vi "Drift Verification Konfig.vi"() -> ()   [LabVIEW 2020, in "EPA 1065.lvlib" / "Gas Analyzer Drift 1065-550.lvlib"]
uses:
  Gas Analyzer Drift 1065-550.lvlib
  Spaninlet Cluster.ctl
  Seiten/System Einstellungen V2/Konfig Gasflasche.ctl
  Seiten/System Einstellungen V2/Analysatoren.ctl
  Seiten/System Einstellungen V2/Gasflasche Auswahl.ctl
  T90 1065-308/Modus.ctl
  Komponentencluster.ctl
  Komponentenauswahl.ctl
  Drifttabelle.ctl
  Konfig Daten Drift Verification.ctl
  Anzeigecluster.ctl
  Chiller NO2 1065-376/Aktion FGV Drift Daten.ctl
  Aktion FGV Komponentenreferenz verwalten.ctl
  Sprachverwaltung/FGV Aktion Tabelle zerlegen.ctl
  Aktion Automatischer Ablauf Zustandsautomat.ctl
  Seiten/System Einstellungen V2/Aktion FGV Gasbottledefinition.ctl
  Seiten/FT-IR/FGV FT-IR Gasliste Aktionen.ctl
  Allgemeine VIs/Aktion Wertaenderung Gasliste.ctl
  Allgemeine VIs/Aktion Test Status.ctl
  Funktionstasten/Funktionstasten-Aktion.ctl
  Funktionstasten/Zustaende.ctl
  Allgemein/allgemeine Sub-VIs.lvlib
  Seiten/FT-IR/FT-IR.lvlib
  Funktionstasten/Funktionstasten.lvlib
  EPA 1065.lvlib
  Sprachverwaltung/Sprachverwaltung.lvlib
  Seiten/System Einstellungen V2/System Einstellungen V2.lvlib
  T90 1065-308/T90 Test 1065-308.lvlib
panel:
  in  "Systemeinstellung":bool
  in  "Gasliste geändert":bool
  in  "Registerkarte":T1(tab)
  in  "Pre Drift entsperren":bool caption="Test Start"
  in  "Pre Drift sperren":bool caption="Test Start"
  in  "Drift Konfig Daten":T2={"Bearbeiter:"="", "Pfad:"=path "D:/IAG_Data/Log", "Textname:"="", "CG Aufschaltzeit:"=120.0, "N2 Aufschaltzeit:"=120.0} caption="T90 Konfig Daten" {"N2 Aufschaltzeit:" min=10.0; "CG Aufschaltzeit:" min=10.0}
  in  "Speichern":bool
  in  "SpanRegister":T3(tab)
  in  "Span 1":T4={"Span Inlet Active"=FALSE, "Analysator"="FT-IR", "Konfig Gasflasche"=FALSE, "Gasflasche"=0, "Gasflaschen Nr.:"="", "Ablaufdatum"=timestamp(0 s since 1904-01-01), "Modus"=0, "Komponenten"={"Komponente 1"={"Komponente:"=0, "Konzentration IST"=0.0, "Einheit"=enum."ppm", "Genauigkeit"=0.0}, "Komponente 2"={"Komponente:"=0, "Konzentration IST"=0.0, "Einheit"=enum."ppm", "Genauigkeit"=0.0}, "Komponente 3"={"Komponente:"=0, "Konzentration IST"=0.0, "Einheit"=enum."ppm", "Genauigkeit"=0.0}, "Komponente 4"={"Komponente:"=0, "Konzentration IST"=0.0, "Einheit"=enum."ppm", "Genauigkeit"=0.0}, "Komponente 5"={"Komponente:"=0, "Konzentration IST"=0.0, "Einheit"=enum."ppm", "Genauigkeit"=0.0}}} {"Komponenten"."Komponente 5"."Komponente:" items=["---", "NO (3000) LP 191C", "NO2 (150) LP 191C (1of2)", "NO2 (2000) LP 191C (2of2)", "N2O (300) LP 191C (1of2)", "NH3 (300) LP 191C (1of2)", "NH3 (900,3000) LP 191C (2of2)", "HNCO (400) 191C", "H2O% (30) LP 191C", "Formaldehyde (70,500) LP 191C", "CO2 low% (4) LP 191C (2of2)", "CO2% (20) LP 191C (1of2)", "CO (700) LP 191C (1of3)", "CO% (1) LP 191C (2of3)", "Propylene (1000) LP 191C", "Aromatic HC C7 (500) LP 191C", "Ethylene (1000) LP 191C", "CH4 (250) LP 191C (1of2)", "CH4 (5000) LP 191C (2of2)", "Ethane (1000) LP 191C", "Acetylene (1000) LP 191C", "HNO2 (20) 191C", "MeOH (1000) 191C", "CO% (10) LP 191C (3of3)", "Formic Acid (100) 191C", "SO2 (500) LP 191C", "Acetaldehyde (1000) LP 191C", "COS (100) LP 191C", "1,3 butadiene (100) LP 191C", "Oil as Octane (200) LP 191C", "N2O (1000) LP 191C (2of2)", "Propane (200) LP 191C", "NO2 autorange (2000)", "CO autorange (100000)", "CH4 autorange (5000)", "NH3 autorange (3000)", "NOx autorange (3000)", "HCD (10000)", "NMHCD (10000)", "CO2% autorange (20)", "H2Oppm (300000)", "N2O autorange (1000)", "NMNEHCD (3000)", "Temp. Gascell", "Pressure Gascell", "sBeam@2500", "Temp. HL to FT-IR", "Temp. HL Extern SP1", "Outlet Temp FT-IR", "Temp. Cabinet", "Constant 0", "Constant 50", "Constant 100", "AK DUMMY"]; "Komponenten"."Komponente 5"."Konzentration IST" format="%#.4f"; "Komponenten"."Komponente 5"."Genauigkeit" format="%#.1f"; "Komponenten"."Komponente 4"."Komponente:" items=["---", "NO (3000) LP 191C", "NO2 (150) LP 191C (1of2)", "NO2 (2000) LP 191C (2of2)", "N2O (300) LP 191C (1of2)", "NH3 (300) LP 191C (1of2)", "NH3 (900,3000) LP 191C (2of2)", "HNCO (400) 191C", "H2O% (30) LP 191C", "Formaldehyde (70,500) LP 191C", "CO2 low% (4) LP 191C (2of2)", "CO2% (20) LP 191C (1of2)", "CO (700) LP 191C (1of3)", "CO% (1) LP 191C (2of3)", "Propylene (1000) LP 191C", "Aromatic HC C7 (500) LP 191C", "Ethylene (1000) LP 191C", "CH4 (250) LP 191C (1of2)", "CH4 (5000) LP 191C (2of2)", "Ethane (1000) LP 191C", "Acetylene (1000) LP 191C", "HNO2 (20) 191C", "MeOH (1000) 191C", "CO% (10) LP 191C (3of3)", "Formic Acid (100) 191C", "SO2 (500) LP 191C", "Acetaldehyde (1000) LP 191C", "COS (100) LP 191C", "1,3 butadiene (100) LP 191C", "Oil as Octane (200) LP 191C", "N2O (1000) LP 191C (2of2)", "Propane (200) LP 191C", "NO2 autorange (2000)", "CO autorange (100000)", "CH4 autorange (5000)", "NH3 autorange (3000)", "NOx autorange (3000)", "HCD (10000)", "NMHCD (10000)", "CO2% autorange (20)", "H2Oppm (300000)", "N2O autorange (1000)", "NMNEHCD (3000)", "Temp. Gascell", "Pressure Gascell", "sBeam@2500", "Temp. HL to FT-IR", "Temp. HL Extern SP1", "Outlet Temp FT-IR", "Temp. Cabinet", "Constant 0", "Constant 50", "Constant 100", "AK DUMMY"]; "Komponenten"."Komponente 4"."Konzentration IST" format="%#.4f"; "Komponenten"."Komponente 4"."Genauigkeit" format="%#.1f"; "Komponenten"."Komponente 3"."Komponente:" items=["---", "NO (3000) LP 191C", "NO2 (150) LP 191C (1of2)", "NO2 (2000) LP 191C (2of2)", "N2O (300) LP 191C (1of2)", "NH3 (300) LP 191C (1of2)", "NH3 (900,3000) LP 191C (2of2)", "HNCO (400) 191C", "H2O% (30) LP 191C", "Formaldehyde (70,500) LP 191C", "CO2 low% (4) LP 191C (2of2)", "CO2% (20) LP 191C (1of2)", "CO (700) LP 191C (1of3)", "CO% (1) LP 191C (2of3)", "Propylene (1000) LP 191C", "Aromatic HC C7 (500) LP 191C", "Ethylene (1000) LP 191C", "CH4 (250) LP 191C (1of2)", "CH4 (5000) LP 191C (2of2)", "Ethane (1000) LP 191C", "Acetylene (1000) LP 191C", "HNO2 (20) 191C", "MeOH (1000) 191C", "CO% (10) LP 191C (3of3)", "Formic Acid (100) 191C", "SO2 (500) LP 191C", "Acetaldehyde (1000) LP 191C", "COS (100) LP 191C", "1,3 butadiene (100) LP 191C", "Oil as Octane (200) LP 191C", "N2O (1000) LP 191C (2of2)", "Propane (200) LP 191C", "NO2 autorange (2000)", "CO autorange (100000)", "CH4 autorange (5000)", "NH3 autorange (3000)", "NOx autorange (3000)", "HCD (10000)", "NMHCD (10000)", "CO2% autorange (20)", "H2Oppm (300000)", "N2O autorange (1000)", "NMNEHCD (3000)", "Temp. Gascell", "Pressure Gascell", "sBeam@2500", "Temp. HL to FT-IR", "Temp. HL Extern SP1", "Outlet Temp FT-IR", "Temp. Cabinet", "Constant 0", "Constant 50", "Constant 100", "AK DUMMY"]; "Komponenten"."Komponente 3"."Konzentration IST" format="%#.4f"; "Komponenten"."Komponente 3"."Genauigkeit" format="%#.1f"; "Komponenten"."Komponente 2"."Komponente:" items=["---", "NO (3000) LP 191C", "NO2 (150) LP 191C (1of2)", "NO2 (2000) LP 191C (2of2)", "N2O (300) LP 191C (1of2)", "NH3 (300) LP 191C (1of2)", "NH3 (900,3000) LP 191C (2of2)", "HNCO (400) 191C", "H2O% (30) LP 191C", "Formaldehyde (70,500) LP 191C", "CO2 low% (4) LP 191C (2of2)", "CO2% (20) LP 191C (1of2)", "CO (700) LP 191C (1of3)", "CO% (1) LP 191C (2of3)", "Propylene (1000) LP 191C", "Aromatic HC C7 (500) LP 191C", "Ethylene (1000) LP 191C", "CH4 (250) LP 191C (1of2)", "CH4 (5000) LP 191C (2of2)", "Ethane (1000) LP 191C", "Acetylene (1000) LP 191C", "HNO2 (20) 191C", "MeOH (1000) 191C", "CO% (10) LP 191C (3of3)", "Formic Acid (100) 191C", "SO2 (500) LP 191C", "Acetaldehyde (1000) LP 191C", "COS (100) LP 191C", "1,3 butadiene (100) LP 191C", "Oil as Octane (200) LP 191C", "N2O (1000) LP 191C (2of2)", "Propane (200) LP 191C", "NO2 autorange (2000)", "CO autorange (100000)", "CH4 autorange (5000)", "NH3 autorange (3000)", "NOx autorange (3000)", "HCD (10000)", "NMHCD (10000)", "CO2% autorange (20)", "H2Oppm (300000)", "N2O autorange (1000)", "NMNEHCD (3000)", "Temp. Gascell", "Pressure Gascell", "sBeam@2500", "Temp. HL to FT-IR", "Temp. HL Extern SP1", "Outlet Temp FT-IR", "Temp. Cabinet", "Constant 0", "Constant 50", "Constant 100", "AK DUMMY"]; "Komponenten"."Komponente 2"."Konzentration IST" format="%#.4f"; "Komponenten"."Komponente 2"."Genauigkeit" format="%#.1f"; "Komponenten"."Komponente 1"."Komponente:" items=["---", "NO (3000) LP 191C", "NO2 (150) LP 191C (1of2)", "NO2 (2000) LP 191C (2of2)", "N2O (300) LP 191C (1of2)", "NH3 (300) LP 191C (1of2)", "NH3 (900,3000) LP 191C (2of2)", "HNCO (400) 191C", "H2O% (30) LP 191C", "Formaldehyde (70,500) LP 191C", "CO2 low% (4) LP 191C (2of2)", "CO2% (20) LP 191C (1of2)", "CO (700) LP 191C (1of3)", "CO% (1) LP 191C (2of3)", "Propylene (1000) LP 191C", "Aromatic HC C7 (500) LP 191C", "Ethylene (1000) LP 191C", "CH4 (250) LP 191C (1of2)", "CH4 (5000) LP 191C (2of2)", "Ethane (1000) LP 191C", "Acetylene (1000) LP 191C", "HNO2 (20) 191C", "MeOH (1000) 191C", "CO% (10) LP 191C (3of3)", "Formic Acid (100) 191C", "SO2 (500) LP 191C", "Acetaldehyde (1000) LP 191C", "COS (100) LP 191C", "1,3 butadiene (100) LP 191C", "Oil as Octane (200) LP 191C", "N2O (1000) LP 191C (2of2)", "Propane (200) LP 191C", "NO2 autorange (2000)", "CO autorange (100000)", "CH4 autorange (5000)", "NH3 autorange (3000)", "NOx autorange (3000)", "HCD (10000)", "NMHCD (10000)", "CO2% autorange (20)", "H2Oppm (300000)", "N2O autorange (1000)", "NMNEHCD (3000)", "Temp. Gascell", "Pressure Gascell", "sBeam@2500", "Temp. HL to FT-IR", "Temp. HL Extern SP1", "Outlet Temp FT-IR", "Temp. Cabinet", "Constant 0", "Constant 50", "Constant 100", "AK DUMMY"]; "Komponenten"."Komponente 1"."Konzentration IST" format="%#.4f"; "Komponenten"."Komponente 1"."Genauigkeit" format="%#.1f"; "Modus" items=["CG zu PNS", "CG zu Entnahmestelle"]; "Ablaufdatum" format="%<%d.%m.%Y>T"; "Gasflasche" items=["----"=10000, "IAG O2"=0, "IAG C2H2"=1, "IAG C2H4"=2, "IAG NH3 200"=3, "IAG NH3 2000"=4, "IAG NH3 3000"=5, "IAG CO 5%"=6, "IAG Propane 2%"=7, "IAG NO 1000"=8, "IAG SO2"=9, "IAG C3H6"=10, "IAG CO2"=11, "IAG CO"=12, "IAG N2O"=13, "IAG N2O 100"=14, "IAG NO2 1000"=15, "IAG NO2 100"=16, "IAG CH4"=17, "IAG Propane"=18, "IAG NO 5000"=19, "Hansi"=20, "IAG MG"=21]}
  in  "Span 2":T4={"Span Inlet Active"=FALSE, "Analysator"="FT-IR", "Konfig Gasflasche"=FALSE, "Gasflasche"=0, "Gasflaschen Nr.:"="", "Ablaufdatum"=timestamp(0 s since 1904-01-01), "Modus"=0, "Komponenten"={"Komponente 1"={"Komponente:"=0, "Konzentration IST"=0.0, "Einheit"=enum."ppm", "Genauigkeit"=0.0}, "Komponente 2"={"Komponente:"=0, "Konzentration IST"=0.0, "Einheit"=enum."ppm", "Genauigkeit"=0.0}, "Komponente 3"={"Komponente:"=0, "Konzentration IST"=0.0, "Einheit"=enum."ppm", "Genauigkeit"=0.0}, "Komponente 4"={"Komponente:"=0, "Konzentration IST"=0.0, "Einheit"=enum."ppm", "Genauigkeit"=0.0}, "Komponente 5"={"Komponente:"=0, "Konzentration IST"=0.0, "Einheit"=enum."ppm", "Genauigkeit"=0.0}}} {"Komponenten"."Komponente 5"."Komponente:" items=["---", "NO (3000) LP 191C", "NO2 (150) LP 191C (1of2)", "NO2 (2000) LP 191C (2of2)", "N2O (300) LP 191C (1of2)", "NH3 (300) LP 191C (1of2)", "NH3 (900,3000) LP 191C (2of2)", "HNCO (400) 191C", "H2O% (30) LP 191C", "Formaldehyde (70,500) LP 191C", "CO2 low% (4) LP 191C (2of2)", "CO2% (20) LP 191C (1of2)", "CO (700) LP 191C (1of3)", "CO% (1) LP 191C (2of3)", "Propylene (1000) LP 191C", "Aromatic HC C7 (500) LP 191C", "Ethylene (1000) LP 191C", "CH4 (250) LP 191C (1of2)", "CH4 (5000) LP 191C (2of2)", "Ethane (1000) LP 191C", "Acetylene (1000) LP 191C", "HNO2 (20) 191C", "MeOH (1000) 191C", "CO% (10) LP 191C (3of3)", "Formic Acid (100) 191C", "SO2 (500) LP 191C", "Acetaldehyde (1000) LP 191C", "COS (100) LP 191C", "1,3 butadiene (100) LP 191C", "Oil as Octane (200) LP 191C", "N2O (1000) LP 191C (2of2)", "Propane (200) LP 191C", "NO2 autorange (2000)", "CO autorange (100000)", "CH4 autorange (5000)", "NH3 autorange (3000)", "NOx autorange (3000)", "HCD (10000)", "NMHCD (10000)", "CO2% autorange (20)", "H2Oppm (300000)", "N2O autorange (1000)", "NMNEHCD (3000)", "Temp. Gascell", "Pressure Gascell", "sBeam@2500", "Temp. HL to FT-IR", "Temp. HL Extern SP1", "Outlet Temp FT-IR", "Temp. Cabinet", "Constant 0", "Constant 50", "Constant 100", "AK DUMMY"]; "Komponenten"."Komponente 5"."Konzentration IST" format="%#.4f"; "Komponenten"."Komponente 5"."Genauigkeit" format="%#.1f"; "Komponenten"."Komponente 4"."Komponente:" items=["---", "NO (3000) LP 191C", "NO2 (150) LP 191C (1of2)", "NO2 (2000) LP 191C (2of2)", "N2O (300) LP 191C (1of2)", "NH3 (300) LP 191C (1of2)", "NH3 (900,3000) LP 191C (2of2)", "HNCO (400) 191C", "H2O% (30) LP 191C", "Formaldehyde (70,500) LP 191C", "CO2 low% (4) LP 191C (2of2)", "CO2% (20) LP 191C (1of2)", "CO (700) LP 191C (1of3)", "CO% (1) LP 191C (2of3)", "Propylene (1000) LP 191C", "Aromatic HC C7 (500) LP 191C", "Ethylene (1000) LP 191C", "CH4 (250) LP 191C (1of2)", "CH4 (5000) LP 191C (2of2)", "Ethane (1000) LP 191C", "Acetylene (1000) LP 191C", "HNO2 (20) 191C", "MeOH (1000) 191C", "CO% (10) LP 191C (3of3)", "Formic Acid (100) 191C", "SO2 (500) LP 191C", "Acetaldehyde (1000) LP 191C", "COS (100) LP 191C", "1,3 butadiene (100) LP 191C", "Oil as Octane (200) LP 191C", "N2O (1000) LP 191C (2of2)", "Propane (200) LP 191C", "NO2 autorange (2000)", "CO autorange (100000)", "CH4 autorange (5000)", "NH3 autorange (3000)", "NOx autorange (3000)", "HCD (10000)", "NMHCD (10000)", "CO2% autorange (20)", "H2Oppm (300000)", "N2O autorange (1000)", "NMNEHCD (3000)", "Temp. Gascell", "Pressure Gascell", "sBeam@2500", "Temp. HL to FT-IR", "Temp. HL Extern SP1", "Outlet Temp FT-IR", "Temp. Cabinet", "Constant 0", "Constant 50", "Constant 100", "AK DUMMY"]; "Komponenten"."Komponente 4"."Konzentration IST" format="%#.4f"; "Komponenten"."Komponente 4"."Genauigkeit" format="%#.1f"; "Komponenten"."Komponente 3"."Komponente:" items=["---", "NO (3000) LP 191C", "NO2 (150) LP 191C (1of2)", "NO2 (2000) LP 191C (2of2)", "N2O (300) LP 191C (1of2)", "NH3 (300) LP 191C (1of2)", "NH3 (900,3000) LP 191C (2of2)", "HNCO (400) 191C", "H2O% (30) LP 191C", "Formaldehyde (70,500) LP 191C", "CO2 low% (4) LP 191C (2of2)", "CO2% (20) LP 191C (1of2)", "CO (700) LP 191C (1of3)", "CO% (1) LP 191C (2of3)", "Propylene (1000) LP 191C", "Aromatic HC C7 (500) LP 191C", "Ethylene (1000) LP 191C", "CH4 (250) LP 191C (1of2)", "CH4 (5000) LP 191C (2of2)", "Ethane (1000) LP 191C", "Acetylene (1000) LP 191C", "HNO2 (20) 191C", "MeOH (1000) 191C", "CO% (10) LP 191C (3of3)", "Formic Acid (100) 191C", "SO2 (500) LP 191C", "Acetaldehyde (1000) LP 191C", "COS (100) LP 191C", "1,3 butadiene (100) LP 191C", "Oil as Octane (200) LP 191C", "N2O (1000) LP 191C (2of2)", "Propane (200) LP 191C", "NO2 autorange (2000)", "CO autorange (100000)", "CH4 autorange (5000)", "NH3 autorange (3000)", "NOx autorange (3000)", "HCD (10000)", "NMHCD (10000)", "CO2% autorange (20)", "H2Oppm (300000)", "N2O autorange (1000)", "NMNEHCD (3000)", "Temp. Gascell", "Pressure Gascell", "sBeam@2500", "Temp. HL to FT-IR", "Temp. HL Extern SP1", "Outlet Temp FT-IR", "Temp. Cabinet", "Constant 0", "Constant 50", "Constant 100", "AK DUMMY"]; "Komponenten"."Komponente 3"."Konzentration IST" format="%#.4f"; "Komponenten"."Komponente 3"."Genauigkeit" format="%#.1f"; "Komponenten"."Komponente 2"."Komponente:" items=["---", "NO (3000) LP 191C", "NO2 (150) LP 191C (1of2)", "NO2 (2000) LP 191C (2of2)", "N2O (300) LP 191C (1of2)", "NH3 (300) LP 191C (1of2)", "NH3 (900,3000) LP 191C (2of2)", "HNCO (400) 191C", "H2O% (30) LP 191C", "Formaldehyde (70,500) LP 191C", "CO2 low% (4) LP 191C (2of2)", "CO2% (20) LP 191C (1of2)", "CO (700) LP 191C (1of3)", "CO% (1) LP 191C (2of3)", "Propylene (1000) LP 191C", "Aromatic HC C7 (500) LP 191C", "Ethylene (1000) LP 191C", "CH4 (250) LP 191C (1of2)", "CH4 (5000) LP 191C (2of2)", "Ethane (1000) LP 191C", "Acetylene (1000) LP 191C", "HNO2 (20) 191C", "MeOH (1000) 191C", "CO% (10) LP 191C (3of3)", "Formic Acid (100) 191C", "SO2 (500) LP 191C", "Acetaldehyde (1000) LP 191C", "COS (100) LP 191C", "1,3 butadiene (100) LP 191C", "Oil as Octane (200) LP 191C", "N2O (1000) LP 191C (2of2)", "Propane (200) LP 191C", "NO2 autorange (2000)", "CO autorange (100000)", "CH4 autorange (5000)", "NH3 autorange (3000)", "NOx autorange (3000)", "HCD (10000)", "NMHCD (10000)", "CO2% autorange (20)", "H2Oppm (300000)", "N2O autorange (1000)", "NMNEHCD (3000)", "Temp. Gascell", "Pressure Gascell", "sBeam@2500", "Temp. HL to FT-IR", "Temp. HL Extern SP1", "Outlet Temp FT-IR", "Temp. Cabinet", "Constant 0", "Constant 50", "Constant 100", "AK DUMMY"]; "Komponenten"."Komponente 2"."Konzentration IST" format="%#.4f"; "Komponenten"."Komponente 2"."Genauigkeit" format="%#.1f"; "Komponenten"."Komponente 1"."Komponente:" items=["---", "NO (3000) LP 191C", "NO2 (150) LP 191C (1of2)", "NO2 (2000) LP 191C (2of2)", "N2O (300) LP 191C (1of2)", "NH3 (300) LP 191C (1of2)", "NH3 (900,3000) LP 191C (2of2)", "HNCO (400) 191C", "H2O% (30) LP 191C", "Formaldehyde (70,500) LP 191C", "CO2 low% (4) LP 191C (2of2)", "CO2% (20) LP 191C (1of2)", "CO (700) LP 191C (1of3)", "CO% (1) LP 191C (2of3)", "Propylene (1000) LP 191C", "Aromatic HC C7 (500) LP 191C", "Ethylene (1000) LP 191C", "CH4 (250) LP 191C (1of2)", "CH4 (5000) LP 191C (2of2)", "Ethane (1000) LP 191C", "Acetylene (1000) LP 191C", "HNO2 (20) 191C", "MeOH (1000) 191C", "CO% (10) LP 191C (3of3)", "Formic Acid (100) 191C", "SO2 (500) LP 191C", "Acetaldehyde (1000) LP 191C", "COS (100) LP 191C", "1,3 butadiene (100) LP 191C", "Oil as Octane (200) LP 191C", "N2O (1000) LP 191C (2of2)", "Propane (200) LP 191C", "NO2 autorange (2000)", "CO autorange (100000)", "CH4 autorange (5000)", "NH3 autorange (3000)", "NOx autorange (3000)", "HCD (10000)", "NMHCD (10000)", "CO2% autorange (20)", "H2Oppm (300000)", "N2O autorange (1000)", "NMNEHCD (3000)", "Temp. Gascell", "Pressure Gascell", "sBeam@2500", "Temp. HL to FT-IR", "Temp. HL Extern SP1", "Outlet Temp FT-IR", "Temp. Cabinet", "Constant 0", "Constant 50", "Constant 100", "AK DUMMY"]; "Komponenten"."Komponente 1"."Konzentration IST" format="%#.4f"; "Komponenten"."Komponente 1"."Genauigkeit" format="%#.1f"; "Modus" items=["CG zu PNS", "CG zu Entnahmestelle"]; "Ablaufdatum" format="%<%d.%m.%Y>T"; "Gasflasche" items=["----"=10000, "IAG O2"=0, "IAG C2H2"=1, "IAG C2H4"=2, "IAG NH3 200"=3, "IAG NH3 2000"=4, "IAG NH3 3000"=5, "IAG CO 5%"=6, "IAG Propane 2%"=7, "IAG NO 1000"=8, "IAG SO2"=9, "IAG C3H6"=10, "IAG CO2"=11, "IAG CO"=12, "IAG N2O"=13, "IAG N2O 100"=14, "IAG NO2 1000"=15, "IAG NO2 100"=16, "IAG CH4"=17, "IAG Propane"=18, "IAG NO 5000"=19, "Hansi"=20, "IAG MG"=21]}
  in  "Span 3":T4={"Span Inlet Active"=FALSE, "Analysator"="FT-IR", "Konfig Gasflasche"=FALSE, "Gasflasche"=0, "Gasflaschen Nr.:"="", "Ablaufdatum"=timestamp(0 s since 1904-01-01), "Modus"=0, "Komponenten"={"Komponente 1"={"Komponente:"=0, "Konzentration IST"=0.0, "Einheit"=enum."ppm", "Genauigkeit"=0.0}, "Komponente 2"={"Komponente:"=0, "Konzentration IST"=0.0, "Einheit"=enum."ppm", "Genauigkeit"=0.0}, "Komponente 3"={"Komponente:"=0, "Konzentration IST"=0.0, "Einheit"=enum."ppm", "Genauigkeit"=0.0}, "Komponente 4"={"Komponente:"=0, "Konzentration IST"=0.0, "Einheit"=enum."ppm", "Genauigkeit"=0.0}, "Komponente 5"={"Komponente:"=0, "Konzentration IST"=0.0, "Einheit"=enum."ppm", "Genauigkeit"=0.0}}} {"Komponenten"."Komponente 5"."Komponente:" items=["---", "NO (3000) LP 191C", "NO2 (150) LP 191C (1of2)", "NO2 (2000) LP 191C (2of2)", "N2O (300) LP 191C (1of2)", "NH3 (300) LP 191C (1of2)", "NH3 (900,3000) LP 191C (2of2)", "HNCO (400) 191C", "H2O% (30) LP 191C", "Formaldehyde (70,500) LP 191C", "CO2 low% (4) LP 191C (2of2)", "CO2% (20) LP 191C (1of2)", "CO (700) LP 191C (1of3)", "CO% (1) LP 191C (2of3)", "Propylene (1000) LP 191C", "Aromatic HC C7 (500) LP 191C", "Ethylene (1000) LP 191C", "CH4 (250) LP 191C (1of2)", "CH4 (5000) LP 191C (2of2)", "Ethane (1000) LP 191C", "Acetylene (1000) LP 191C", "HNO2 (20) 191C", "MeOH (1000) 191C", "CO% (10) LP 191C (3of3)", "Formic Acid (100) 191C", "SO2 (500) LP 191C", "Acetaldehyde (1000) LP 191C", "COS (100) LP 191C", "1,3 butadiene (100) LP 191C", "Oil as Octane (200) LP 191C", "N2O (1000) LP 191C (2of2)", "Propane (200) LP 191C", "NO2 autorange (2000)", "CO autorange (100000)", "CH4 autorange (5000)", "NH3 autorange (3000)", "NOx autorange (3000)", "HCD (10000)", "NMHCD (10000)", "CO2% autorange (20)", "H2Oppm (300000)", "N2O autorange (1000)", "NMNEHCD (3000)", "Temp. Gascell", "Pressure Gascell", "sBeam@2500", "Temp. HL to FT-IR", "Temp. HL Extern SP1", "Outlet Temp FT-IR", "Temp. Cabinet", "Constant 0", "Constant 50", "Constant 100", "AK DUMMY"]; "Komponenten"."Komponente 5"."Konzentration IST" format="%#.4f"; "Komponenten"."Komponente 5"."Genauigkeit" format="%#.1f"; "Komponenten"."Komponente 4"."Komponente:" items=["---", "NO (3000) LP 191C", "NO2 (150) LP 191C (1of2)", "NO2 (2000) LP 191C (2of2)", "N2O (300) LP 191C (1of2)", "NH3 (300) LP 191C (1of2)", "NH3 (900,3000) LP 191C (2of2)", "HNCO (400) 191C", "H2O% (30) LP 191C", "Formaldehyde (70,500) LP 191C", "CO2 low% (4) LP 191C (2of2)", "CO2% (20) LP 191C (1of2)", "CO (700) LP 191C (1of3)", "CO% (1) LP 191C (2of3)", "Propylene (1000) LP 191C", "Aromatic HC C7 (500) LP 191C", "Ethylene (1000) LP 191C", "CH4 (250) LP 191C (1of2)", "CH4 (5000) LP 191C (2of2)", "Ethane (1000) LP 191C", "Acetylene (1000) LP 191C", "HNO2 (20) 191C", "MeOH (1000) 191C", "CO% (10) LP 191C (3of3)", "Formic Acid (100) 191C", "SO2 (500) LP 191C", "Acetaldehyde (1000) LP 191C", "COS (100) LP 191C", "1,3 butadiene (100) LP 191C", "Oil as Octane (200) LP 191C", "N2O (1000) LP 191C (2of2)", "Propane (200) LP 191C", "NO2 autorange (2000)", "CO autorange (100000)", "CH4 autorange (5000)", "NH3 autorange (3000)", "NOx autorange (3000)", "HCD (10000)", "NMHCD (10000)", "CO2% autorange (20)", "H2Oppm (300000)", "N2O autorange (1000)", "NMNEHCD (3000)", "Temp. Gascell", "Pressure Gascell", "sBeam@2500", "Temp. HL to FT-IR", "Temp. HL Extern SP1", "Outlet Temp FT-IR", "Temp. Cabinet", "Constant 0", "Constant 50", "Constant 100", "AK DUMMY"]; "Komponenten"."Komponente 4"."Konzentration IST" format="%#.4f"; "Komponenten"."Komponente 4"."Genauigkeit" format="%#.1f"; "Komponenten"."Komponente 3"."Komponente:" items=["---", "NO (3000) LP 191C", "NO2 (150) LP 191C (1of2)", "NO2 (2000) LP 191C (2of2)", "N2O (300) LP 191C (1of2)", "NH3 (300) LP 191C (1of2)", "NH3 (900,3000) LP 191C (2of2)", "HNCO (400) 191C", "H2O% (30) LP 191C", "Formaldehyde (70,500) LP 191C", "CO2 low% (4) LP 191C (2of2)", "CO2% (20) LP 191C (1of2)", "CO (700) LP 191C (1of3)", "CO% (1) LP 191C (2of3)", "Propylene (1000) LP 191C", "Aromatic HC C7 (500) LP 191C", "Ethylene (1000) LP 191C", "CH4 (250) LP 191C (1of2)", "CH4 (5000) LP 191C (2of2)", "Ethane (1000) LP 191C", "Acetylene (1000) LP 191C", "HNO2 (20) 191C", "MeOH (1000) 191C", "CO% (10) LP 191C (3of3)", "Formic Acid (100) 191C", "SO2 (500) LP 191C", "Acetaldehyde (1000) LP 191C", "COS (100) LP 191C", "1,3 butadiene (100) LP 191C", "Oil as Octane (200) LP 191C", "N2O (1000) LP 191C (2of2)", "Propane (200) LP 191C", "NO2 autorange (2000)", "CO autorange (100000)", "CH4 autorange (5000)", "NH3 autorange (3000)", "NOx autorange (3000)", "HCD (10000)", "NMHCD (10000)", "CO2% autorange (20)", "H2Oppm (300000)", "N2O autorange (1000)", "NMNEHCD (3000)", "Temp. Gascell", "Pressure Gascell", "sBeam@2500", "Temp. HL to FT-IR", "Temp. HL Extern SP1", "Outlet Temp FT-IR", "Temp. Cabinet", "Constant 0", "Constant 50", "Constant 100", "AK DUMMY"]; "Komponenten"."Komponente 3"."Konzentration IST" format="%#.4f"; "Komponenten"."Komponente 3"."Genauigkeit" format="%#.1f"; "Komponenten"."Komponente 2"."Komponente:" items=["---", "NO (3000) LP 191C", "NO2 (150) LP 191C (1of2)", "NO2 (2000) LP 191C (2of2)", "N2O (300) LP 191C (1of2)", "NH3 (300) LP 191C (1of2)", "NH3 (900,3000) LP 191C (2of2)", "HNCO (400) 191C", "H2O% (30) LP 191C", "Formaldehyde (70,500) LP 191C", "CO2 low% (4) LP 191C (2of2)", "CO2% (20) LP 191C (1of2)", "CO (700) LP 191C (1of3)", "CO% (1) LP 191C (2of3)", "Propylene (1000) LP 191C", "Aromatic HC C7 (500) LP 191C", "Ethylene (1000) LP 191C", "CH4 (250) LP 191C (1of2)", "CH4 (5000) LP 191C (2of2)", "Ethane (1000) LP 191C", "Acetylene (1000) LP 191C", "HNO2 (20) 191C", "MeOH (1000) 191C", "CO% (10) LP 191C (3of3)", "Formic Acid (100) 191C", "SO2 (500) LP 191C", "Acetaldehyde (1000) LP 191C", "COS (100) LP 191C", "1,3 butadiene (100) LP 191C", "Oil as Octane (200) LP 191C", "N2O (1000) LP 191C (2of2)", "Propane (200) LP 191C", "NO2 autorange (2000)", "CO autorange (100000)", "CH4 autorange (5000)", "NH3 autorange (3000)", "NOx autorange (3000)", "HCD (10000)", "NMHCD (10000)", "CO2% autorange (20)", "H2Oppm (300000)", "N2O autorange (1000)", "NMNEHCD (3000)", "Temp. Gascell", "Pressure Gascell", "sBeam@2500", "Temp. HL to FT-IR", "Temp. HL Extern SP1", "Outlet Temp FT-IR", "Temp. Cabinet", "Constant 0", "Constant 50", "Constant 100", "AK DUMMY"]; "Komponenten"."Komponente 2"."Konzentration IST" format="%#.4f"; "Komponenten"."Komponente 2"."Genauigkeit" format="%#.1f"; "Komponenten"."Komponente 1"."Komponente:" items=["---", "NO (3000) LP 191C", "NO2 (150) LP 191C (1of2)", "NO2 (2000) LP 191C (2of2)", "N2O (300) LP 191C (1of2)", "NH3 (300) LP 191C (1of2)", "NH3 (900,3000) LP 191C (2of2)", "HNCO (400) 191C", "H2O% (30) LP 191C", "Formaldehyde (70,500) LP 191C", "CO2 low% (4) LP 191C (2of2)", "CO2% (20) LP 191C (1of2)", "CO (700) LP 191C (1of3)", "CO% (1) LP 191C (2of3)", "Propylene (1000) LP 191C", "Aromatic HC C7 (500) LP 191C", "Ethylene (1000) LP 191C", "CH4 (250) LP 191C (1of2)", "CH4 (5000) LP 191C (2of2)", "Ethane (1000) LP 191C", "Acetylene (1000) LP 191C", "HNO2 (20) 191C", "MeOH (1000) 191C", "CO% (10) LP 191C (3of3)", "Formic Acid (100) 191C", "SO2 (500) LP 191C", "Acetaldehyde (1000) LP 191C", "COS (100) LP 191C", "1,3 butadiene (100) LP 191C", "Oil as Octane (200) LP 191C", "N2O (1000) LP 191C (2of2)", "Propane (200) LP 191C", "NO2 autorange (2000)", "CO autorange (100000)", "CH4 autorange (5000)", "NH3 autorange (3000)", "NOx autorange (3000)", "HCD (10000)", "NMHCD (10000)", "CO2% autorange (20)", "H2Oppm (300000)", "N2O autorange (1000)", "NMNEHCD (3000)", "Temp. Gascell", "Pressure Gascell", "sBeam@2500", "Temp. HL to FT-IR", "Temp. HL Extern SP1", "Outlet Temp FT-IR", "Temp. Cabinet", "Constant 0", "Constant 50", "Constant 100", "AK DUMMY"]; "Komponenten"."Komponente 1"."Konzentration IST" format="%#.4f"; "Komponenten"."Komponente 1"."Genauigkeit" format="%#.1f"; "Modus" items=["CG zu PNS", "CG zu Entnahmestelle"]; "Ablaufdatum" format="%<%d.%m.%Y>T"; "Gasflasche" items=["----"=10000, "IAG O2"=0, "IAG C2H2"=1, "IAG C2H4"=2, "IAG NH3 200"=3, "IAG NH3 2000"=4, "IAG NH3 3000"=5, "IAG CO 5%"=6, "IAG Propane 2%"=7, "IAG NO 1000"=8, "IAG SO2"=9, "IAG C3H6"=10, "IAG CO2"=11, "IAG CO"=12, "IAG N2O"=13, "IAG N2O 100"=14, "IAG NO2 1000"=15, "IAG NO2 100"=16, "IAG CH4"=17, "IAG Propane"=18, "IAG NO 5000"=19, "Hansi"=20, "IAG MG"=21]}
  in  "Span 4":T4={"Span Inlet Active"=FALSE, "Analysator"="FT-IR", "Konfig Gasflasche"=FALSE, "Gasflasche"=0, "Gasflaschen Nr.:"="", "Ablaufdatum"=timestamp(0 s since 1904-01-01), "Modus"=0, "Komponenten"={"Komponente 1"={"Komponente:"=0, "Konzentration IST"=0.0, "Einheit"=enum."ppm", "Genauigkeit"=0.0}, "Komponente 2"={"Komponente:"=0, "Konzentration IST"=0.0, "Einheit"=enum."ppm", "Genauigkeit"=0.0}, "Komponente 3"={"Komponente:"=0, "Konzentration IST"=0.0, "Einheit"=enum."ppm", "Genauigkeit"=0.0}, "Komponente 4"={"Komponente:"=0, "Konzentration IST"=0.0, "Einheit"=enum."ppm", "Genauigkeit"=0.0}, "Komponente 5"={"Komponente:"=0, "Konzentration IST"=0.0, "Einheit"=enum."ppm", "Genauigkeit"=0.0}}} {"Komponenten"."Komponente 5"."Komponente:" items=["---", "NO (3000) LP 191C", "NO2 (150) LP 191C (1of2)", "NO2 (2000) LP 191C (2of2)", "N2O (300) LP 191C (1of2)", "NH3 (300) LP 191C (1of2)", "NH3 (900,3000) LP 191C (2of2)", "HNCO (400) 191C", "H2O% (30) LP 191C", "Formaldehyde (70,500) LP 191C", "CO2 low% (4) LP 191C (2of2)", "CO2% (20) LP 191C (1of2)", "CO (700) LP 191C (1of3)", "CO% (1) LP 191C (2of3)", "Propylene (1000) LP 191C", "Aromatic HC C7 (500) LP 191C", "Ethylene (1000) LP 191C", "CH4 (250) LP 191C (1of2)", "CH4 (5000) LP 191C (2of2)", "Ethane (1000) LP 191C", "Acetylene (1000) LP 191C", "HNO2 (20) 191C", "MeOH (1000) 191C", "CO% (10) LP 191C (3of3)", "Formic Acid (100) 191C", "SO2 (500) LP 191C", "Acetaldehyde (1000) LP 191C", "COS (100) LP 191C", "1,3 butadiene (100) LP 191C", "Oil as Octane (200) LP 191C", "N2O (1000) LP 191C (2of2)", "Propane (200) LP 191C", "NO2 autorange (2000)", "CO autorange (100000)", "CH4 autorange (5000)", "NH3 autorange (3000)", "NOx autorange (3000)", "HCD (10000)", "NMHCD (10000)", "CO2% autorange (20)", "H2Oppm (300000)", "N2O autorange (1000)", "NMNEHCD (3000)", "Temp. Gascell", "Pressure Gascell", "sBeam@2500", "Temp. HL to FT-IR", "Temp. HL Extern SP1", "Outlet Temp FT-IR", "Temp. Cabinet", "Constant 0", "Constant 50", "Constant 100", "AK DUMMY"]; "Komponenten"."Komponente 5"."Konzentration IST" format="%#.4f"; "Komponenten"."Komponente 5"."Genauigkeit" format="%#.1f"; "Komponenten"."Komponente 4"."Komponente:" items=["---", "NO (3000) LP 191C", "NO2 (150) LP 191C (1of2)", "NO2 (2000) LP 191C (2of2)", "N2O (300) LP 191C (1of2)", "NH3 (300) LP 191C (1of2)", "NH3 (900,3000) LP 191C (2of2)", "HNCO (400) 191C", "H2O% (30) LP 191C", "Formaldehyde (70,500) LP 191C", "CO2 low% (4) LP 191C (2of2)", "CO2% (20) LP 191C (1of2)", "CO (700) LP 191C (1of3)", "CO% (1) LP 191C (2of3)", "Propylene (1000) LP 191C", "Aromatic HC C7 (500) LP 191C", "Ethylene (1000) LP 191C", "CH4 (250) LP 191C (1of2)", "CH4 (5000) LP 191C (2of2)", "Ethane (1000) LP 191C", "Acetylene (1000) LP 191C", "HNO2 (20) 191C", "MeOH (1000) 191C", "CO% (10) LP 191C (3of3)", "Formic Acid (100) 191C", "SO2 (500) LP 191C", "Acetaldehyde (1000) LP 191C", "COS (100) LP 191C", "1,3 butadiene (100) LP 191C", "Oil as Octane (200) LP 191C", "N2O (1000) LP 191C (2of2)", "Propane (200) LP 191C", "NO2 autorange (2000)", "CO autorange (100000)", "CH4 autorange (5000)", "NH3 autorange (3000)", "NOx autorange (3000)", "HCD (10000)", "NMHCD (10000)", "CO2% autorange (20)", "H2Oppm (300000)", "N2O autorange (1000)", "NMNEHCD (3000)", "Temp. Gascell", "Pressure Gascell", "sBeam@2500", "Temp. HL to FT-IR", "Temp. HL Extern SP1", "Outlet Temp FT-IR", "Temp. Cabinet", "Constant 0", "Constant 50", "Constant 100", "AK DUMMY"]; "Komponenten"."Komponente 4"."Konzentration IST" format="%#.4f"; "Komponenten"."Komponente 4"."Genauigkeit" format="%#.1f"; "Komponenten"."Komponente 3"."Komponente:" items=["---", "NO (3000) LP 191C", "NO2 (150) LP 191C (1of2)", "NO2 (2000) LP 191C (2of2)", "N2O (300) LP 191C (1of2)", "NH3 (300) LP 191C (1of2)", "NH3 (900,3000) LP 191C (2of2)", "HNCO (400) 191C", "H2O% (30) LP 191C", "Formaldehyde (70,500) LP 191C", "CO2 low% (4) LP 191C (2of2)", "CO2% (20) LP 191C (1of2)", "CO (700) LP 191C (1of3)", "CO% (1) LP 191C (2of3)", "Propylene (1000) LP 191C", "Aromatic HC C7 (500) LP 191C", "Ethylene (1000) LP 191C", "CH4 (250) LP 191C (1of2)", "CH4 (5000) LP 191C (2of2)", "Ethane (1000) LP 191C", "Acetylene (1000) LP 191C", "HNO2 (20) 191C", "MeOH (1000) 191C", "CO% (10) LP 191C (3of3)", "Formic Acid (100) 191C", "SO2 (500) LP 191C", "Acetaldehyde (1000) LP 191C", "COS (100) LP 191C", "1,3 butadiene (100) LP 191C", "Oil as Octane (200) LP 191C", "N2O (1000) LP 191C (2of2)", "Propane (200) LP 191C", "NO2 autorange (2000)", "CO autorange (100000)", "CH4 autorange (5000)", "NH3 autorange (3000)", "NOx autorange (3000)", "HCD (10000)", "NMHCD (10000)", "CO2% autorange (20)", "H2Oppm (300000)", "N2O autorange (1000)", "NMNEHCD (3000)", "Temp. Gascell", "Pressure Gascell", "sBeam@2500", "Temp. HL to FT-IR", "Temp. HL Extern SP1", "Outlet Temp FT-IR", "Temp. Cabinet", "Constant 0", "Constant 50", "Constant 100", "AK DUMMY"]; "Komponenten"."Komponente 3"."Konzentration IST" format="%#.4f"; "Komponenten"."Komponente 3"."Genauigkeit" format="%#.1f"; "Komponenten"."Komponente 2"."Komponente:" items=["---", "NO (3000) LP 191C", "NO2 (150) LP 191C (1of2)", "NO2 (2000) LP 191C (2of2)", "N2O (300) LP 191C (1of2)", "NH3 (300) LP 191C (1of2)", "NH3 (900,3000) LP 191C (2of2)", "HNCO (400) 191C", "H2O% (30) LP 191C", "Formaldehyde (70,500) LP 191C", "CO2 low% (4) LP 191C (2of2)", "CO2% (20) LP 191C (1of2)", "CO (700) LP 191C (1of3)", "CO% (1) LP 191C (2of3)", "Propylene (1000) LP 191C", "Aromatic HC C7 (500) LP 191C", "Ethylene (1000) LP 191C", "CH4 (250) LP 191C (1of2)", "CH4 (5000) LP 191C (2of2)", "Ethane (1000) LP 191C", "Acetylene (1000) LP 191C", "HNO2 (20) 191C", "MeOH (1000) 191C", "CO% (10) LP 191C (3of3)", "Formic Acid (100) 191C", "SO2 (500) LP 191C", "Acetaldehyde (1000) LP 191C", "COS (100) LP 191C", "1,3 butadiene (100) LP 191C", "Oil as Octane (200) LP 191C", "N2O (1000) LP 191C (2of2)", "Propane (200) LP 191C", "NO2 autorange (2000)", "CO autorange (100000)", "CH4 autorange (5000)", "NH3 autorange (3000)", "NOx autorange (3000)", "HCD (10000)", "NMHCD (10000)", "CO2% autorange (20)", "H2Oppm (300000)", "N2O autorange (1000)", "NMNEHCD (3000)", "Temp. Gascell", "Pressure Gascell", "sBeam@2500", "Temp. HL to FT-IR", "Temp. HL Extern SP1", "Outlet Temp FT-IR", "Temp. Cabinet", "Constant 0", "Constant 50", "Constant 100", "AK DUMMY"]; "Komponenten"."Komponente 2"."Konzentration IST" format="%#.4f"; "Komponenten"."Komponente 2"."Genauigkeit" format="%#.1f"; "Komponenten"."Komponente 1"."Komponente:" items=["---", "NO (3000) LP 191C", "NO2 (150) LP 191C (1of2)", "NO2 (2000) LP 191C (2of2)", "N2O (300) LP 191C (1of2)", "NH3 (300) LP 191C (1of2)", "NH3 (900,3000) LP 191C (2of2)", "HNCO (400) 191C", "H2O% (30) LP 191C", "Formaldehyde (70,500) LP 191C", "CO2 low% (4) LP 191C (2of2)", "CO2% (20) LP 191C (1of2)", "CO (700) LP 191C (1of3)", "CO% (1) LP 191C (2of3)", "Propylene (1000) LP 191C", "Aromatic HC C7 (500) LP 191C", "Ethylene (1000) LP 191C", "CH4 (250) LP 191C (1of2)", "CH4 (5000) LP 191C (2of2)", "Ethane (1000) LP 191C", "Acetylene (1000) LP 191C", "HNO2 (20) 191C", "MeOH (1000) 191C", "CO% (10) LP 191C (3of3)", "Formic Acid (100) 191C", "SO2 (500) LP 191C", "Acetaldehyde (1000) LP 191C", "COS (100) LP 191C", "1,3 butadiene (100) LP 191C", "Oil as Octane (200) LP 191C", "N2O (1000) LP 191C (2of2)", "Propane (200) LP 191C", "NO2 autorange (2000)", "CO autorange (100000)", "CH4 autorange (5000)", "NH3 autorange (3000)", "NOx autorange (3000)", "HCD (10000)", "NMHCD (10000)", "CO2% autorange (20)", "H2Oppm (300000)", "N2O autorange (1000)", "NMNEHCD (3000)", "Temp. Gascell", "Pressure Gascell", "sBeam@2500", "Temp. HL to FT-IR", "Temp. HL Extern SP1", "Outlet Temp FT-IR", "Temp. Cabinet", "Constant 0", "Constant 50", "Constant 100", "AK DUMMY"]; "Komponenten"."Komponente 1"."Konzentration IST" format="%#.4f"; "Komponenten"."Komponente 1"."Genauigkeit" format="%#.1f"; "Modus" items=["CG zu PNS", "CG zu Entnahmestelle"]; "Ablaufdatum" format="%<%d.%m.%Y>T"; "Gasflasche" items=["----"=10000, "IAG O2"=0, "IAG C2H2"=1, "IAG C2H4"=2, "IAG NH3 200"=3, "IAG NH3 2000"=4, "IAG NH3 3000"=5, "IAG CO 5%"=6, "IAG Propane 2%"=7, "IAG NO 1000"=8, "IAG SO2"=9, "IAG C3H6"=10, "IAG CO2"=11, "IAG CO"=12, "IAG N2O"=13, "IAG N2O 100"=14, "IAG NO2 1000"=15, "IAG NO2 100"=16, "IAG CH4"=17, "IAG Propane"=18, "IAG NO 5000"=19, "Hansi"=20, "IAG MG"=21]}
  in  "Span 5":T4={"Span Inlet Active"=FALSE, "Analysator"="FT-IR", "Konfig Gasflasche"=FALSE, "Gasflasche"=0, "Gasflaschen Nr.:"="", "Ablaufdatum"=timestamp(0 s since 1904-01-01), "Modus"=0, "Komponenten"={"Komponente 1"={"Komponente:"=0, "Konzentration IST"=0.0, "Einheit"=enum."ppm", "Genauigkeit"=0.0}, "Komponente 2"={"Komponente:"=0, "Konzentration IST"=0.0, "Einheit"=enum."ppm", "Genauigkeit"=0.0}, "Komponente 3"={"Komponente:"=0, "Konzentration IST"=0.0, "Einheit"=enum."ppm", "Genauigkeit"=0.0}, "Komponente 4"={"Komponente:"=0, "Konzentration IST"=0.0, "Einheit"=enum."ppm", "Genauigkeit"=0.0}, "Komponente 5"={"Komponente:"=0, "Konzentration IST"=0.0, "Einheit"=enum."ppm", "Genauigkeit"=0.0}}} {"Komponenten"."Komponente 5"."Komponente:" items=["---", "NO (3000) LP 191C", "NO2 (150) LP 191C (1of2)", "NO2 (2000) LP 191C (2of2)", "N2O (300) LP 191C (1of2)", "NH3 (300) LP 191C (1of2)", "NH3 (900,3000) LP 191C (2of2)", "HNCO (400) 191C", "H2O% (30) LP 191C", "Formaldehyde (70,500) LP 191C", "CO2 low% (4) LP 191C (2of2)", "CO2% (20) LP 191C (1of2)", "CO (700) LP 191C (1of3)", "CO% (1) LP 191C (2of3)", "Propylene (1000) LP 191C", "Aromatic HC C7 (500) LP 191C", "Ethylene (1000) LP 191C", "CH4 (250) LP 191C (1of2)", "CH4 (5000) LP 191C (2of2)", "Ethane (1000) LP 191C", "Acetylene (1000) LP 191C", "HNO2 (20) 191C", "MeOH (1000) 191C", "CO% (10) LP 191C (3of3)", "Formic Acid (100) 191C", "SO2 (500) LP 191C", "Acetaldehyde (1000) LP 191C", "COS (100) LP 191C", "1,3 butadiene (100) LP 191C", "Oil as Octane (200) LP 191C", "N2O (1000) LP 191C (2of2)", "Propane (200) LP 191C", "NO2 autorange (2000)", "CO autorange (100000)", "CH4 autorange (5000)", "NH3 autorange (3000)", "NOx autorange (3000)", "HCD (10000)", "NMHCD (10000)", "CO2% autorange (20)", "H2Oppm (300000)", "N2O autorange (1000)", "NMNEHCD (3000)", "Temp. Gascell", "Pressure Gascell", "sBeam@2500", "Temp. HL to FT-IR", "Temp. HL Extern SP1", "Outlet Temp FT-IR", "Temp. Cabinet", "Constant 0", "Constant 50", "Constant 100", "AK DUMMY"]; "Komponenten"."Komponente 5"."Konzentration IST" format="%#.4f"; "Komponenten"."Komponente 5"."Genauigkeit" format="%#.1f"; "Komponenten"."Komponente 4"."Komponente:" items=["---", "NO (3000) LP 191C", "NO2 (150) LP 191C (1of2)", "NO2 (2000) LP 191C (2of2)", "N2O (300) LP 191C (1of2)", "NH3 (300) LP 191C (1of2)", "NH3 (900,3000) LP 191C (2of2)", "HNCO (400) 191C", "H2O% (30) LP 191C", "Formaldehyde (70,500) LP 191C", "CO2 low% (4) LP 191C (2of2)", "CO2% (20) LP 191C (1of2)", "CO (700) LP 191C (1of3)", "CO% (1) LP 191C (2of3)", "Propylene (1000) LP 191C", "Aromatic HC C7 (500) LP 191C", "Ethylene (1000) LP 191C", "CH4 (250) LP 191C (1of2)", "CH4 (5000) LP 191C (2of2)", "Ethane (1000) LP 191C", "Acetylene (1000) LP 191C", "HNO2 (20) 191C", "MeOH (1000) 191C", "CO% (10) LP 191C (3of3)", "Formic Acid (100) 191C", "SO2 (500) LP 191C", "Acetaldehyde (1000) LP 191C", "COS (100) LP 191C", "1,3 butadiene (100) LP 191C", "Oil as Octane (200) LP 191C", "N2O (1000) LP 191C (2of2)", "Propane (200) LP 191C", "NO2 autorange (2000)", "CO autorange (100000)", "CH4 autorange (5000)", "NH3 autorange (3000)", "NOx autorange (3000)", "HCD (10000)", "NMHCD (10000)", "CO2% autorange (20)", "H2Oppm (300000)", "N2O autorange (1000)", "NMNEHCD (3000)", "Temp. Gascell", "Pressure Gascell", "sBeam@2500", "Temp. HL to FT-IR", "Temp. HL Extern SP1", "Outlet Temp FT-IR", "Temp. Cabinet", "Constant 0", "Constant 50", "Constant 100", "AK DUMMY"]; "Komponenten"."Komponente 4"."Konzentration IST" format="%#.4f"; "Komponenten"."Komponente 4"."Genauigkeit" format="%#.1f"; "Komponenten"."Komponente 3"."Komponente:" items=["---", "NO (3000) LP 191C", "NO2 (150) LP 191C (1of2)", "NO2 (2000) LP 191C (2of2)", "N2O (300) LP 191C (1of2)", "NH3 (300) LP 191C (1of2)", "NH3 (900,3000) LP 191C (2of2)", "HNCO (400) 191C", "H2O% (30) LP 191C", "Formaldehyde (70,500) LP 191C", "CO2 low% (4) LP 191C (2of2)", "CO2% (20) LP 191C (1of2)", "CO (700) LP 191C (1of3)", "CO% (1) LP 191C (2of3)", "Propylene (1000) LP 191C", "Aromatic HC C7 (500) LP 191C", "Ethylene (1000) LP 191C", "CH4 (250) LP 191C (1of2)", "CH4 (5000) LP 191C (2of2)", "Ethane (1000) LP 191C", "Acetylene (1000) LP 191C", "HNO2 (20) 191C", "MeOH (1000) 191C", "CO% (10) LP 191C (3of3)", "Formic Acid (100) 191C", "SO2 (500) LP 191C", "Acetaldehyde (1000) LP 191C", "COS (100) LP 191C", "1,3 butadiene (100) LP 191C", "Oil as Octane (200) LP 191C", "N2O (1000) LP 191C (2of2)", "Propane (200) LP 191C", "NO2 autorange (2000)", "CO autorange (100000)", "CH4 autorange (5000)", "NH3 autorange (3000)", "NOx autorange (3000)", "HCD (10000)", "NMHCD (10000)", "CO2% autorange (20)", "H2Oppm (300000)", "N2O autorange (1000)", "NMNEHCD (3000)", "Temp. Gascell", "Pressure Gascell", "sBeam@2500", "Temp. HL to FT-IR", "Temp. HL Extern SP1", "Outlet Temp FT-IR", "Temp. Cabinet", "Constant 0", "Constant 50", "Constant 100", "AK DUMMY"]; "Komponenten"."Komponente 3"."Konzentration IST" format="%#.4f"; "Komponenten"."Komponente 3"."Genauigkeit" format="%#.1f"; "Komponenten"."Komponente 2"."Komponente:" items=["---", "NO (3000) LP 191C", "NO2 (150) LP 191C (1of2)", "NO2 (2000) LP 191C (2of2)", "N2O (300) LP 191C (1of2)", "NH3 (300) LP 191C (1of2)", "NH3 (900,3000) LP 191C (2of2)", "HNCO (400) 191C", "H2O% (30) LP 191C", "Formaldehyde (70,500) LP 191C", "CO2 low% (4) LP 191C (2of2)", "CO2% (20) LP 191C (1of2)", "CO (700) LP 191C (1of3)", "CO% (1) LP 191C (2of3)", "Propylene (1000) LP 191C", "Aromatic HC C7 (500) LP 191C", "Ethylene (1000) LP 191C", "CH4 (250) LP 191C (1of2)", "CH4 (5000) LP 191C (2of2)", "Ethane (1000) LP 191C", "Acetylene (1000) LP 191C", "HNO2 (20) 191C", "MeOH (1000) 191C", "CO% (10) LP 191C (3of3)", "Formic Acid (100) 191C", "SO2 (500) LP 191C", "Acetaldehyde (1000) LP 191C", "COS (100) LP 191C", "1,3 butadiene (100) LP 191C", "Oil as Octane (200) LP 191C", "N2O (1000) LP 191C (2of2)", "Propane (200) LP 191C", "NO2 autorange (2000)", "CO autorange (100000)", "CH4 autorange (5000)", "NH3 autorange (3000)", "NOx autorange (3000)", "HCD (10000)", "NMHCD (10000)", "CO2% autorange (20)", "H2Oppm (300000)", "N2O autorange (1000)", "NMNEHCD (3000)", "Temp. Gascell", "Pressure Gascell", "sBeam@2500", "Temp. HL to FT-IR", "Temp. HL Extern SP1", "Outlet Temp FT-IR", "Temp. Cabinet", "Constant 0", "Constant 50", "Constant 100", "AK DUMMY"]; "Komponenten"."Komponente 2"."Konzentration IST" format="%#.4f"; "Komponenten"."Komponente 2"."Genauigkeit" format="%#.1f"; "Komponenten"."Komponente 1"."Komponente:" items=["---", "NO (3000) LP 191C", "NO2 (150) LP 191C (1of2)", "NO2 (2000) LP 191C (2of2)", "N2O (300) LP 191C (1of2)", "NH3 (300) LP 191C (1of2)", "NH3 (900,3000) LP 191C (2of2)", "HNCO (400) 191C", "H2O% (30) LP 191C", "Formaldehyde (70,500) LP 191C", "CO2 low% (4) LP 191C (2of2)", "CO2% (20) LP 191C (1of2)", "CO (700) LP 191C (1of3)", "CO% (1) LP 191C (2of3)", "Propylene (1000) LP 191C", "Aromatic HC C7 (500) LP 191C", "Ethylene (1000) LP 191C", "CH4 (250) LP 191C (1of2)", "CH4 (5000) LP 191C (2of2)", "Ethane (1000) LP 191C", "Acetylene (1000) LP 191C", "HNO2 (20) 191C", "MeOH (1000) 191C", "CO% (10) LP 191C (3of3)", "Formic Acid (100) 191C", "SO2 (500) LP 191C", "Acetaldehyde (1000) LP 191C", "COS (100) LP 191C", "1,3 butadiene (100) LP 191C", "Oil as Octane (200) LP 191C", "N2O (1000) LP 191C (2of2)", "Propane (200) LP 191C", "NO2 autorange (2000)", "CO autorange (100000)", "CH4 autorange (5000)", "NH3 autorange (3000)", "NOx autorange (3000)", "HCD (10000)", "NMHCD (10000)", "CO2% autorange (20)", "H2Oppm (300000)", "N2O autorange (1000)", "NMNEHCD (3000)", "Temp. Gascell", "Pressure Gascell", "sBeam@2500", "Temp. HL to FT-IR", "Temp. HL Extern SP1", "Outlet Temp FT-IR", "Temp. Cabinet", "Constant 0", "Constant 50", "Constant 100", "AK DUMMY"]; "Komponenten"."Komponente 1"."Konzentration IST" format="%#.4f"; "Komponenten"."Komponente 1"."Genauigkeit" format="%#.1f"; "Modus" items=["CG zu PNS", "CG zu Entnahmestelle"]; "Ablaufdatum" format="%<%d.%m.%Y>T"; "Gasflasche" items=["----"=10000, "IAG O2"=0, "IAG C2H2"=1, "IAG C2H4"=2, "IAG NH3 200"=3, "IAG NH3 2000"=4, "IAG NH3 3000"=5, "IAG CO 5%"=6, "IAG Propane 2%"=7, "IAG NO 1000"=8, "IAG SO2"=9, "IAG C3H6"=10, "IAG CO2"=11, "IAG CO"=12, "IAG N2O"=13, "IAG N2O 100"=14, "IAG NO2 1000"=15, "IAG NO2 100"=16, "IAG CH4"=17, "IAG Propane"=18, "IAG NO 5000"=19, "Hansi"=20, "IAG MG"=21]}
  in  "Span 6":T4={"Span Inlet Active"=FALSE, "Analysator"="FT-IR", "Konfig Gasflasche"=FALSE, "Gasflasche"=0, "Gasflaschen Nr.:"="", "Ablaufdatum"=timestamp(0 s since 1904-01-01), "Modus"=0, "Komponenten"={"Komponente 1"={"Komponente:"=0, "Konzentration IST"=0.0, "Einheit"=enum."ppm", "Genauigkeit"=0.0}, "Komponente 2"={"Komponente:"=0, "Konzentration IST"=0.0, "Einheit"=enum."ppm", "Genauigkeit"=0.0}, "Komponente 3"={"Komponente:"=0, "Konzentration IST"=0.0, "Einheit"=enum."ppm", "Genauigkeit"=0.0}, "Komponente 4"={"Komponente:"=0, "Konzentration IST"=0.0, "Einheit"=enum."ppm", "Genauigkeit"=0.0}, "Komponente 5"={"Komponente:"=0, "Konzentration IST"=0.0, "Einheit"=enum."ppm", "Genauigkeit"=0.0}}} {"Komponenten"."Komponente 5"."Komponente:" items=["---", "NO (3000) LP 191C", "NO2 (150) LP 191C (1of2)", "NO2 (2000) LP 191C (2of2)", "N2O (300) LP 191C (1of2)", "NH3 (300) LP 191C (1of2)", "NH3 (900,3000) LP 191C (2of2)", "HNCO (400) 191C", "H2O% (30) LP 191C", "Formaldehyde (70,500) LP 191C", "CO2 low% (4) LP 191C (2of2)", "CO2% (20) LP 191C (1of2)", "CO (700) LP 191C (1of3)", "CO% (1) LP 191C (2of3)", "Propylene (1000) LP 191C", "Aromatic HC C7 (500) LP 191C", "Ethylene (1000) LP 191C", "CH4 (250) LP 191C (1of2)", "CH4 (5000) LP 191C (2of2)", "Ethane (1000) LP 191C", "Acetylene (1000) LP 191C", "HNO2 (20) 191C", "MeOH (1000) 191C", "CO% (10) LP 191C (3of3)", "Formic Acid (100) 191C", "SO2 (500) LP 191C", "Acetaldehyde (1000) LP 191C", "COS (100) LP 191C", "1,3 butadiene (100) LP 191C", "Oil as Octane (200) LP 191C", "N2O (1000) LP 191C (2of2)", "Propane (200) LP 191C", "NO2 autorange (2000)", "CO autorange (100000)", "CH4 autorange (5000)", "NH3 autorange (3000)", "NOx autorange (3000)", "HCD (10000)", "NMHCD (10000)", "CO2% autorange (20)", "H2Oppm (300000)", "N2O autorange (1000)", "NMNEHCD (3000)", "Temp. Gascell", "Pressure Gascell", "sBeam@2500", "Temp. HL to FT-IR", "Temp. HL Extern SP1", "Outlet Temp FT-IR", "Temp. Cabinet", "Constant 0", "Constant 50", "Constant 100", "AK DUMMY"]; "Komponenten"."Komponente 5"."Konzentration IST" format="%#.4f"; "Komponenten"."Komponente 5"."Genauigkeit" format="%#.1f"; "Komponenten"."Komponente 4"."Komponente:" items=["---", "NO (3000) LP 191C", "NO2 (150) LP 191C (1of2)", "NO2 (2000) LP 191C (2of2)", "N2O (300) LP 191C (1of2)", "NH3 (300) LP 191C (1of2)", "NH3 (900,3000) LP 191C (2of2)", "HNCO (400) 191C", "H2O% (30) LP 191C", "Formaldehyde (70,500) LP 191C", "CO2 low% (4) LP 191C (2of2)", "CO2% (20) LP 191C (1of2)", "CO (700) LP 191C (1of3)", "CO% (1) LP 191C (2of3)", "Propylene (1000) LP 191C", "Aromatic HC C7 (500) LP 191C", "Ethylene (1000) LP 191C", "CH4 (250) LP 191C (1of2)", "CH4 (5000) LP 191C (2of2)", "Ethane (1000) LP 191C", "Acetylene (1000) LP 191C", "HNO2 (20) 191C", "MeOH (1000) 191C", "CO% (10) LP 191C (3of3)", "Formic Acid (100) 191C", "SO2 (500) LP 191C", "Acetaldehyde (1000) LP 191C", "COS (100) LP 191C", "1,3 butadiene (100) LP 191C", "Oil as Octane (200) LP 191C", "N2O (1000) LP 191C (2of2)", "Propane (200) LP 191C", "NO2 autorange (2000)", "CO autorange (100000)", "CH4 autorange (5000)", "NH3 autorange (3000)", "NOx autorange (3000)", "HCD (10000)", "NMHCD (10000)", "CO2% autorange (20)", "H2Oppm (300000)", "N2O autorange (1000)", "NMNEHCD (3000)", "Temp. Gascell", "Pressure Gascell", "sBeam@2500", "Temp. HL to FT-IR", "Temp. HL Extern SP1", "Outlet Temp FT-IR", "Temp. Cabinet", "Constant 0", "Constant 50", "Constant 100", "AK DUMMY"]; "Komponenten"."Komponente 4"."Konzentration IST" format="%#.4f"; "Komponenten"."Komponente 4"."Genauigkeit" format="%#.1f"; "Komponenten"."Komponente 3"."Komponente:" items=["---", "NO (3000) LP 191C", "NO2 (150) LP 191C (1of2)", "NO2 (2000) LP 191C (2of2)", "N2O (300) LP 191C (1of2)", "NH3 (300) LP 191C (1of2)", "NH3 (900,3000) LP 191C (2of2)", "HNCO (400) 191C", "H2O% (30) LP 191C", "Formaldehyde (70,500) LP 191C", "CO2 low% (4) LP 191C (2of2)", "CO2% (20) LP 191C (1of2)", "CO (700) LP 191C (1of3)", "CO% (1) LP 191C (2of3)", "Propylene (1000) LP 191C", "Aromatic HC C7 (500) LP 191C", "Ethylene (1000) LP 191C", "CH4 (250) LP 191C (1of2)", "CH4 (5000) LP 191C (2of2)", "Ethane (1000) LP 191C", "Acetylene (1000) LP 191C", "HNO2 (20) 191C", "MeOH (1000) 191C", "CO% (10) LP 191C (3of3)", "Formic Acid (100) 191C", "SO2 (500) LP 191C", "Acetaldehyde (1000) LP 191C", "COS (100) LP 191C", "1,3 butadiene (100) LP 191C", "Oil as Octane (200) LP 191C", "N2O (1000) LP 191C (2of2)", "Propane (200) LP 191C", "NO2 autorange (2000)", "CO autorange (100000)", "CH4 autorange (5000)", "NH3 autorange (3000)", "NOx autorange (3000)", "HCD (10000)", "NMHCD (10000)", "CO2% autorange (20)", "H2Oppm (300000)", "N2O autorange (1000)", "NMNEHCD (3000)", "Temp. Gascell", "Pressure Gascell", "sBeam@2500", "Temp. HL to FT-IR", "Temp. HL Extern SP1", "Outlet Temp FT-IR", "Temp. Cabinet", "Constant 0", "Constant 50", "Constant 100", "AK DUMMY"]; "Komponenten"."Komponente 3"."Konzentration IST" format="%#.4f"; "Komponenten"."Komponente 3"."Genauigkeit" format="%#.1f"; "Komponenten"."Komponente 2"."Komponente:" items=["---", "NO (3000) LP 191C", "NO2 (150) LP 191C (1of2)", "NO2 (2000) LP 191C (2of2)", "N2O (300) LP 191C (1of2)", "NH3 (300) LP 191C (1of2)", "NH3 (900,3000) LP 191C (2of2)", "HNCO (400) 191C", "H2O% (30) LP 191C", "Formaldehyde (70,500) LP 191C", "CO2 low% (4) LP 191C (2of2)", "CO2% (20) LP 191C (1of2)", "CO (700) LP 191C (1of3)", "CO% (1) LP 191C (2of3)", "Propylene (1000) LP 191C", "Aromatic HC C7 (500) LP 191C", "Ethylene (1000) LP 191C", "CH4 (250) LP 191C (1of2)", "CH4 (5000) LP 191C (2of2)", "Ethane (1000) LP 191C", "Acetylene (1000) LP 191C", "HNO2 (20) 191C", "MeOH (1000) 191C", "CO% (10) LP 191C (3of3)", "Formic Acid (100) 191C", "SO2 (500) LP 191C", "Acetaldehyde (1000) LP 191C", "COS (100) LP 191C", "1,3 butadiene (100) LP 191C", "Oil as Octane (200) LP 191C", "N2O (1000) LP 191C (2of2)", "Propane (200) LP 191C", "NO2 autorange (2000)", "CO autorange (100000)", "CH4 autorange (5000)", "NH3 autorange (3000)", "NOx autorange (3000)", "HCD (10000)", "NMHCD (10000)", "CO2% autorange (20)", "H2Oppm (300000)", "N2O autorange (1000)", "NMNEHCD (3000)", "Temp. Gascell", "Pressure Gascell", "sBeam@2500", "Temp. HL to FT-IR", "Temp. HL Extern SP1", "Outlet Temp FT-IR", "Temp. Cabinet", "Constant 0", "Constant 50", "Constant 100", "AK DUMMY"]; "Komponenten"."Komponente 2"."Konzentration IST" format="%#.4f"; "Komponenten"."Komponente 2"."Genauigkeit" format="%#.1f"; "Komponenten"."Komponente 1"."Komponente:" items=["---", "NO (3000) LP 191C", "NO2 (150) LP 191C (1of2)", "NO2 (2000) LP 191C (2of2)", "N2O (300) LP 191C (1of2)", "NH3 (300) LP 191C (1of2)", "NH3 (900,3000) LP 191C (2of2)", "HNCO (400) 191C", "H2O% (30) LP 191C", "Formaldehyde (70,500) LP 191C", "CO2 low% (4) LP 191C (2of2)", "CO2% (20) LP 191C (1of2)", "CO (700) LP 191C (1of3)", "CO% (1) LP 191C (2of3)", "Propylene (1000) LP 191C", "Aromatic HC C7 (500) LP 191C", "Ethylene (1000) LP 191C", "CH4 (250) LP 191C (1of2)", "CH4 (5000) LP 191C (2of2)", "Ethane (1000) LP 191C", "Acetylene (1000) LP 191C", "HNO2 (20) 191C", "MeOH (1000) 191C", "CO% (10) LP 191C (3of3)", "Formic Acid (100) 191C", "SO2 (500) LP 191C", "Acetaldehyde (1000) LP 191C", "COS (100) LP 191C", "1,3 butadiene (100) LP 191C", "Oil as Octane (200) LP 191C", "N2O (1000) LP 191C (2of2)", "Propane (200) LP 191C", "NO2 autorange (2000)", "CO autorange (100000)", "CH4 autorange (5000)", "NH3 autorange (3000)", "NOx autorange (3000)", "HCD (10000)", "NMHCD (10000)", "CO2% autorange (20)", "H2Oppm (300000)", "N2O autorange (1000)", "NMNEHCD (3000)", "Temp. Gascell", "Pressure Gascell", "sBeam@2500", "Temp. HL to FT-IR", "Temp. HL Extern SP1", "Outlet Temp FT-IR", "Temp. Cabinet", "Constant 0", "Constant 50", "Constant 100", "AK DUMMY"]; "Komponenten"."Komponente 1"."Konzentration IST" format="%#.4f"; "Komponenten"."Komponente 1"."Genauigkeit" format="%#.1f"; "Modus" items=["CG zu PNS", "CG zu Entnahmestelle"]; "Ablaufdatum" format="%<%d.%m.%Y>T"; "Gasflasche" items=["----"=10000, "IAG O2"=0, "IAG C2H2"=1, "IAG C2H4"=2, "IAG NH3 200"=3, "IAG NH3 2000"=4, "IAG NH3 3000"=5, "IAG CO 5%"=6, "IAG Propane 2%"=7, "IAG NO 1000"=8, "IAG SO2"=9, "IAG C3H6"=10, "IAG CO2"=11, "IAG CO"=12, "IAG N2O"=13, "IAG N2O 100"=14, "IAG NO2 1000"=15, "IAG NO2 100"=16, "IAG CH4"=17, "IAG Propane"=18, "IAG NO 5000"=19, "Hansi"=20, "IAG MG"=21]}
  in  "Span 7":T4={"Span Inlet Active"=FALSE, "Analysator"="FT-IR", "Konfig Gasflasche"=FALSE, "Gasflasche"=0, "Gasflaschen Nr.:"="", "Ablaufdatum"=timestamp(0 s since 1904-01-01), "Modus"=0, "Komponenten"={"Komponente 1"={"Komponente:"=0, "Konzentration IST"=0.0, "Einheit"=enum."ppm", "Genauigkeit"=0.0}, "Komponente 2"={"Komponente:"=0, "Konzentration IST"=0.0, "Einheit"=enum."ppm", "Genauigkeit"=0.0}, "Komponente 3"={"Komponente:"=0, "Konzentration IST"=0.0, "Einheit"=enum."ppm", "Genauigkeit"=0.0}, "Komponente 4"={"Komponente:"=0, "Konzentration IST"=0.0, "Einheit"=enum."ppm", "Genauigkeit"=0.0}, "Komponente 5"={"Komponente:"=0, "Konzentration IST"=0.0, "Einheit"=enum."ppm", "Genauigkeit"=0.0}}} {"Komponenten"."Komponente 5"."Komponente:" items=["---", "NO (3000) LP 191C", "NO2 (150) LP 191C (1of2)", "NO2 (2000) LP 191C (2of2)", "N2O (300) LP 191C (1of2)", "NH3 (300) LP 191C (1of2)", "NH3 (900,3000) LP 191C (2of2)", "HNCO (400) 191C", "H2O% (30) LP 191C", "Formaldehyde (70,500) LP 191C", "CO2 low% (4) LP 191C (2of2)", "CO2% (20) LP 191C (1of2)", "CO (700) LP 191C (1of3)", "CO% (1) LP 191C (2of3)", "Propylene (1000) LP 191C", "Aromatic HC C7 (500) LP 191C", "Ethylene (1000) LP 191C", "CH4 (250) LP 191C (1of2)", "CH4 (5000) LP 191C (2of2)", "Ethane (1000) LP 191C", "Acetylene (1000) LP 191C", "HNO2 (20) 191C", "MeOH (1000) 191C", "CO% (10) LP 191C (3of3)", "Formic Acid (100) 191C", "SO2 (500) LP 191C", "Acetaldehyde (1000) LP 191C", "COS (100) LP 191C", "1,3 butadiene (100) LP 191C", "Oil as Octane (200) LP 191C", "N2O (1000) LP 191C (2of2)", "Propane (200) LP 191C", "NO2 autorange (2000)", "CO autorange (100000)", "CH4 autorange (5000)", "NH3 autorange (3000)", "NOx autorange (3000)", "HCD (10000)", "NMHCD (10000)", "CO2% autorange (20)", "H2Oppm (300000)", "N2O autorange (1000)", "NMNEHCD (3000)", "Temp. Gascell", "Pressure Gascell", "sBeam@2500", "Temp. HL to FT-IR", "Temp. HL Extern SP1", "Outlet Temp FT-IR", "Temp. Cabinet", "Constant 0", "Constant 50", "Constant 100", "AK DUMMY"]; "Komponenten"."Komponente 5"."Konzentration IST" format="%#.4f"; "Komponenten"."Komponente 5"."Genauigkeit" format="%#.1f"; "Komponenten"."Komponente 4"."Komponente:" items=["---", "NO (3000) LP 191C", "NO2 (150) LP 191C (1of2)", "NO2 (2000) LP 191C (2of2)", "N2O (300) LP 191C (1of2)", "NH3 (300) LP 191C (1of2)", "NH3 (900,3000) LP 191C (2of2)", "HNCO (400) 191C", "H2O% (30) LP 191C", "Formaldehyde (70,500) LP 191C", "CO2 low% (4) LP 191C (2of2)", "CO2% (20) LP 191C (1of2)", "CO (700) LP 191C (1of3)", "CO% (1) LP 191C (2of3)", "Propylene (1000) LP 191C", "Aromatic HC C7 (500) LP 191C", "Ethylene (1000) LP 191C", "CH4 (250) LP 191C (1of2)", "CH4 (5000) LP 191C (2of2)", "Ethane (1000) LP 191C", "Acetylene (1000) LP 191C", "HNO2 (20) 191C", "MeOH (1000) 191C", "CO% (10) LP 191C (3of3)", "Formic Acid (100) 191C", "SO2 (500) LP 191C", "Acetaldehyde (1000) LP 191C", "COS (100) LP 191C", "1,3 butadiene (100) LP 191C", "Oil as Octane (200) LP 191C", "N2O (1000) LP 191C (2of2)", "Propane (200) LP 191C", "NO2 autorange (2000)", "CO autorange (100000)", "CH4 autorange (5000)", "NH3 autorange (3000)", "NOx autorange (3000)", "HCD (10000)", "NMHCD (10000)", "CO2% autorange (20)", "H2Oppm (300000)", "N2O autorange (1000)", "NMNEHCD (3000)", "Temp. Gascell", "Pressure Gascell", "sBeam@2500", "Temp. HL to FT-IR", "Temp. HL Extern SP1", "Outlet Temp FT-IR", "Temp. Cabinet", "Constant 0", "Constant 50", "Constant 100", "AK DUMMY"]; "Komponenten"."Komponente 4"."Konzentration IST" format="%#.4f"; "Komponenten"."Komponente 4"."Genauigkeit" format="%#.1f"; "Komponenten"."Komponente 3"."Komponente:" items=["---", "NO (3000) LP 191C", "NO2 (150) LP 191C (1of2)", "NO2 (2000) LP 191C (2of2)", "N2O (300) LP 191C (1of2)", "NH3 (300) LP 191C (1of2)", "NH3 (900,3000) LP 191C (2of2)", "HNCO (400) 191C", "H2O% (30) LP 191C", "Formaldehyde (70,500) LP 191C", "CO2 low% (4) LP 191C (2of2)", "CO2% (20) LP 191C (1of2)", "CO (700) LP 191C (1of3)", "CO% (1) LP 191C (2of3)", "Propylene (1000) LP 191C", "Aromatic HC C7 (500) LP 191C", "Ethylene (1000) LP 191C", "CH4 (250) LP 191C (1of2)", "CH4 (5000) LP 191C (2of2)", "Ethane (1000) LP 191C", "Acetylene (1000) LP 191C", "HNO2 (20) 191C", "MeOH (1000) 191C", "CO% (10) LP 191C (3of3)", "Formic Acid (100) 191C", "SO2 (500) LP 191C", "Acetaldehyde (1000) LP 191C", "COS (100) LP 191C", "1,3 butadiene (100) LP 191C", "Oil as Octane (200) LP 191C", "N2O (1000) LP 191C (2of2)", "Propane (200) LP 191C", "NO2 autorange (2000)", "CO autorange (100000)", "CH4 autorange (5000)", "NH3 autorange (3000)", "NOx autorange (3000)", "HCD (10000)", "NMHCD (10000)", "CO2% autorange (20)", "H2Oppm (300000)", "N2O autorange (1000)", "NMNEHCD (3000)", "Temp. Gascell", "Pressure Gascell", "sBeam@2500", "Temp. HL to FT-IR", "Temp. HL Extern SP1", "Outlet Temp FT-IR", "Temp. Cabinet", "Constant 0", "Constant 50", "Constant 100", "AK DUMMY"]; "Komponenten"."Komponente 3"."Konzentration IST" format="%#.4f"; "Komponenten"."Komponente 3"."Genauigkeit" format="%#.1f"; "Komponenten"."Komponente 2"."Komponente:" items=["---", "NO (3000) LP 191C", "NO2 (150) LP 191C (1of2)", "NO2 (2000) LP 191C (2of2)", "N2O (300) LP 191C (1of2)", "NH3 (300) LP 191C (1of2)", "NH3 (900,3000) LP 191C (2of2)", "HNCO (400) 191C", "H2O% (30) LP 191C", "Formaldehyde (70,500) LP 191C", "CO2 low% (4) LP 191C (2of2)", "CO2% (20) LP 191C (1of2)", "CO (700) LP 191C (1of3)", "CO% (1) LP 191C (2of3)", "Propylene (1000) LP 191C", "Aromatic HC C7 (500) LP 191C", "Ethylene (1000) LP 191C", "CH4 (250) LP 191C (1of2)", "CH4 (5000) LP 191C (2of2)", "Ethane (1000) LP 191C", "Acetylene (1000) LP 191C", "HNO2 (20) 191C", "MeOH (1000) 191C", "CO% (10) LP 191C (3of3)", "Formic Acid (100) 191C", "SO2 (500) LP 191C", "Acetaldehyde (1000) LP 191C", "COS (100) LP 191C", "1,3 butadiene (100) LP 191C", "Oil as Octane (200) LP 191C", "N2O (1000) LP 191C (2of2)", "Propane (200) LP 191C", "NO2 autorange (2000)", "CO autorange (100000)", "CH4 autorange (5000)", "NH3 autorange (3000)", "NOx autorange (3000)", "HCD (10000)", "NMHCD (10000)", "CO2% autorange (20)", "H2Oppm (300000)", "N2O autorange (1000)", "NMNEHCD (3000)", "Temp. Gascell", "Pressure Gascell", "sBeam@2500", "Temp. HL to FT-IR", "Temp. HL Extern SP1", "Outlet Temp FT-IR", "Temp. Cabinet", "Constant 0", "Constant 50", "Constant 100", "AK DUMMY"]; "Komponenten"."Komponente 2"."Konzentration IST" format="%#.4f"; "Komponenten"."Komponente 2"."Genauigkeit" format="%#.1f"; "Komponenten"."Komponente 1"."Komponente:" items=["---", "NO (3000) LP 191C", "NO2 (150) LP 191C (1of2)", "NO2 (2000) LP 191C (2of2)", "N2O (300) LP 191C (1of2)", "NH3 (300) LP 191C (1of2)", "NH3 (900,3000) LP 191C (2of2)", "HNCO (400) 191C", "H2O% (30) LP 191C", "Formaldehyde (70,500) LP 191C", "CO2 low% (4) LP 191C (2of2)", "CO2% (20) LP 191C (1of2)", "CO (700) LP 191C (1of3)", "CO% (1) LP 191C (2of3)", "Propylene (1000) LP 191C", "Aromatic HC C7 (500) LP 191C", "Ethylene (1000) LP 191C", "CH4 (250) LP 191C (1of2)", "CH4 (5000) LP 191C (2of2)", "Ethane (1000) LP 191C", "Acetylene (1000) LP 191C", "HNO2 (20) 191C", "MeOH (1000) 191C", "CO% (10) LP 191C (3of3)", "Formic Acid (100) 191C", "SO2 (500) LP 191C", "Acetaldehyde (1000) LP 191C", "COS (100) LP 191C", "1,3 butadiene (100) LP 191C", "Oil as Octane (200) LP 191C", "N2O (1000) LP 191C (2of2)", "Propane (200) LP 191C", "NO2 autorange (2000)", "CO autorange (100000)", "CH4 autorange (5000)", "NH3 autorange (3000)", "NOx autorange (3000)", "HCD (10000)", "NMHCD (10000)", "CO2% autorange (20)", "H2Oppm (300000)", "N2O autorange (1000)", "NMNEHCD (3000)", "Temp. Gascell", "Pressure Gascell", "sBeam@2500", "Temp. HL to FT-IR", "Temp. HL Extern SP1", "Outlet Temp FT-IR", "Temp. Cabinet", "Constant 0", "Constant 50", "Constant 100", "AK DUMMY"]; "Komponenten"."Komponente 1"."Konzentration IST" format="%#.4f"; "Komponenten"."Komponente 1"."Genauigkeit" format="%#.1f"; "Modus" items=["CG zu PNS", "CG zu Entnahmestelle"]; "Ablaufdatum" format="%<%d.%m.%Y>T"; "Gasflasche" items=["----"=10000, "IAG O2"=0, "IAG C2H2"=1, "IAG C2H4"=2, "IAG NH3 200"=3, "IAG NH3 2000"=4, "IAG NH3 3000"=5, "IAG CO 5%"=6, "IAG Propane 2%"=7, "IAG NO 1000"=8, "IAG SO2"=9, "IAG C3H6"=10, "IAG CO2"=11, "IAG CO"=12, "IAG N2O"=13, "IAG N2O 100"=14, "IAG NO2 1000"=15, "IAG NO2 100"=16, "IAG CH4"=17, "IAG Propane"=18, "IAG NO 5000"=19, "Hansi"=20, "IAG MG"=21]}
  in  "Span 8":T4={"Span Inlet Active"=FALSE, "Analysator"="FT-IR", "Konfig Gasflasche"=FALSE, "Gasflasche"=0, "Gasflaschen Nr.:"="", "Ablaufdatum"=timestamp(0 s since 1904-01-01), "Modus"=0, "Komponenten"={"Komponente 1"={"Komponente:"=0, "Konzentration IST"=0.0, "Einheit"=enum."ppm", "Genauigkeit"=0.0}, "Komponente 2"={"Komponente:"=0, "Konzentration IST"=0.0, "Einheit"=enum."ppm", "Genauigkeit"=0.0}, "Komponente 3"={"Komponente:"=0, "Konzentration IST"=0.0, "Einheit"=enum."ppm", "Genauigkeit"=0.0}, "Komponente 4"={"Komponente:"=0, "Konzentration IST"=0.0, "Einheit"=enum."ppm", "Genauigkeit"=0.0}, "Komponente 5"={"Komponente:"=0, "Konzentration IST"=0.0, "Einheit"=enum."ppm", "Genauigkeit"=0.0}}} {"Komponenten"."Komponente 5"."Komponente:" items=["---", "NO (3000) LP 191C", "NO2 (150) LP 191C (1of2)", "NO2 (2000) LP 191C (2of2)", "N2O (300) LP 191C (1of2)", "NH3 (300) LP 191C (1of2)", "NH3 (900,3000) LP 191C (2of2)", "HNCO (400) 191C", "H2O% (30) LP 191C", "Formaldehyde (70,500) LP 191C", "CO2 low% (4) LP 191C (2of2)", "CO2% (20) LP 191C (1of2)", "CO (700) LP 191C (1of3)", "CO% (1) LP 191C (2of3)", "Propylene (1000) LP 191C", "Aromatic HC C7 (500) LP 191C", "Ethylene (1000) LP 191C", "CH4 (250) LP 191C (1of2)", "CH4 (5000) LP 191C (2of2)", "Ethane (1000) LP 191C", "Acetylene (1000) LP 191C", "HNO2 (20) 191C", "MeOH (1000) 191C", "CO% (10) LP 191C (3of3)", "Formic Acid (100) 191C", "SO2 (500) LP 191C", "Acetaldehyde (1000) LP 191C", "COS (100) LP 191C", "1,3 butadiene (100) LP 191C", "Oil as Octane (200) LP 191C", "N2O (1000) LP 191C (2of2)", "Propane (200) LP 191C", "NO2 autorange (2000)", "CO autorange (100000)", "CH4 autorange (5000)", "NH3 autorange (3000)", "NOx autorange (3000)", "HCD (10000)", "NMHCD (10000)", "CO2% autorange (20)", "H2Oppm (300000)", "N2O autorange (1000)", "NMNEHCD (3000)", "Temp. Gascell", "Pressure Gascell", "sBeam@2500", "Temp. HL to FT-IR", "Temp. HL Extern SP1", "Outlet Temp FT-IR", "Temp. Cabinet", "Constant 0", "Constant 50", "Constant 100", "AK DUMMY"]; "Komponenten"."Komponente 5"."Konzentration IST" format="%#.4f"; "Komponenten"."Komponente 5"."Genauigkeit" format="%#.1f"; "Komponenten"."Komponente 4"."Komponente:" items=["---", "NO (3000) LP 191C", "NO2 (150) LP 191C (1of2)", "NO2 (2000) LP 191C (2of2)", "N2O (300) LP 191C (1of2)", "NH3 (300) LP 191C (1of2)", "NH3 (900,3000) LP 191C (2of2)", "HNCO (400) 191C", "H2O% (30) LP 191C", "Formaldehyde (70,500) LP 191C", "CO2 low% (4) LP 191C (2of2)", "CO2% (20) LP 191C (1of2)", "CO (700) LP 191C (1of3)", "CO% (1) LP 191C (2of3)", "Propylene (1000) LP 191C", "Aromatic HC C7 (500) LP 191C", "Ethylene (1000) LP 191C", "CH4 (250) LP 191C (1of2)", "CH4 (5000) LP 191C (2of2)", "Ethane (1000) LP 191C", "Acetylene (1000) LP 191C", "HNO2 (20) 191C", "MeOH (1000) 191C", "CO% (10) LP 191C (3of3)", "Formic Acid (100) 191C", "SO2 (500) LP 191C", "Acetaldehyde (1000) LP 191C", "COS (100) LP 191C", "1,3 butadiene (100) LP 191C", "Oil as Octane (200) LP 191C", "N2O (1000) LP 191C (2of2)", "Propane (200) LP 191C", "NO2 autorange (2000)", "CO autorange (100000)", "CH4 autorange (5000)", "NH3 autorange (3000)", "NOx autorange (3000)", "HCD (10000)", "NMHCD (10000)", "CO2% autorange (20)", "H2Oppm (300000)", "N2O autorange (1000)", "NMNEHCD (3000)", "Temp. Gascell", "Pressure Gascell", "sBeam@2500", "Temp. HL to FT-IR", "Temp. HL Extern SP1", "Outlet Temp FT-IR", "Temp. Cabinet", "Constant 0", "Constant 50", "Constant 100", "AK DUMMY"]; "Komponenten"."Komponente 4"."Konzentration IST" format="%#.4f"; "Komponenten"."Komponente 4"."Genauigkeit" format="%#.1f"; "Komponenten"."Komponente 3"."Komponente:" items=["---", "NO (3000) LP 191C", "NO2 (150) LP 191C (1of2)", "NO2 (2000) LP 191C (2of2)", "N2O (300) LP 191C (1of2)", "NH3 (300) LP 191C (1of2)", "NH3 (900,3000) LP 191C (2of2)", "HNCO (400) 191C", "H2O% (30) LP 191C", "Formaldehyde (70,500) LP 191C", "CO2 low% (4) LP 191C (2of2)", "CO2% (20) LP 191C (1of2)", "CO (700) LP 191C (1of3)", "CO% (1) LP 191C (2of3)", "Propylene (1000) LP 191C", "Aromatic HC C7 (500) LP 191C", "Ethylene (1000) LP 191C", "CH4 (250) LP 191C (1of2)", "CH4 (5000) LP 191C (2of2)", "Ethane (1000) LP 191C", "Acetylene (1000) LP 191C", "HNO2 (20) 191C", "MeOH (1000) 191C", "CO% (10) LP 191C (3of3)", "Formic Acid (100) 191C", "SO2 (500) LP 191C", "Acetaldehyde (1000) LP 191C", "COS (100) LP 191C", "1,3 butadiene (100) LP 191C", "Oil as Octane (200) LP 191C", "N2O (1000) LP 191C (2of2)", "Propane (200) LP 191C", "NO2 autorange (2000)", "CO autorange (100000)", "CH4 autorange (5000)", "NH3 autorange (3000)", "NOx autorange (3000)", "HCD (10000)", "NMHCD (10000)", "CO2% autorange (20)", "H2Oppm (300000)", "N2O autorange (1000)", "NMNEHCD (3000)", "Temp. Gascell", "Pressure Gascell", "sBeam@2500", "Temp. HL to FT-IR", "Temp. HL Extern SP1", "Outlet Temp FT-IR", "Temp. Cabinet", "Constant 0", "Constant 50", "Constant 100", "AK DUMMY"]; "Komponenten"."Komponente 3"."Konzentration IST" format="%#.4f"; "Komponenten"."Komponente 3"."Genauigkeit" format="%#.1f"; "Komponenten"."Komponente 2"."Komponente:" items=["---", "NO (3000) LP 191C", "NO2 (150) LP 191C (1of2)", "NO2 (2000) LP 191C (2of2)", "N2O (300) LP 191C (1of2)", "NH3 (300) LP 191C (1of2)", "NH3 (900,3000) LP 191C (2of2)", "HNCO (400) 191C", "H2O% (30) LP 191C", "Formaldehyde (70,500) LP 191C", "CO2 low% (4) LP 191C (2of2)", "CO2% (20) LP 191C (1of2)", "CO (700) LP 191C (1of3)", "CO% (1) LP 191C (2of3)", "Propylene (1000) LP 191C", "Aromatic HC C7 (500) LP 191C", "Ethylene (1000) LP 191C", "CH4 (250) LP 191C (1of2)", "CH4 (5000) LP 191C (2of2)", "Ethane (1000) LP 191C", "Acetylene (1000) LP 191C", "HNO2 (20) 191C", "MeOH (1000) 191C", "CO% (10) LP 191C (3of3)", "Formic Acid (100) 191C", "SO2 (500) LP 191C", "Acetaldehyde (1000) LP 191C", "COS (100) LP 191C", "1,3 butadiene (100) LP 191C", "Oil as Octane (200) LP 191C", "N2O (1000) LP 191C (2of2)", "Propane (200) LP 191C", "NO2 autorange (2000)", "CO autorange (100000)", "CH4 autorange (5000)", "NH3 autorange (3000)", "NOx autorange (3000)", "HCD (10000)", "NMHCD (10000)", "CO2% autorange (20)", "H2Oppm (300000)", "N2O autorange (1000)", "NMNEHCD (3000)", "Temp. Gascell", "Pressure Gascell", "sBeam@2500", "Temp. HL to FT-IR", "Temp. HL Extern SP1", "Outlet Temp FT-IR", "Temp. Cabinet", "Constant 0", "Constant 50", "Constant 100", "AK DUMMY"]; "Komponenten"."Komponente 2"."Konzentration IST" format="%#.4f"; "Komponenten"."Komponente 2"."Genauigkeit" format="%#.1f"; "Komponenten"."Komponente 1"."Komponente:" items=["---", "NO (3000) LP 191C", "NO2 (150) LP 191C (1of2)", "NO2 (2000) LP 191C (2of2)", "N2O (300) LP 191C (1of2)", "NH3 (300) LP 191C (1of2)", "NH3 (900,3000) LP 191C (2of2)", "HNCO (400) 191C", "H2O% (30) LP 191C", "Formaldehyde (70,500) LP 191C", "CO2 low% (4) LP 191C (2of2)", "CO2% (20) LP 191C (1of2)", "CO (700) LP 191C (1of3)", "CO% (1) LP 191C (2of3)", "Propylene (1000) LP 191C", "Aromatic HC C7 (500) LP 191C", "Ethylene (1000) LP 191C", "CH4 (250) LP 191C (1of2)", "CH4 (5000) LP 191C (2of2)", "Ethane (1000) LP 191C", "Acetylene (1000) LP 191C", "HNO2 (20) 191C", "MeOH (1000) 191C", "CO% (10) LP 191C (3of3)", "Formic Acid (100) 191C", "SO2 (500) LP 191C", "Acetaldehyde (1000) LP 191C", "COS (100) LP 191C", "1,3 butadiene (100) LP 191C", "Oil as Octane (200) LP 191C", "N2O (1000) LP 191C (2of2)", "Propane (200) LP 191C", "NO2 autorange (2000)", "CO autorange (100000)", "CH4 autorange (5000)", "NH3 autorange (3000)", "NOx autorange (3000)", "HCD (10000)", "NMHCD (10000)", "CO2% autorange (20)", "H2Oppm (300000)", "N2O autorange (1000)", "NMNEHCD (3000)", "Temp. Gascell", "Pressure Gascell", "sBeam@2500", "Temp. HL to FT-IR", "Temp. HL Extern SP1", "Outlet Temp FT-IR", "Temp. Cabinet", "Constant 0", "Constant 50", "Constant 100", "AK DUMMY"]; "Komponenten"."Komponente 1"."Konzentration IST" format="%#.4f"; "Komponenten"."Komponente 1"."Genauigkeit" format="%#.1f"; "Modus" items=["CG zu PNS", "CG zu Entnahmestelle"]; "Ablaufdatum" format="%<%d.%m.%Y>T"; "Gasflasche" items=["----"=10000, "IAG O2"=0, "IAG C2H2"=1, "IAG C2H4"=2, "IAG NH3 200"=3, "IAG NH3 2000"=4, "IAG NH3 3000"=5, "IAG CO 5%"=6, "IAG Propane 2%"=7, "IAG NO 1000"=8, "IAG SO2"=9, "IAG C3H6"=10, "IAG CO2"=11, "IAG CO"=12, "IAG N2O"=13, "IAG N2O 100"=14, "IAG NO2 1000"=15, "IAG NO2 100"=16, "IAG CH4"=17, "IAG Propane"=18, "IAG NO 5000"=19, "Hansi"=20, "IAG MG"=21]}
  in  "Span 9":T4={"Span Inlet Active"=FALSE, "Analysator"="FT-IR", "Konfig Gasflasche"=FALSE, "Gasflasche"=0, "Gasflaschen Nr.:"="", "Ablaufdatum"=timestamp(0 s since 1904-01-01), "Modus"=0, "Komponenten"={"Komponente 1"={"Komponente:"=0, "Konzentration IST"=0.0, "Einheit"=enum."ppm", "Genauigkeit"=0.0}, "Komponente 2"={"Komponente:"=0, "Konzentration IST"=0.0, "Einheit"=enum."ppm", "Genauigkeit"=0.0}, "Komponente 3"={"Komponente:"=0, "Konzentration IST"=0.0, "Einheit"=enum."ppm", "Genauigkeit"=0.0}, "Komponente 4"={"Komponente:"=0, "Konzentration IST"=0.0, "Einheit"=enum."ppm", "Genauigkeit"=0.0}, "Komponente 5"={"Komponente:"=0, "Konzentration IST"=0.0, "Einheit"=enum."ppm", "Genauigkeit"=0.0}}} {"Komponenten"."Komponente 5"."Komponente:" items=["NO (350,3000) LP 191C", "NO2 (150) LP 191C (1of2)", "NO2 (2000) LP 191C (2of2)", "N2O (300) LP 191C (1of2)", "NH3 (300) LP 191C (1of2)", "NH3 (900,3000) LP 191C (2of2)", "HNCO (400) 191C", "H2O% (30) LP 191C", "Formaldehyde (70,500) LP 191C", "CO2 low% (4) LP 191C (2of2)", "CO2% (20) LP 191C (1of2)", "CO (700) LP 191C (1of3)", "CO% (1) LP 191C (2of3)", "Propylene (1000) LP 191C", "Aromatic HC C7 (500) LP 191C", "Ethylene (1000) LP 191C", "CH4 (250) LP 191C (1of2)", "CH4 (5000) LP 191C (2of2)", "Ethane (1000) LP 191C", "Acetylene (1000) LP 191C", "HNO2 (20) 191C", "MeOH (1000) 191C", "CO% (10) LP 191C (3of3)", "Formic Acid (100) 191C", "SO2 (500) LP 191C", "Acetaldehyde (1000) LP 191C", "COS (100) LP 191C", "1,3 butadiene (100) LP 191C", "Oil as Octane (200) LP 191C", "N2O (1000) LP 191C (2of2)", "Propane (200) LP 191C", "NO2 autorange (2000)", "CO autorange (100000)", "CH4 autorange (5000)", "NH3 autorange (3000)", "Temp. Gascell", "Pressure Gascell", "sBeam@2500"]; "Komponenten"."Komponente 5"."Konzentration IST" format="%#.4f"; "Komponenten"."Komponente 5"."Genauigkeit" format="%#.1f"; "Komponenten"."Komponente 4"."Komponente:" items=["NO (350,3000) LP 191C", "NO2 (150) LP 191C (1of2)", "NO2 (2000) LP 191C (2of2)", "N2O (300) LP 191C (1of2)", "NH3 (300) LP 191C (1of2)", "NH3 (900,3000) LP 191C (2of2)", "HNCO (400) 191C", "H2O% (30) LP 191C", "Formaldehyde (70,500) LP 191C", "CO2 low% (4) LP 191C (2of2)", "CO2% (20) LP 191C (1of2)", "CO (700) LP 191C (1of3)", "CO% (1) LP 191C (2of3)", "Propylene (1000) LP 191C", "Aromatic HC C7 (500) LP 191C", "Ethylene (1000) LP 191C", "CH4 (250) LP 191C (1of2)", "CH4 (5000) LP 191C (2of2)", "Ethane (1000) LP 191C", "Acetylene (1000) LP 191C", "HNO2 (20) 191C", "MeOH (1000) 191C", "CO% (10) LP 191C (3of3)", "Formic Acid (100) 191C", "SO2 (500) LP 191C", "Acetaldehyde (1000) LP 191C", "COS (100) LP 191C", "1,3 butadiene (100) LP 191C", "Oil as Octane (200) LP 191C", "N2O (1000) LP 191C (2of2)", "Propane (200) LP 191C", "NO2 autorange (2000)", "CO autorange (100000)", "CH4 autorange (5000)", "NH3 autorange (3000)", "Temp. Gascell", "Pressure Gascell", "sBeam@2500"]; "Komponenten"."Komponente 4"."Konzentration IST" format="%#.4f"; "Komponenten"."Komponente 4"."Genauigkeit" format="%#.1f"; "Komponenten"."Komponente 3"."Komponente:" items=["NO (350,3000) LP 191C", "NO2 (150) LP 191C (1of2)", "NO2 (2000) LP 191C (2of2)", "N2O (300) LP 191C (1of2)", "NH3 (300) LP 191C (1of2)", "NH3 (900,3000) LP 191C (2of2)", "HNCO (400) 191C", "H2O% (30) LP 191C", "Formaldehyde (70,500) LP 191C", "CO2 low% (4) LP 191C (2of2)", "CO2% (20) LP 191C (1of2)", "CO (700) LP 191C (1of3)", "CO% (1) LP 191C (2of3)", "Propylene (1000) LP 191C", "Aromatic HC C7 (500) LP 191C", "Ethylene (1000) LP 191C", "CH4 (250) LP 191C (1of2)", "CH4 (5000) LP 191C (2of2)", "Ethane (1000) LP 191C", "Acetylene (1000) LP 191C", "HNO2 (20) 191C", "MeOH (1000) 191C", "CO% (10) LP 191C (3of3)", "Formic Acid (100) 191C", "SO2 (500) LP 191C", "Acetaldehyde (1000) LP 191C", "COS (100) LP 191C", "1,3 butadiene (100) LP 191C", "Oil as Octane (200) LP 191C", "N2O (1000) LP 191C (2of2)", "Propane (200) LP 191C", "NO2 autorange (2000)", "CO autorange (100000)", "CH4 autorange (5000)", "NH3 autorange (3000)", "Temp. Gascell", "Pressure Gascell", "sBeam@2500"]; "Komponenten"."Komponente 3"."Konzentration IST" format="%#.4f"; "Komponenten"."Komponente 3"."Genauigkeit" format="%#.1f"; "Komponenten"."Komponente 2"."Komponente:" items=["NO (350,3000) LP 191C", "NO2 (150) LP 191C (1of2)", "NO2 (2000) LP 191C (2of2)", "N2O (300) LP 191C (1of2)", "NH3 (300) LP 191C (1of2)", "NH3 (900,3000) LP 191C (2of2)", "HNCO (400) 191C", "H2O% (30) LP 191C", "Formaldehyde (70,500) LP 191C", "CO2 low% (4) LP 191C (2of2)", "CO2% (20) LP 191C (1of2)", "CO (700) LP 191C (1of3)", "CO% (1) LP 191C (2of3)", "Propylene (1000) LP 191C", "Aromatic HC C7 (500) LP 191C", "Ethylene (1000) LP 191C", "CH4 (250) LP 191C (1of2)", "CH4 (5000) LP 191C (2of2)", "Ethane (1000) LP 191C", "Acetylene (1000) LP 191C", "HNO2 (20) 191C", "MeOH (1000) 191C", "CO% (10) LP 191C (3of3)", "Formic Acid (100) 191C", "SO2 (500) LP 191C", "Acetaldehyde (1000) LP 191C", "COS (100) LP 191C", "1,3 butadiene (100) LP 191C", "Oil as Octane (200) LP 191C", "N2O (1000) LP 191C (2of2)", "Propane (200) LP 191C", "NO2 autorange (2000)", "CO autorange (100000)", "CH4 autorange (5000)", "NH3 autorange (3000)", "Temp. Gascell", "Pressure Gascell", "sBeam@2500"]; "Komponenten"."Komponente 2"."Konzentration IST" format="%#.4f"; "Komponenten"."Komponente 2"."Genauigkeit" format="%#.1f"; "Komponenten"."Komponente 1"."Komponente:" items=["NO (350,3000) LP 191C", "NO2 (150) LP 191C (1of2)", "NO2 (2000) LP 191C (2of2)", "N2O (300) LP 191C (1of2)", "NH3 (300) LP 191C (1of2)", "NH3 (900,3000) LP 191C (2of2)", "HNCO (400) 191C", "H2O% (30) LP 191C", "Formaldehyde (70,500) LP 191C", "CO2 low% (4) LP 191C (2of2)", "CO2% (20) LP 191C (1of2)", "CO (700) LP 191C (1of3)", "CO% (1) LP 191C (2of3)", "Propylene (1000) LP 191C", "Aromatic HC C7 (500) LP 191C", "Ethylene (1000) LP 191C", "CH4 (250) LP 191C (1of2)", "CH4 (5000) LP 191C (2of2)", "Ethane (1000) LP 191C", "Acetylene (1000) LP 191C", "HNO2 (20) 191C", "MeOH (1000) 191C", "CO% (10) LP 191C (3of3)", "Formic Acid (100) 191C", "SO2 (500) LP 191C", "Acetaldehyde (1000) LP 191C", "COS (100) LP 191C", "1,3 butadiene (100) LP 191C", "Oil as Octane (200) LP 191C", "N2O (1000) LP 191C (2of2)", "Propane (200) LP 191C", "NO2 autorange (2000)", "CO autorange (100000)", "CH4 autorange (5000)", "NH3 autorange (3000)", "Temp. Gascell", "Pressure Gascell", "sBeam@2500"]; "Komponenten"."Komponente 1"."Konzentration IST" format="%#.4f"; "Komponenten"."Komponente 1"."Genauigkeit" format="%#.1f"; "Modus" items=["CG zu PNS", "CG zu Entnahmestelle"]; "Ablaufdatum" format="%<%d.%m.%Y>T"; "Gasflasche" items=["----"=10000, "IAG O2"=0, "IAG C2H2"=1, "IAG C2H4"=2, "IAG NH3 200"=3, "IAG NH3 2000"=4, "IAG NH3 3000"=5, "IAG CO 5%"=6, "IAG Propane 2%"=7, "IAG NO 1000"=8, "IAG SO2"=9, "IAG C3H6"=10, "IAG CO2"=11, "IAG CO"=12, "IAG N2O"=13, "IAG N2O 100"=14, "IAG NO2 1000"=15, "IAG NO2 100"=16, "IAG CH4"=17, "IAG Propane"=18, "IAG NO 5000"=19, "Hansi"=20, "IAG MG"=21]}
  in  "Span 10":T4={"Span Inlet Active"=FALSE, "Analysator"="FT-IR", "Konfig Gasflasche"=FALSE, "Gasflasche"=0, "Gasflaschen Nr.:"="", "Ablaufdatum"=timestamp(0 s since 1904-01-01), "Modus"=0, "Komponenten"={"Komponente 1"={"Komponente:"=0, "Konzentration IST"=0.0, "Einheit"=enum."ppm", "Genauigkeit"=0.0}, "Komponente 2"={"Komponente:"=0, "Konzentration IST"=0.0, "Einheit"=enum."ppm", "Genauigkeit"=0.0}, "Komponente 3"={"Komponente:"=0, "Konzentration IST"=0.0, "Einheit"=enum."ppm", "Genauigkeit"=0.0}, "Komponente 4"={"Komponente:"=0, "Konzentration IST"=0.0, "Einheit"=enum."ppm", "Genauigkeit"=0.0}, "Komponente 5"={"Komponente:"=0, "Konzentration IST"=0.0, "Einheit"=enum."ppm", "Genauigkeit"=0.0}}} {"Komponenten"."Komponente 5"."Komponente:" items=["NO (350,3000) LP 191C", "NO2 (150) LP 191C (1of2)", "NO2 (2000) LP 191C (2of2)", "N2O (300) LP 191C (1of2)", "NH3 (300) LP 191C (1of2)", "NH3 (900,3000) LP 191C (2of2)", "HNCO (400) 191C", "H2O% (30) LP 191C", "Formaldehyde (70,500) LP 191C", "CO2 low% (4) LP 191C (2of2)", "CO2% (20) LP 191C (1of2)", "CO (700) LP 191C (1of3)", "CO% (1) LP 191C (2of3)", "Propylene (1000) LP 191C", "Aromatic HC C7 (500) LP 191C", "Ethylene (1000) LP 191C", "CH4 (250) LP 191C (1of2)", "CH4 (5000) LP 191C (2of2)", "Ethane (1000) LP 191C", "Acetylene (1000) LP 191C", "HNO2 (20) 191C", "MeOH (1000) 191C", "CO% (10) LP 191C (3of3)", "Formic Acid (100) 191C", "SO2 (500) LP 191C", "Acetaldehyde (1000) LP 191C", "COS (100) LP 191C", "1,3 butadiene (100) LP 191C", "Oil as Octane (200) LP 191C", "N2O (1000) LP 191C (2of2)", "Propane (200) LP 191C", "NO2 autorange (2000)", "CO autorange (100000)", "CH4 autorange (5000)", "NH3 autorange (3000)", "Temp. Gascell", "Pressure Gascell", "sBeam@2500"]; "Komponenten"."Komponente 5"."Konzentration IST" format="%#.4f"; "Komponenten"."Komponente 5"."Genauigkeit" format="%#.1f"; "Komponenten"."Komponente 4"."Komponente:" items=["NO (350,3000) LP 191C", "NO2 (150) LP 191C (1of2)", "NO2 (2000) LP 191C (2of2)", "N2O (300) LP 191C (1of2)", "NH3 (300) LP 191C (1of2)", "NH3 (900,3000) LP 191C (2of2)", "HNCO (400) 191C", "H2O% (30) LP 191C", "Formaldehyde (70,500) LP 191C", "CO2 low% (4) LP 191C (2of2)", "CO2% (20) LP 191C (1of2)", "CO (700) LP 191C (1of3)", "CO% (1) LP 191C (2of3)", "Propylene (1000) LP 191C", "Aromatic HC C7 (500) LP 191C", "Ethylene (1000) LP 191C", "CH4 (250) LP 191C (1of2)", "CH4 (5000) LP 191C (2of2)", "Ethane (1000) LP 191C", "Acetylene (1000) LP 191C", "HNO2 (20) 191C", "MeOH (1000) 191C", "CO% (10) LP 191C (3of3)", "Formic Acid (100) 191C", "SO2 (500) LP 191C", "Acetaldehyde (1000) LP 191C", "COS (100) LP 191C", "1,3 butadiene (100) LP 191C", "Oil as Octane (200) LP 191C", "N2O (1000) LP 191C (2of2)", "Propane (200) LP 191C", "NO2 autorange (2000)", "CO autorange (100000)", "CH4 autorange (5000)", "NH3 autorange (3000)", "Temp. Gascell", "Pressure Gascell", "sBeam@2500"]; "Komponenten"."Komponente 4"."Konzentration IST" format="%#.4f"; "Komponenten"."Komponente 4"."Genauigkeit" format="%#.1f"; "Komponenten"."Komponente 3"."Komponente:" items=["NO (350,3000) LP 191C", "NO2 (150) LP 191C (1of2)", "NO2 (2000) LP 191C (2of2)", "N2O (300) LP 191C (1of2)", "NH3 (300) LP 191C (1of2)", "NH3 (900,3000) LP 191C (2of2)", "HNCO (400) 191C", "H2O% (30) LP 191C", "Formaldehyde (70,500) LP 191C", "CO2 low% (4) LP 191C (2of2)", "CO2% (20) LP 191C (1of2)", "CO (700) LP 191C (1of3)", "CO% (1) LP 191C (2of3)", "Propylene (1000) LP 191C", "Aromatic HC C7 (500) LP 191C", "Ethylene (1000) LP 191C", "CH4 (250) LP 191C (1of2)", "CH4 (5000) LP 191C (2of2)", "Ethane (1000) LP 191C", "Acetylene (1000) LP 191C", "HNO2 (20) 191C", "MeOH (1000) 191C", "CO% (10) LP 191C (3of3)", "Formic Acid (100) 191C", "SO2 (500) LP 191C", "Acetaldehyde (1000) LP 191C", "COS (100) LP 191C", "1,3 butadiene (100) LP 191C", "Oil as Octane (200) LP 191C", "N2O (1000) LP 191C (2of2)", "Propane (200) LP 191C", "NO2 autorange (2000)", "CO autorange (100000)", "CH4 autorange (5000)", "NH3 autorange (3000)", "Temp. Gascell", "Pressure Gascell", "sBeam@2500"]; "Komponenten"."Komponente 3"."Konzentration IST" format="%#.4f"; "Komponenten"."Komponente 3"."Genauigkeit" format="%#.1f"; "Komponenten"."Komponente 2"."Komponente:" items=["NO (350,3000) LP 191C", "NO2 (150) LP 191C (1of2)", "NO2 (2000) LP 191C (2of2)", "N2O (300) LP 191C (1of2)", "NH3 (300) LP 191C (1of2)", "NH3 (900,3000) LP 191C (2of2)", "HNCO (400) 191C", "H2O% (30) LP 191C", "Formaldehyde (70,500) LP 191C", "CO2 low% (4) LP 191C (2of2)", "CO2% (20) LP 191C (1of2)", "CO (700) LP 191C (1of3)", "CO% (1) LP 191C (2of3)", "Propylene (1000) LP 191C", "Aromatic HC C7 (500) LP 191C", "Ethylene (1000) LP 191C", "CH4 (250) LP 191C (1of2)", "CH4 (5000) LP 191C (2of2)", "Ethane (1000) LP 191C", "Acetylene (1000) LP 191C", "HNO2 (20) 191C", "MeOH (1000) 191C", "CO% (10) LP 191C (3of3)", "Formic Acid (100) 191C", "SO2 (500) LP 191C", "Acetaldehyde (1000) LP 191C", "COS (100) LP 191C", "1,3 butadiene (100) LP 191C", "Oil as Octane (200) LP 191C", "N2O (1000) LP 191C (2of2)", "Propane (200) LP 191C", "NO2 autorange (2000)", "CO autorange (100000)", "CH4 autorange (5000)", "NH3 autorange (3000)", "Temp. Gascell", "Pressure Gascell", "sBeam@2500"]; "Komponenten"."Komponente 2"."Konzentration IST" format="%#.4f"; "Komponenten"."Komponente 2"."Genauigkeit" format="%#.1f"; "Komponenten"."Komponente 1"."Komponente:" items=["NO (350,3000) LP 191C", "NO2 (150) LP 191C (1of2)", "NO2 (2000) LP 191C (2of2)", "N2O (300) LP 191C (1of2)", "NH3 (300) LP 191C (1of2)", "NH3 (900,3000) LP 191C (2of2)", "HNCO (400) 191C", "H2O% (30) LP 191C", "Formaldehyde (70,500) LP 191C", "CO2 low% (4) LP 191C (2of2)", "CO2% (20) LP 191C (1of2)", "CO (700) LP 191C (1of3)", "CO% (1) LP 191C (2of3)", "Propylene (1000) LP 191C", "Aromatic HC C7 (500) LP 191C", "Ethylene (1000) LP 191C", "CH4 (250) LP 191C (1of2)", "CH4 (5000) LP 191C (2of2)", "Ethane (1000) LP 191C", "Acetylene (1000) LP 191C", "HNO2 (20) 191C", "MeOH (1000) 191C", "CO% (10) LP 191C (3of3)", "Formic Acid (100) 191C", "SO2 (500) LP 191C", "Acetaldehyde (1000) LP 191C", "COS (100) LP 191C", "1,3 butadiene (100) LP 191C", "Oil as Octane (200) LP 191C", "N2O (1000) LP 191C (2of2)", "Propane (200) LP 191C", "NO2 autorange (2000)", "CO autorange (100000)", "CH4 autorange (5000)", "NH3 autorange (3000)", "Temp. Gascell", "Pressure Gascell", "sBeam@2500"]; "Komponenten"."Komponente 1"."Konzentration IST" format="%#.4f"; "Komponenten"."Komponente 1"."Genauigkeit" format="%#.1f"; "Modus" items=["CG zu PNS", "CG zu Entnahmestelle"]; "Ablaufdatum" format="%<%d.%m.%Y>T"; "Gasflasche" items=["----"=10000, "IAG O2"=0, "IAG C2H2"=1, "IAG C2H4"=2, "IAG NH3 200"=3, "IAG NH3 2000"=4, "IAG NH3 3000"=5, "IAG CO 5%"=6, "IAG Propane 2%"=7, "IAG NO 1000"=8, "IAG SO2"=9, "IAG C3H6"=10, "IAG CO2"=11, "IAG CO"=12, "IAG N2O"=13, "IAG N2O 100"=14, "IAG NO2 1000"=15, "IAG NO2 100"=16, "IAG CH4"=17, "IAG Propane"=18, "IAG NO 5000"=19, "Hansi"=20, "IAG MG"=21]}
  in  "Tab löschen":bool caption="Test Start"
  out "Anzeigecluster":T11 {"Wert 5" format="%.3g"; "Wert 4" format="%.3g"; "Wert 3" format="%.3g"; "Wert 2" format="%.3g"; "Wert 1" format="%.3g"}
  out "Drifttabelle":T12
  out "Status":string
  in  "Test Start":bool
  in  "Abbrechen":bool
  out "Anzeigecluster 2":T11 {"Wert 5" format="%.3g"; "Wert 4" format="%.3g"; "Wert 3" format="%.3g"; "Wert 2" format="%.3g"; "Wert 1" format="%.3g"}
  out "Drifttabelle 2":T12
  out "Status 2":string caption="Status"
  in  "Test Start 2":bool caption="Test Start"
  in  "Abbrechen 2":bool caption="Abbrechen"
  in  "Print PDF":bool caption="Abbrechen"
  # "Gas Analyzer Drift Verification EPA CRF40 §1065.550"
  # "Allgemeine Einstellungen"
  # "Protokoll Einstellung"
  # "sec."
  # "sec."
  # "Span Einstellungen"
  # "Komponente"
  # "Konzentration"
  # "Einheit"
  # "Genauigkeit [%]"
  # "Komponente"
  # "Konzentration"
  # "Einheit"
  # "Genauigkeit [%]"
  # "Komponente"
  # "Konzentration"
  # "Einheit"
  # "Genauigkeit [%]"
  # "Komponente"
  # "Konzentration"
  # "Einheit"
  # "Genauigkeit [%]"
  # "Komponente"
  # "Konzentration"
  # "Einheit"
  # "Genauigkeit [%]"
  # "Komponente"
  # "Konzentration"
  # "Einheit"
  # "Genauigkeit [%]"
  # "Komponente"
  # "Konzentration"
  # "Einheit"
  # "Genauigkeit [%]"
  # "Komponente"
  # "Konzentration"
  # "Einheit"
  # "Genauigkeit [%]"
  # "Komponente"
  # "Konzentration"
  # "Einheit"
  # "Genauigkeit [%]"
  # "Komponente"
  # "Konzentration"
  # "Einheit"
  # "Genauigkeit [%]"
  # "Komponente"
  # "Aktueller Wert"
  # "Einheit"
  # "x"
  # "x"
  # "x"
  # "x"
  # "x"
  # "x"
  # "Komponente"
  # "Aktueller Wert"
  # "Einheit"
  # "x"
  # "x"
  # "x"
  # "x"
  # "x"
  # "x"
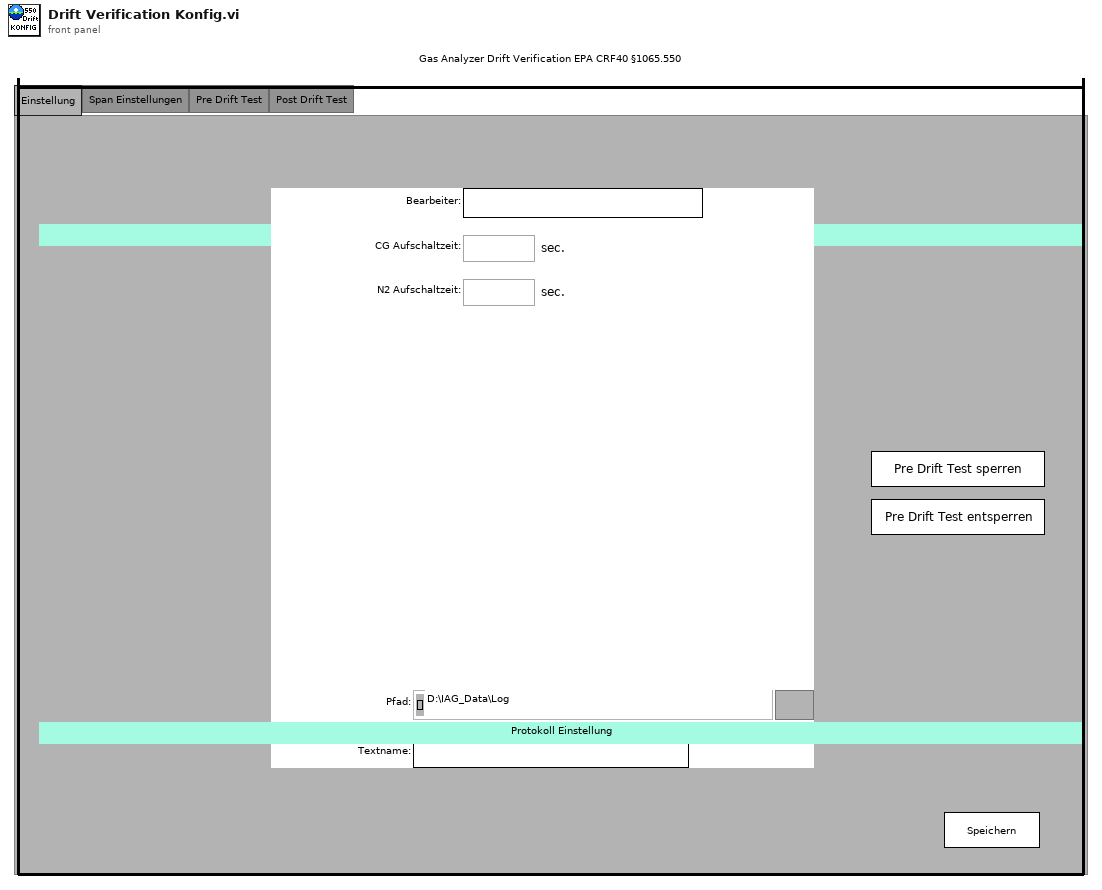
[diagram p1: front panel]
types:
  T1 = enum32{"Settings", "Spaninlet Settings", "Pre Drift Test", "Post Drift Test"}
  T2 = typedef "EPA 1065.lvlib/Gas Analyzer Drift 1065-550.lvlib/Konfig Daten Drift Verification.ctl" = cluster{"Bearbeiter:":string, "Pfad:":path, "Textname:":string, "CG Aufschaltzeit:":dbl, "N2 Aufschaltzeit:":dbl}
  T3 = enum32{"SPAN  1", "SPAN  2", "SPAN  3", "SPAN  4", "SPAN  5", "SPAN  6", "SPAN  7", "SPAN  8", "SPAN  9", "SPAN  10"}
  T4 = typedef "EPA 1065.lvlib/Gas Analyzer Drift 1065-550.lvlib/Spaninlet Cluster.ctl" = cluster{"Span Inlet Active":T5, "Analysator":T6, "Konfig Gasflasche":T5, "Gasflasche":T7, "Gasflaschen Nr.:":string, "Ablaufdatum":timestamp, "Modus":T8, "Komponenten":T9}
  T5 = typedef "System Einstellungen V2.lvlib/Konfig Gasflasche.ctl" = bool
  T6 = typedef "System Einstellungen V2.lvlib/Analysatoren.ctl" = string
  T7 = typedef "System Einstellungen V2.lvlib/Gasflasche Auswahl.ctl" = u16
  T8 = typedef "EPA 1065.lvlib/T90 Test 1065-308.lvlib/Modus.ctl" = u16
  T9 = typedef "EPA 1065.lvlib/Gas Analyzer Drift 1065-550.lvlib/Komponentencluster.ctl" = cluster{"Komponente 1":T10, "Komponente 2":T10, "Komponente 3":T10, "Komponente 4":T10, "Komponente 5":T10}
  T10 = typedef "EPA 1065.lvlib/Gas Analyzer Drift 1065-550.lvlib/Komponentenauswahl.ctl" = cluster{"Komponente:":u16, "Konzentration IST":dbl, "Einheit":enum16{"ppm", "%"}, "Genauigkeit":dbl}
  T11 = typedef "EPA 1065.lvlib/Gas Analyzer Drift 1065-550.lvlib/Anzeigecluster.ctl" = cluster{"Komponente 1":string, "Komponente 2":string, "Komponente 3":string, "Komponente 4":string, "Komponente 5":string, "Wert 1":sgl, "Wert 2":sgl, "Wert 3":sgl, "Wert 4":sgl, "Wert 5":sgl, "Einheit 1":string, "Einheit 2":string, "Einheit 3":string, "Einheit 4":string, "Einheit 5":string}
  T12 = typedef "EPA 1065.lvlib/Gas Analyzer Drift 1065-550.lvlib/Drifttabelle.ctl" = string[][]
  T13 = typedef "EPA 1065.lvlib/Gas Analyzer Drift 1065-550.lvlib/Aktion FGV Drift Daten.ctl" = enum16{"lesen", "Konfig Daten", "PDF einstellen", "laden", "speichern", "Tabelle init", "Zeile Prüfen", "Info schreiben", "Span Einstellung", "Pre Werte schreiben", "Post Werte schreiben", "NB Pre Wert schreiben", "NB Post Wert schreiben", "Tabelle löschen"}
  T14 = enum32{"Page Enabled", "Page Disabled", "Page Disabled & Grayed"}
  T15 = typedef "EPA 1065.lvlib/Gas Analyzer Drift 1065-550.lvlib/Aktion FGV Komponentenreferenz verwalten.ctl" = enum16{"Referenzen init", "lesen", "Referenzen schließen", "Ring beschreiben"}
  T16 = typedef "EPA 1065.lvlib/Gas Analyzer Drift 1065-550.lvlib/Aktion Automatischer Ablauf Zustandsautomat.ctl" = enum16{"init", "leerlauf", "N2 aufschalten", "N2 Aufschaltzeit warten", "N2 aufzeichnen", "CG aufschalten", "CG Aufschaltzeit warten", "CG aufzeichnen", "Span Auswahl ändern", "Test abgeschlossen", "Pre Test aktiv", "Post Test aktiv", "Störungen einlesen", "Störung", "Test anhalten", "Test fortsetzen", "Nachbehandlung init", "Nachbehandeln CG aufschalten", "Nachbehandeln CG warten", "Nachbehandeln CG aufzeichnen", "Abbrechen"}
  T17 = typedef "Sprachverwaltung.lvlib/FGV Aktion Tabelle zerlegen.ctl" = enum16{"laden", "vereinzeln", "speichern"}
  T18 = typedef "FT-IR.lvlib/FGV FT-IR Gasliste Aktionen.ctl" = enum16{"lesen", "Gasliste FT-IR", "Gasliste ausgelesen", "laden", "speichern", "löschen"}
  T19 = typedef "System Einstellungen V2.lvlib/Aktion FGV Gasbottledefinition.ctl" = enum16{"lesen", "schreiben", "löschen", "laden", "speichern", "exportieren", "importieren"}
  T20 = typedef "String - Ausgabefeld.ctl" = string
  T21 = typedef "System Einstellungen V2.lvlib/Gasflasche gesamt.ctl" = cluster{"Gasflasche":T22, "Trägergas":T23, "Komponenten":T24[]}
  T22 = typedef "System Einstellungen V2.lvlib/Gasflasche.ctl" = cluster{"Gasname für die Auswahl":string, "Chargennummer":string, "Ablaufdatum":timestamp}
  T23 = typedef "System Einstellungen V2.lvlib/Traegergas.ctl" = string
  T24 = typedef "System Einstellungen V2.lvlib/Gasflaschenkomponente.ctl" = cluster{"Gasauswahl":string, "Konzentration IST":dbl, "Einheit":string, "Genauigkeit":dbl}
  T25 = typedef "EPA 1065.lvlib/Aktion Wertaenderung Gasliste.ctl" = enum16{"Init", "lesen", "Gasliste geändert", "ARN inaktiv", "LEAK inaktiv", "Interference 366 inaktiv", "T90 inaktiv", "Interference 375 inaktiv", "Chiller inaktiv", "FID O2 inaktiv", "FID Opti inaktiv", "Drift inaktiv", "Pre Test inaktiv", "LinV2 inaktiv", "HovaCAL Interference inaktiv"}
  T26 = typedef "EPA 1065.lvlib/Aktion Test Status.ctl" = enum16{"init", "lesen", "prüfen", "Interference 366", "Interference 375", "Chiller läuft", "Drift läuft", "Pre Test läuft", "FID Optimization läuft", "FID Interference läuft", "HovaCAL Interference", "LinV2"}
  T27 = typedef "Funktionstasten.lvlib/Zustaende.ctl" = enum16{"Standby", "Pause", "Eco", "Messen", "Kalibrieren", "Spülen Filter", "Spülen Leitung", "Umgebungsluft", "0-Gas", "Cal-Gas", "CG zu PNS", "-------------", "Init 1", "Init 2", "Init 3", "Init 4", "Messen vorbereiten", "Messen durchführen", "Exit"}
  T28 = typedef "Funktionstasten.lvlib/Funktionstasten-Aktion.ctl" = enum16{"Initialisieren", "Zustand setzen", "Taste gedrückt", "Fehler speichern", "Lesen", "Manuell", "Remote", "Bitparallel", "Samplepoint", "Zeit Prüfen", "reset Umschalten"}
  T29 = typedef "EPA 1065.lvlib/Aktive Tests Cluster.ctl" = cluster{"ANR läuft":bool, "T90 läuft":bool, "Leak läuft":bool, "Interference 366 läuft":bool, "Interference 375 läuft":bool, "Chiller läuft":bool, "FID Interference läuft":bool, "FID optimization läuft":bool, "Drift läuft":bool, "Pre-test läuft":bool, "HovaCAL Interference läuft":bool, "LinV2 läuft":bool}
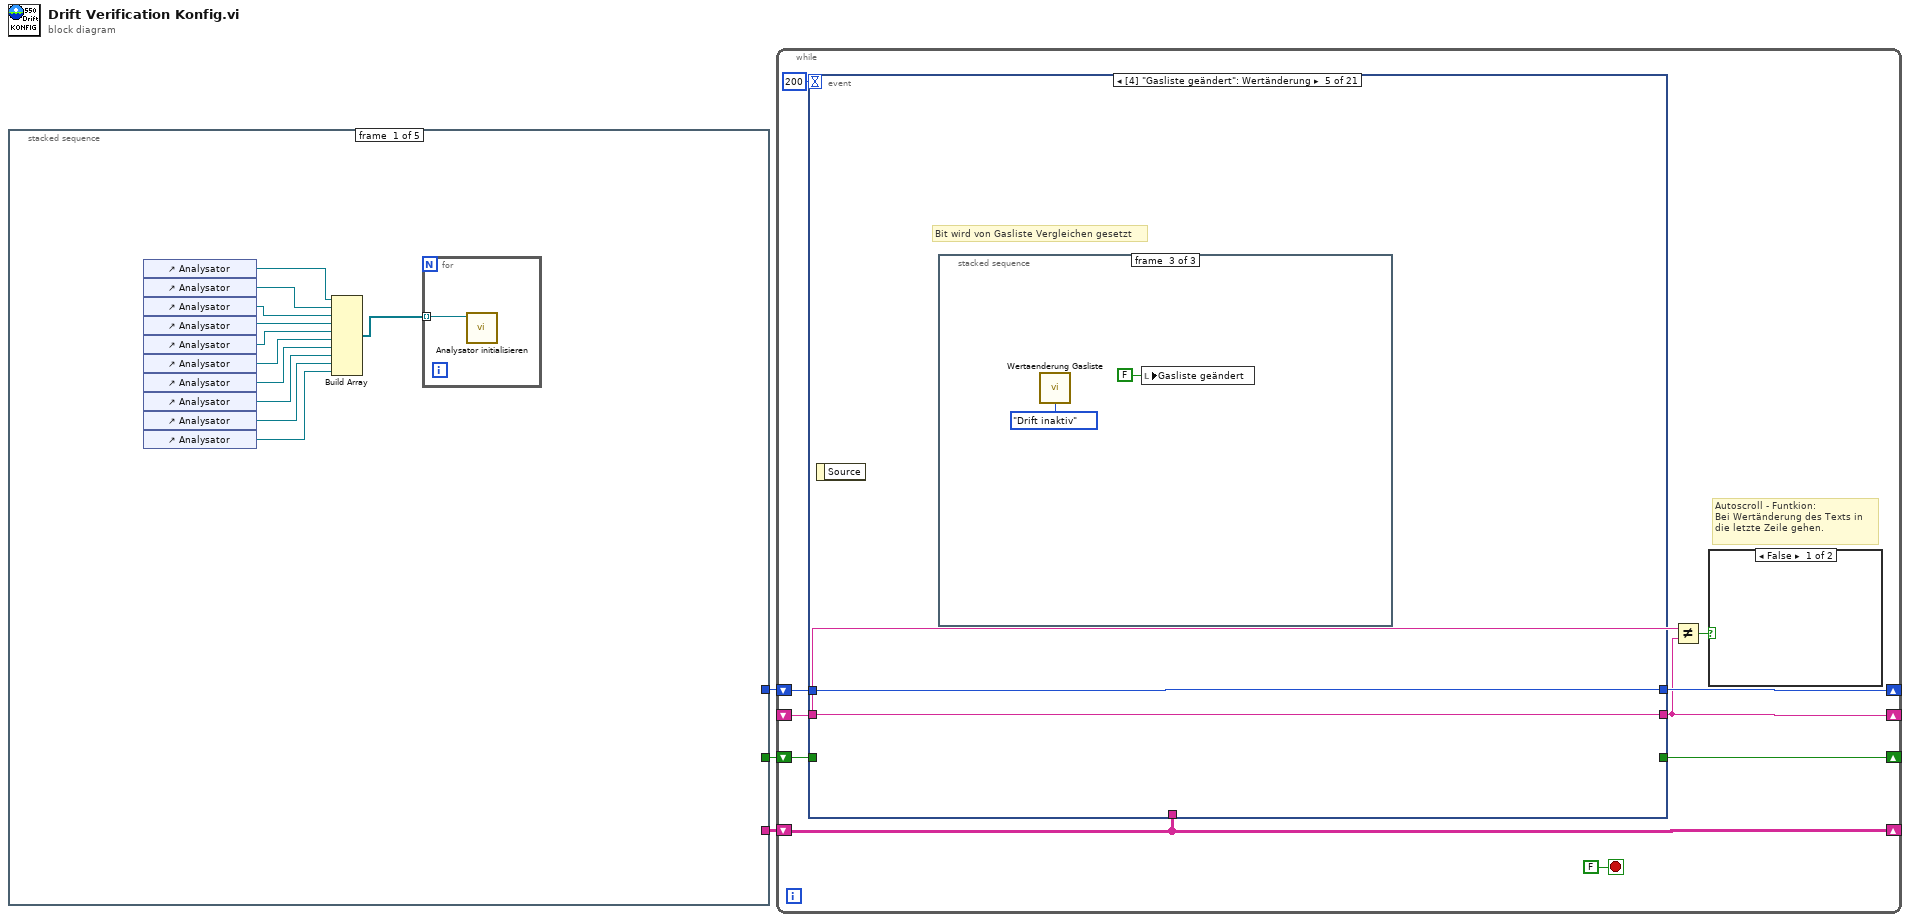
[diagram p0: block diagram]
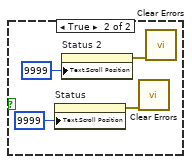
[diagram p2: hidden frame]
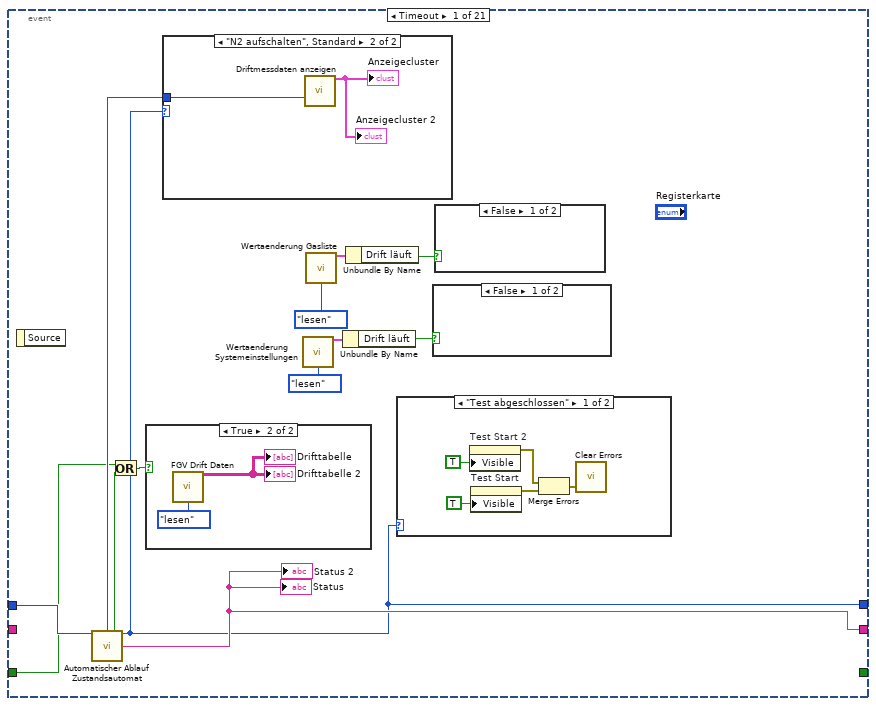
[diagram p3: hidden frame]
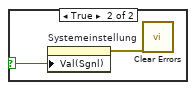
[diagram p5: hidden frame]
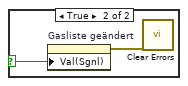
[diagram p8: hidden frame]
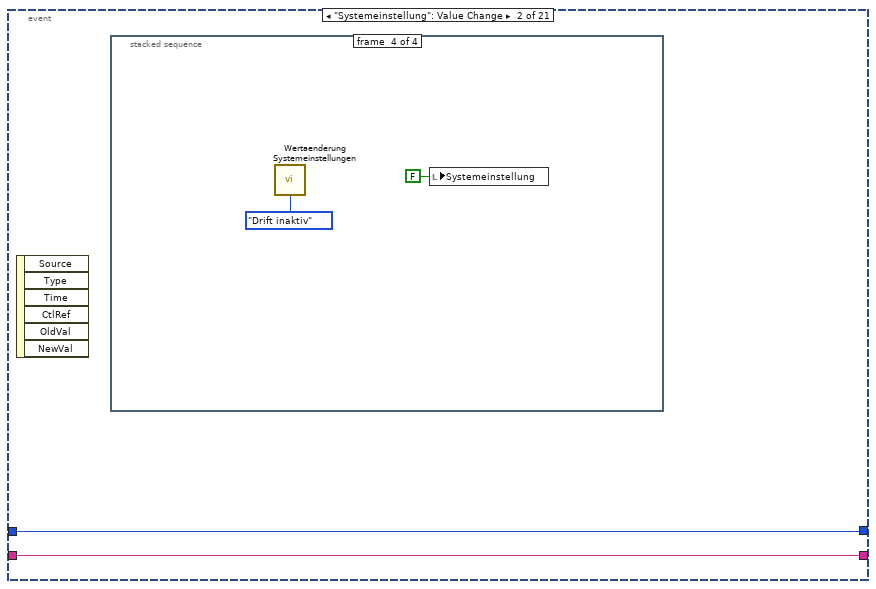
[diagram p9: hidden frame]
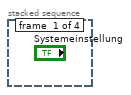
[diagram p10: hidden frame]
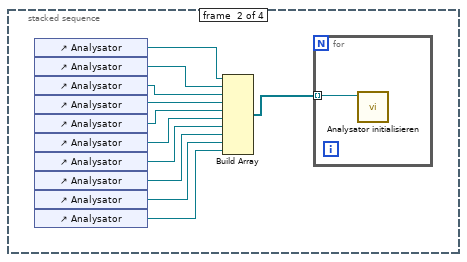
[diagram p11: hidden frame]
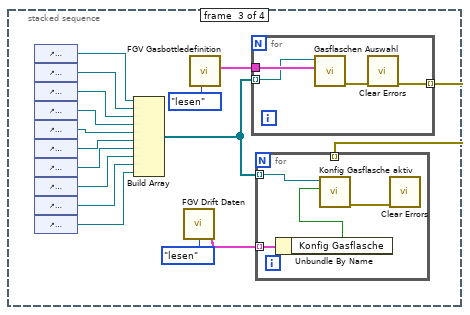
[diagram p12: hidden frame]
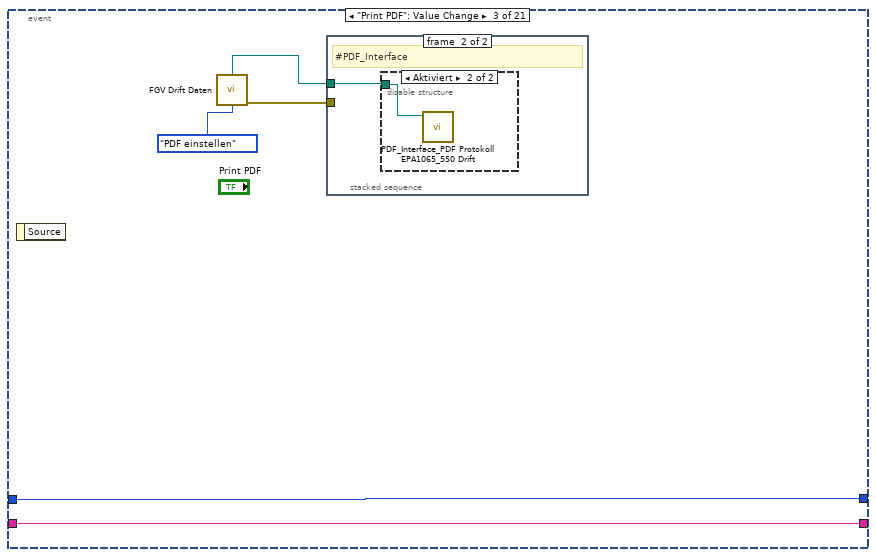
[diagram p13: hidden frame]
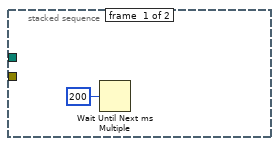
[diagram p14: hidden frame]
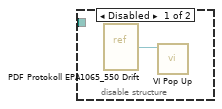
[diagram p15: hidden frame]
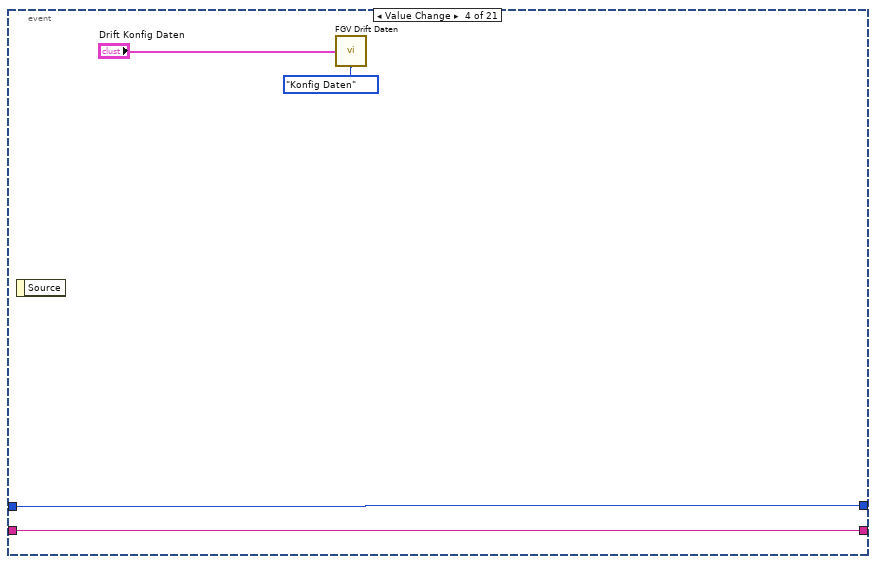
[diagram p16: hidden frame]
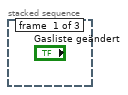
[diagram p17: hidden frame]
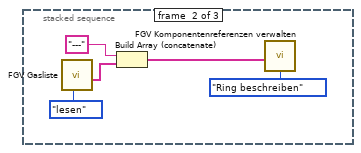
[diagram p18: hidden frame]
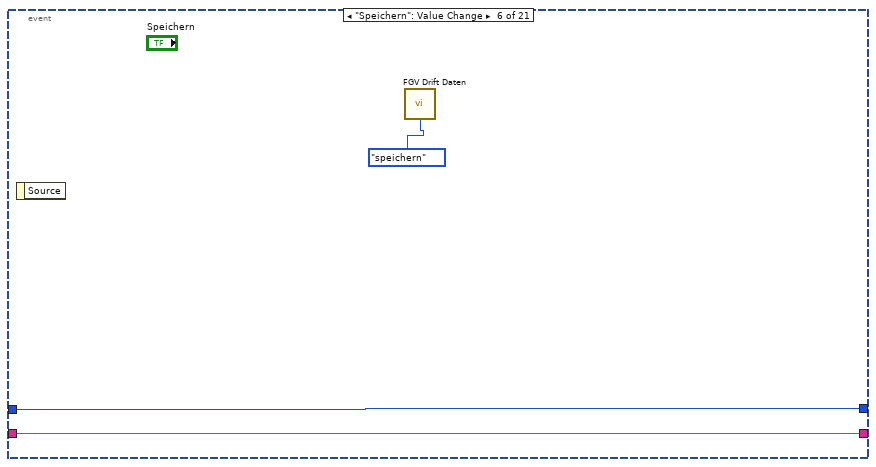
[diagram p19: hidden frame]
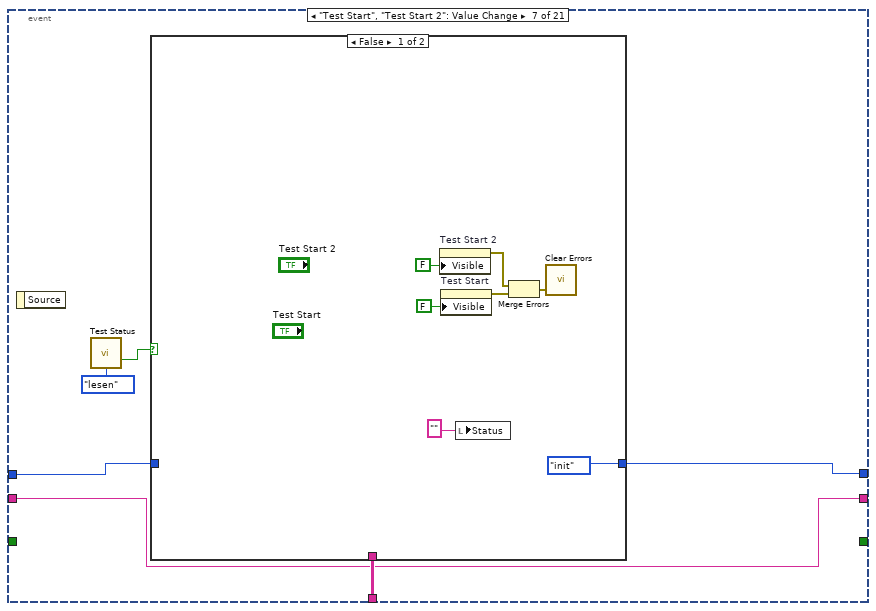
[diagram p20: hidden frame]
diagram:
  n1 = stacked-sequence {
    tunnel: [_ _ _ w110 _] -> w3
    tunnel: [_ _ _ Aktion_Automatischer_Ablauf_Zustandsautomat."leerlauf" ("Aktion") _] -> w2
    tunnel: [_ _ _ _ FALSE] -> w1
    frame #0 {
      n2 = control-ref of="Analysator"() -> (w14:refnum<vi>)
      n3 = control-ref of="Analysator"() -> (w13:refnum<vi>)
      n4 = control-ref of="Analysator"() -> (w12:refnum<vi>)
      n5 = control-ref of="Analysator"() -> (w11:refnum<vi>)
      n6 = control-ref of="Analysator"() -> (w10:refnum<vi>)
      n7 = control-ref of="Analysator"() -> (w9:refnum<vi>)
      n8 = control-ref of="Analysator"() -> (w8:refnum<vi>)
      n9 = control-ref of="Analysator"() -> (w7:refnum<vi>)
      n10 = control-ref of="Analysator"() -> (w6:refnum<vi>)
      n11 = control-ref of="Analysator"() -> (w5:refnum<vi>)
      n12 = Build Array(w14, w13, w12, w11, w10, w9, w8, w7, w6, w5) -> (w4:refnum<vi>[])
      n13 = for {
        tunnel: w4 -> [w15] mode=indexing
        n14 = call "Analysator initialisieren.vi"("Referenz Analysator"=w15) -> ()  [unwired: 9 in, 2 out]
      }
    }
    frame #1 {
      n15 = control-ref of="SpanRegister"() -> (w17:refnum<vi>)
      n16 = call "FGV Drift Daten.vi"("SpanRegister"=w17, "Aktion"=Aktion_FGV_Drift_Daten."Tabelle init") -> ("Drifttabelle"=w34:T12, "error out"=w32:errorcluster)  [unwired: 6 in, 6 out]
      n17 = local write "Drifttabelle 2"(w34) -> ()
      n18 = local write "Drifttabelle"(w34) -> ()
      n19 = call "FGV Drift Daten.vi"("error in (no error)"=w32, "Aktion"=Aktion_FGV_Drift_Daten."laden") -> ("Drift Konfig Daten"=w31:T2, "Spangaseinstellungen"=w28:T4[], "error out"=w29:errorcluster)  [unwired: 6 in, 5 out]
      n20 = property on="Registerkarte" class="RKElem (strikt)"() -> (error out=w36:errorcluster, "Pages"=w40:refnum<vi>[])  [unwired: 2 in, 1 out]
      n21 = local write "Drift Konfig Daten"(w31) -> ()
      n22 = Index Array(array=w40, index=3 ("Index")) -> (element=w38:refnum<vi>)
      n23 = call "FGV Drift Daten.vi"("Spangaseinstellungen"=w28, "error in (no error)"=w29, "Aktion"=Aktion_FGV_Drift_Daten."Span Einstellung") -> ("Spangaseinstellungen"=w16:T4[])  [unwired: 5 in, 7 out]
      n24 = Index Array(array=w16) -> (element #1=w27:T4, element #2=w26:T4, element #3=w25:T4, element #4=w24:T4, element #5=w23:T4, element #6=w22:T4, element #7=w21:T4, element #8=w20:T4, element #9=w19:T4, element #10=w18:T4)  [unwired: 10 in]
      n25 = property class="Seite"(reference=w38, error in=w36, "PageEnb"=T14."Page Disabled & Grayed" ("Aktiv-Status der Seite")) -> (error out=w37:errorcluster)  [unwired: 1 out]
      n26 = local write "Span 10"(w18) -> ()
      n27 = local write "Span 1"(w27) -> ()
      n28 = local write "Span 2"(w26) -> ()
      n29 = local write "Span 3"(w25) -> ()
      n30 = local write "Span 4"(w24) -> ()
      n31 = local write "Span 5"(w23) -> ()
      n32 = local write "Span 6"(w22) -> ()
      n33 = local write "Span 7"(w21) -> ()
      n34 = local write "Span 8"(w20) -> ()
      n35 = local write "Span 9"(w19) -> ()
      n36 = call <vilib>:"Clear Errors.vi"("error in (no error)"=w37) -> ()  [unwired: 5 in, 2 out]
    }
    frame #2 {
      n37 = control-ref of="Komponente:"() -> (w91:refnum<vi>)
      n38 = control-ref of="Komponente:"() -> (w90:refnum<vi>)
      n39 = control-ref of="Komponente:"() -> (w89:refnum<vi>)
      n40 = control-ref of="Komponente:"() -> (w88:refnum<vi>)
      n41 = control-ref of="Komponente:"() -> (w87:refnum<vi>)
      n42 = control-ref of="Komponente:"() -> (w71:refnum<vi>)
      n43 = control-ref of="Komponente:"() -> (w70:refnum<vi>)
      n44 = control-ref of="Komponente:"() -> (w69:refnum<vi>)
      n45 = control-ref of="Komponente:"() -> (w68:refnum<vi>)
      n46 = control-ref of="Komponente:"() -> (w67:refnum<vi>)
      n47 = control-ref of="Komponente:"() -> (w81:refnum<vi>)
      n48 = control-ref of="Komponente:"() -> (w80:refnum<vi>)
      n49 = control-ref of="Komponente:"() -> (w79:refnum<vi>)
      n50 = control-ref of="Komponente:"() -> (w78:refnum<vi>)
      n51 = control-ref of="Komponente:"() -> (w77:refnum<vi>)
      n52 = control-ref of="Komponente:"() -> (w61:refnum<vi>)
      n53 = control-ref of="Komponente:"() -> (w60:refnum<vi>)
      n54 = control-ref of="Komponente:"() -> (w59:refnum<vi>)
      n55 = control-ref of="Komponente:"() -> (w58:refnum<vi>)
      n56 = control-ref of="Komponente:"() -> (w57:refnum<vi>)
      n57 = Build Array(w71, w70, w69, w68, w67) -> (w46:refnum<vi>[])
      n58 = Build Array(w91, w90, w89, w88, w87) -> (w50:refnum<vi>[])
      n59 = Build Array(w81, w80, w79, w78, w77) -> (w48:refnum<vi>[])
      n60 = Build Array(w61, w60, w59, w58, w57) -> (w44:refnum<vi>[])
      n61 = control-ref of="Komponente:"() -> (w86:refnum<vi>)
      n62 = control-ref of="Komponente:"() -> (w85:refnum<vi>)
      n63 = control-ref of="Komponente:"() -> (w84:refnum<vi>)
      n64 = control-ref of="Komponente:"() -> (w83:refnum<vi>)
      n65 = control-ref of="Komponente:"() -> (w82:refnum<vi>)
      n66 = control-ref of="Komponente:"() -> (w66:refnum<vi>)
      n67 = control-ref of="Komponente:"() -> (w65:refnum<vi>)
      n68 = control-ref of="Komponente:"() -> (w64:refnum<vi>)
      n69 = control-ref of="Komponente:"() -> (w63:refnum<vi>)
      n70 = control-ref of="Komponente:"() -> (w62:refnum<vi>)
      n71 = control-ref of="Komponente:"() -> (w76:refnum<vi>)
      n72 = control-ref of="Komponente:"() -> (w75:refnum<vi>)
      n73 = control-ref of="Komponente:"() -> (w74:refnum<vi>)
      n74 = control-ref of="Komponente:"() -> (w73:refnum<vi>)
      n75 = control-ref of="Komponente:"() -> (w72:refnum<vi>)
      n76 = control-ref of="Komponente:"() -> (w56:refnum<vi>)
      n77 = control-ref of="Komponente:"() -> (w55:refnum<vi>)
      n78 = control-ref of="Komponente:"() -> (w54:refnum<vi>)
      n79 = control-ref of="Komponente:"() -> (w53:refnum<vi>)
      n80 = control-ref of="Komponente:"() -> (w52:refnum<vi>)
      n81 = Build Array(w66, w65, w64, w63, w62) -> (w45:refnum<vi>[])
      n82 = Build Array(w56, w55, w54, w53, w52) -> (w43:refnum<vi>[])
      n83 = Build Array(w86, w85, w84, w83, w82) -> (w49:refnum<vi>[])
      n84 = Build Array(w76, w75, w74, w73, w72) -> (w47:refnum<vi>[])
      n85 = Build Array (concatenate)(w50, w49, w48, w47, w46, w45, w44, w43) -> (w42:refnum<vi>[])
      n86 = call "FGV Komponentenreferenzen verwalten.vi"("Referenzen"=w42, "Aktion"=Aktion_FGV_Komponentenreferenz_verwalten."Referenzen init") -> ()  [unwired: 13 in, 1 out]
    }
    frame #3 {
      n87 = for {
        N: 200 -> [_]
        tunnel: [w111] -> w102 mode=indexing
        i -> [w113]
        n88 = Increment(x=w113) -> (x+1=w112:i32)
        n89 = Number To Decimal String(number=w112) -> (decimal integer string=w111:string)  [unwired: 1 in]
      }
      n90 = control-ref of="Dieses VI"() -> (w108:refnum<vi>)
      n91 = call "Automatischer Ablauf Zustandsautomat.vi"("Aktion"=Aktion_Automatischer_Ablauf_Zustandsautomat."Pre Test aktiv") -> ()  [unwired: 10 in, 5 out]
      n92 = property on="Drifttabelle" class="Tbl (strikt)"("Row Headers[]"=w102) -> (error out=w103:errorcluster)  [unwired: 2 in, 1 out]
      n93 = property on="Drifttabelle 2" class="Tbl (strikt)"("Row Headers[]"=w102) -> (error out=w104:errorcluster)  [unwired: 2 in, 1 out]
      n94 = call "in Ursprung setzen.vi"("VI Referenz"=w108) -> ()  [unwired: 10 in, 1 out]
      n95 = invoke class="VI" method="FP.Zentrieren"(reference=w108) -> (error out=w107:errorcluster)  [unwired: 2 in, 2 out]
      n96 = Merge Errors(w103, w104, w107) -> (w109:errorcluster)
      n97 = call "Tabelle in die einzelnen Seiten zerlegen.vi"("Aktion"=FGV_Aktion_Tabelle_zerlegen."vereinzeln", "Index (Seite)"=102) -> ("Sprachliste"=w110:string[][])  [unwired: 7 in, 2 out]
      n98 = property on="Test Start 2" class="Bool."("Visible"=FALSE ("Sichtbar")) -> (error out=w100:errorcluster)  [unwired: 2 in, 1 out]
      n99 = property on="Test Start" class="Bool."("Visible"=TRUE ("Sichtbar")) -> (error out=w97:errorcluster)  [unwired: 2 in, 1 out]
      n100 = call <vilib>:"Clear Errors.vi"("error in (no error)"=w109) -> ()  [unwired: 5 in, 2 out]
      n101 = property on="Test Start 2" class="Bool."("Visible"=TRUE ("Sichtbar")) -> (error out=w95:errorcluster)  [unwired: 2 in, 1 out]
      n102 = Merge Errors(w100, w97) -> (w99:errorcluster)
      n103 = call <vilib>:"Clear Errors.vi"("error in (no error)"=w99) -> ()  [unwired: 5 in, 2 out]
      n104 = call <vilib>:"Clear Errors.vi"("error in (no error)"=w95) -> ()  [unwired: 5 in, 2 out]
    }
    frame #4 {
      # "Anzeigeaktualisieren"
      n105 = call "FGV Gasliste.vi"("Aktionen"=FGV_FT-IR_Gasliste_Aktionen."lesen") -> ("Aktuelle Gasliste gesamt"=w120:T20[])  [unwired: 8 in, 2 out]
      n106 = Build Array (concatenate)("---" ("String"), w120) -> (w118:T20[])
      n107 = control-ref of="Gasflasche"() -> (w133:refnum<vi>)
      n108 = control-ref of="Gasflasche"() -> (w131:refnum<vi>)
      n109 = control-ref of="Gasflasche"() -> (w130:refnum<vi>)
      n110 = control-ref of="Gasflasche"() -> (w129:refnum<vi>)
      n111 = control-ref of="Gasflasche"() -> (w128:refnum<vi>)
      n112 = control-ref of="Gasflasche"() -> (w127:refnum<vi>)
      n113 = control-ref of="Gasflasche"() -> (w126:refnum<vi>)
      n114 = control-ref of="Gasflasche"() -> (w125:refnum<vi>)
      n115 = control-ref of="Gasflasche"() -> (w124:refnum<vi>)
      n116 = control-ref of="Gasflasche"() -> (w123:refnum<vi>)
      n117 = call "FGV Komponentenreferenzen verwalten.vi"("Strings []"=w118, "Aktion"=Aktion_FGV_Komponentenreferenz_verwalten."Ring beschreiben") -> ()  [unwired: 13 in, 1 out]
      n118 = Build Array(w133, w131, w130, w129, w128, w127, w126, w125, w124, w123) -> (w116:refnum<vi>[])
      n119 = call "FGV Drift Daten.vi"("Aktion"=Aktion_FGV_Drift_Daten."lesen") -> ("Spangaseinstellungen"=w117:T4[])  [unwired: 7 in, 7 out]
      n120 = call "FGV Gasbottledefinition.vi"("Aktion"=Aktion_FGV_Gasbottledefinition."lesen") -> ("Gasflaschen Liste gesamt"=w135:T21[])  [unwired: 8 in, 2 out]
      n121 = for {
        tunnel: w135 -> [w143]
        tunnel: w116 -> [w142] mode=indexing
        tunnel: [w141] -> w115 mode=indexing
        n122 = call "Gasflaschen Auswahl.vi"("Gasflaschen Liste gesamt"=w143, "Ring (Eingang)"=w142) -> ("error out"=w140:errorcluster)  [unwired: 9 in]
        n123 = call <vilib>:"Clear Errors.vi"("error in (no error)"=w140) -> ("error out"=w141:errorcluster)  [unwired: 5 in, 1 out]
      }
      n124 = for {
        tunnel: w116 -> [w138] mode=indexing
        tunnel: w117 -> [w137] mode=indexing
        tunnel: w115 -> [_] mode=indexing
        n125 = Unbundle By Name(w137) -> ("Konfig Gasflasche"=w136:T5)
        n126 = call "Konfig Gasflasche aktiv.vi"("Konfig Gasflasche"=w136, "Referenz Gasflasche"=w138) -> ("error out"=w139:errorcluster)  [unwired: 9 in]
        n127 = call <vilib>:"Clear Errors.vi"("error in (no error)"=w139) -> ()  [unwired: 5 in, 2 out]
      }
    }
  }
  n128 = while {
    shift-right: [w151] -> _
    shift-left: w3 -> [w151]
    shift-right: [w149] -> _
    shift-left: w2 -> [w150]
    shift-right: [w147] -> _
    shift-left: _ -> [w146]
    shift-right: [w144] -> _
    shift-left: w1 -> [w145]
    stop <- FALSE stop-if-true
    # "Autoscroll - Funtkion:\nBei Wertänderung des Texts in \ndie letzte Zeile gehen."
    n129 = event shown="[4] \"Gasliste geändert\": Wertänderung" {
      selector: _ -> [_ _ _ _ _ _ _ _ _ _ _ _ _ _ _ _ _ _ _ _ _]
      dyn-events: _ -> [_ _ _ _ _ _ _ _ _ _ _ _ _ _ _ _ _ _ _ _ _]
      timeout: 200 -> [_ _ _ _ _ _ _ _ _ _ _ _ _ _ _ _ _ _ _ _ _]
      tunnel: w151 -> [_ _ _ _ _ _ w252 _ _ _ _ _ _ _ _ _ _ _ _ _ _]
      tunnel: w150 -> [w165 w185 w228 w234 w238 w248 w251 w271 w306 w326 w334 w365 w395 w425 w455 w485 w515 w545 w575 w605 w630]
      tunnel: [w161 w185 w228 w234 w238 w248 w250 w270 w306 w326 w334 w365 w395 w425 w455 w485 w515 w545 w575 w605 w630] -> w149
      tunnel: [w167 w184 w226 w233 w237 w246 w249 w267 w288 w308 w347 w377 w407 w437 w467 w497 w527 w557 w587 w617 w629] -> w147
      tunnel: w146 -> [_ w184 w226 w233 w237 w246 w249 w267 w288 w308 w347 w377 w407 w437 w467 w497 w527 w557 w587 w617 w629]
      tunnel: w145 -> [w158 _ _ _ _ _ _ _ _ _ _ _ _ _ _ _ _ _ _ _ _]
      tunnel: [_ _ _ _ _ _ _ _ _ _ _ _ _ _ _ _ _ _ _ _ TRUE] -> w144
      event Timeout {
        n130 = event-data() -> ()  [unwired: 1 in, 1 out]
        n131 = call "Automatischer Ablauf Zustandsautomat.vi"("Aktion"=w165) -> ("Aktueller test"=w160:i32, "Aktion"=w161:T16, "Anzeige aktualisieren"=w166:bool, "Status"=w167:string)  [unwired: 10 in, 1 out]
        "Status" <- w167
        "Status 2" <- w167
        n132 = Or(x=w158, y=w166) -> (x .or. y?=w159:bool)
        n133 = case shown="True" w159 {
          frame False {
          }
          frame True {
            n134 = call "FGV Drift Daten.vi"("Aktion"=Aktion_FGV_Drift_Daten."lesen") -> ("Drifttabelle"=→"Drifttabelle" →"Drifttabelle 2":T12)  [unwired: 7 in, 7 out]
          }
        }
        n135 = case shown="\"N2 aufschalten\", Standard" w161 {
          tunnel: w160 -> [_ w171]
          frame "leerlauf" {
          }
          frame "N2 aufschalten", Default {
            n136 = call "Driftmessdaten anzeigen.vi"("Spaninlet"=w171) -> ("Anzeigecluster"=→"Anzeigecluster" →"Anzeigecluster 2":T11)  [unwired: 13 in, 1 out]
          }
        }
        n137 = call "Wertaenderung Systemeinstellungen.vi"("Aktion"=Aktion_Wertaenderung_Gasliste."lesen") -> ("Tests"=w163:T29)  [unwired: 13 in, 1 out]
        n138 = call "Wertaenderung Gasliste.vi"("Aktion"=Aktion_Wertaenderung_Gasliste."lesen") -> ("Tests"=w169:T29)  [unwired: 13 in, 1 out]
        n139 = Unbundle By Name(w163) -> ("Drift läuft"=w162:bool)
        n140 = Unbundle By Name(w169) -> ("Drift läuft"=w168:bool)
        n141 = case shown="\"Test abgeschlossen\"" w161 {
          frame "Test abgeschlossen" {
            n142 = property on="Test Start 2" class="Bool."("Visible"=TRUE ("Sichtbar")) -> (error out=w177:errorcluster)  [unwired: 2 in, 1 out]
            n143 = property on="Test Start" class="Bool."("Visible"=TRUE ("Sichtbar")) -> (error out=w180:errorcluster)  [unwired: 2 in, 1 out]
            n144 = Merge Errors(w177, w180) -> (w178:errorcluster)
            n145 = call <vilib>:"Clear Errors.vi"("error in (no error)"=w178) -> ()  [unwired: 5 in, 2 out]
          }
          frame "leerlauf", Default {
          }
        }
        n146 = case shown="False" w162 {
          selector: w162 -> [_ w173]
          frame False {
          }
          frame True {
            n147 = property on="Systemeinstellung" class="Bool. (strikt)"("Val(Sgnl)"=w173) -> (error out=w174:errorcluster)  [unwired: 2 in, 1 out]
            n148 = call <vilib>:"Clear Errors.vi"("error in (no error)"=w174) -> ()  [unwired: 5 in, 2 out]
          }
        }
        n149 = case shown="False" w168 {
          selector: w168 -> [_ w182]
          frame False {
          }
          frame True {
            n150 = property on="Gasliste geändert" class="Bool. (strikt)"("Val(Sgnl)"=w182) -> (error out=w183:errorcluster)  [unwired: 2 in, 1 out]
            n151 = call <vilib>:"Clear Errors.vi"("error in (no error)"=w183) -> ()  [unwired: 5 in, 2 out]
          }
        }
      }
      event "Systemeinstellung": Value Change {
        n152 = event-data() -> ()  [unwired: 1 in, 6 out]
        n153 = stacked-sequence {
          frame #0 {
          }
          frame #1 {
            n154 = control-ref of="Analysator"() -> (w186:refnum<vi>)
            n155 = control-ref of="Analysator"() -> (w187:refnum<vi>)
            n156 = control-ref of="Analysator"() -> (w188:refnum<vi>)
            n157 = control-ref of="Analysator"() -> (w189:refnum<vi>)
            n158 = control-ref of="Analysator"() -> (w190:refnum<vi>)
            n159 = control-ref of="Analysator"() -> (w191:refnum<vi>)
            n160 = control-ref of="Analysator"() -> (w192:refnum<vi>)
            n161 = control-ref of="Analysator"() -> (w193:refnum<vi>)
            n162 = control-ref of="Analysator"() -> (w194:refnum<vi>)
            n163 = control-ref of="Analysator"() -> (w195:refnum<vi>)
            n164 = Build Array(w186, w187, w188, w189, w190, w191, w192, w193, w194, w195) -> (w196:refnum<vi>[])
            n165 = for {
              tunnel: w196 -> [w197] mode=indexing
              n166 = call "Analysator initialisieren.vi"("Referenz Analysator"=w197) -> ()  [unwired: 9 in, 2 out]
            }
          }
          frame #2 {
            n167 = control-ref of="Gasflasche"() -> (w200:refnum<vi>)
            n168 = control-ref of="Gasflasche"() -> (w202:refnum<vi>)
            n169 = control-ref of="Gasflasche"() -> (w203:refnum<vi>)
            n170 = control-ref of="Gasflasche"() -> (w204:refnum<vi>)
            n171 = control-ref of="Gasflasche"() -> (w205:refnum<vi>)
            n172 = control-ref of="Gasflasche"() -> (w206:refnum<vi>)
            n173 = control-ref of="Gasflasche"() -> (w207:refnum<vi>)
            n174 = control-ref of="Gasflasche"() -> (w208:refnum<vi>)
            n175 = control-ref of="Gasflasche"() -> (w209:refnum<vi>)
            n176 = control-ref of="Gasflasche"() -> (w210:refnum<vi>)
            n177 = Build Array(w200, w202, w203, w204, w205, w206, w207, w208, w209, w210) -> (w212:refnum<vi>[])
            n178 = call "FGV Drift Daten.vi"("Aktion"=Aktion_FGV_Drift_Daten."lesen") -> ("Spangaseinstellungen"=w211:T4[])  [unwired: 7 in, 7 out]
            n179 = call "FGV Gasbottledefinition.vi"("Aktion"=Aktion_FGV_Gasbottledefinition."lesen") -> ("Gasflaschen Liste gesamt"=w198:T21[])  [unwired: 8 in, 2 out]
            n180 = for {
              tunnel: w198 -> [w221]
              tunnel: w212 -> [w220] mode=indexing
              tunnel: [w219] -> w213 mode=indexing
              n181 = call "Gasflaschen Auswahl.vi"("Gasflaschen Liste gesamt"=w221, "Ring (Eingang)"=w220) -> ("error out"=w218:errorcluster)  [unwired: 9 in]
              n182 = call <vilib>:"Clear Errors.vi"("error in (no error)"=w218) -> ("error out"=w219:errorcluster)  [unwired: 5 in, 1 out]
            }
            n183 = for {
              tunnel: w212 -> [w216] mode=indexing
              tunnel: w211 -> [w215] mode=indexing
              tunnel: w213 -> [_] mode=indexing
              n184 = Unbundle By Name(w215) -> ("Konfig Gasflasche"=w214:T5)
              n185 = call "Konfig Gasflasche aktiv.vi"("Konfig Gasflasche"=w214, "Referenz Gasflasche"=w216) -> ("error out"=w217:errorcluster)  [unwired: 9 in]
              n186 = call <vilib>:"Clear Errors.vi"("error in (no error)"=w217) -> ()  [unwired: 5 in, 2 out]
            }
          }
          frame #3 {
            n187 = call "Wertaenderung Systemeinstellungen.vi"("Aktion"=Aktion_Wertaenderung_Gasliste."Drift inaktiv") -> ()  [unwired: 13 in, 2 out]
            n188 = local write "Systemeinstellung"(FALSE ("Systemeinstellung")) -> ()
          }
        }
      }
      event "Print PDF": Value Change {
        n189 = event-data() -> ()  [unwired: 1 in, 1 out]
        n190 = call "FGV Drift Daten.vi"("Aktion"=Aktion_FGV_Drift_Daten."PDF einstellen") -> ("PDF Pfad"=w224:path, "error out"=w225:errorcluster)  [unwired: 7 in, 6 out]
        n191 = stacked-sequence {
          tunnel: w225 -> [_ _]
          tunnel: w224 -> [_ w230]
          frame #0 {
            n192 = Wait Until Next ms Multiple(millisecond multiple=u32 200 ("ms")) -> ()  [unwired: 1 out]
          }
          frame #1 {
            # "#PDF_Interface"
            n193 = disable-structure shown="Aktiviert" {
              disable-tunnel: w230 -> [_ w232]
              frame Disabled {
                n194 = vi-ref "PDF Protokoll EPA1065_550 Drift.vi"() -> (w231:refnum<vi>)
                n195 = call "VI Pop Up.vi"("VI Referenz"=w231) -> ()  [unwired: 10 in, 1 out]
              }
              frame Enabled {
                n196 = call "PDF_Interface_PDF Protokoll EPA1065_550 Drift.vi"("Save PDF File Path"=w232) -> ()  [unwired: 10 in, 1 out]
              }
            }
          }
        }
      }
      event Value Change {
        n197 = event-data() -> ()  [unwired: 1 in, 1 out]
        n198 = call "FGV Drift Daten.vi"("Drift Konfig Daten"="Drift Konfig Daten", "Aktion"=Aktion_FGV_Drift_Daten."Konfig Daten") -> ()  [unwired: 6 in, 8 out]
      }
      event "Gasliste geändert": Value Change {
        # "Bit wird von Gasliste Vergleichen gesetzt"
        n199 = event-data() -> ()  [unwired: 1 in, 1 out]
        n200 = stacked-sequence {
          frame #0 {
          }
          frame #1 {
            n201 = call "FGV Gasliste.vi"("Aktionen"=FGV_FT-IR_Gasliste_Aktionen."lesen") -> ("Aktuelle Gasliste gesamt"=w241:T20[])  [unwired: 8 in, 2 out]
            n202 = Build Array (concatenate)("---" ("String"), w241) -> (w243:T20[])
            n203 = call "FGV Komponentenreferenzen verwalten.vi"("Strings []"=w243, "Aktion"=Aktion_FGV_Komponentenreferenz_verwalten."Ring beschreiben") -> ()  [unwired: 13 in, 1 out]
          }
          frame #2 {
            n204 = call "Wertaenderung Gasliste.vi"("Aktion"=Aktion_Wertaenderung_Gasliste."Drift inaktiv") -> ()  [unwired: 13 in, 2 out]
            n205 = local write "Gasliste geändert"(FALSE ("Gasliste geändert")) -> ()
          }
        }
      }
      event "Speichern": Value Change {
        n206 = event-data() -> ()  [unwired: 1 in, 1 out]
        n207 = call "FGV Drift Daten.vi"("Aktion"=Aktion_FGV_Drift_Daten."speichern") -> ()  [unwired: 7 in, 8 out]
      }
      event "Test Start", "Test Start 2": Value Change {
        n208 = event-data() -> ()  [unwired: 1 in, 1 out]
        n209 = call "Test Status.vi"("Aktion"=Aktion_Test_Status."lesen") -> ("Tests sperren"=w253:bool)  [unwired: 11 in, 3 out]
        n210 = case shown="False" w253 {
          tunnel: w252 -> [_ w263]
          tunnel: [Aktion_Automatischer_Ablauf_Zustandsautomat."init" ("Aktion") w262] -> w250
          tunnel: w251 -> [_ w262]
          frame False {
            n211 = property on="Test Start 2" class="Bool."("Visible"=FALSE ("Sichtbar")) -> (error out=w256:errorcluster)  [unwired: 2 in, 1 out]
            n212 = property on="Test Start" class="Bool."("Visible"=FALSE ("Sichtbar")) -> (error out=w259:errorcluster)  [unwired: 2 in, 1 out]
            n213 = local write "Status"("" ("Status")) -> ()
            n214 = Merge Errors(w256, w259) -> (w257:errorcluster)
            n215 = call <vilib>:"Clear Errors.vi"("error in (no error)"=w257) -> ()  [unwired: 5 in, 2 out]
          }
          frame True {
            n216 = call "Texte in VIs uebersetzen.vi"("Sprachliste"=w263, "String zum Übersetzen"="Anderer Test läuft gerade.\nBitte etwas Geduld." ("Nachricht")) -> ("String zum Übersetzen"=w264:string)  [unwired: 9 in, 4 out]
            n217 = One Button Dialog(message=w264, button name ("OK")="OK" ("Schaltflächentext (\"OK\")")) -> ()  [unwired: 1 out]
          }
        }
      }
      event "Abbrechen", "Abbrechen 2": Value Change {
        n218 = event-data() -> ()  [unwired: 1 in, 6 out]
        n219 = call "Test Status.vi"("Aktion"=Aktion_Test_Status."lesen") -> ("Aktive Tests"=w275:T29, "Tests sperren"=w273:bool)  [unwired: 11 in, 2 out]
        n220 = Unbundle By Name(w275) -> ("Drift läuft"=w274:bool)
        n221 = And(x=w274, y=w273) -> (x .and. y?=w272:bool)
        n222 = case shown="True" w272 {
          tunnel: w271 -> [w277 _]
          tunnel: [w277 Aktion_Automatischer_Ablauf_Zustandsautomat."Abbrechen" ("Aktion")] -> w270
          tunnel: "Abbrechen 2" -> [_ w280]
          tunnel: "Abbrechen" -> [_ w279]
          frame False {
          }
          frame True {
            n223 = call "FGV-Funktionstasten.vi"("Herkunft"="Drift Test", "Zustand"=Zustaende."Standby", "Aktion"=Funktionstasten-Aktion."Zustand setzen") -> ()  [unwired: 5 in, 8 out]
            n224 = property on="Test Start 2" class="Bool."("Visible"=w280) -> (error out=w281:errorcluster)  [unwired: 2 in, 1 out]
            n225 = property on="Test Start" class="Bool."("Visible"=w279) -> (error out=w283:errorcluster)  [unwired: 2 in, 1 out]
            n226 = Merge Errors(w281, w283) -> (w282:errorcluster)
            n227 = call <vilib>:"Clear Errors.vi"("error in (no error)"=w282) -> ()  [unwired: 5 in, 2 out]
          }
        }
      }
      event "Pre Drift sperren": Value Change {
        n228 = event-data() -> ()  [unwired: 1 in, 1 out]
        n229 = property on="Registerkarte" class="RKElem (strikt)"() -> (error out=w296:errorcluster, "Pages"=w300:refnum<vi>[])  [unwired: 2 in, 1 out]
        n230 = call "Automatischer Ablauf Zustandsautomat.vi"("Aktion"=Aktion_Automatischer_Ablauf_Zustandsautomat."Post Test aktiv") -> ()  [unwired: 10 in, 5 out]
        n231 = Index Array(array=w300, index #1=2 ("Index"), index #2=3 ("Index")) -> (element #1=w298:refnum<vi>, element #2=w290:refnum<vi>)
        n232 = property class="Seite"(reference=w298, error in=w296, "PageEnb"=T14."Page Disabled & Grayed" ("Aktiv-Status der Seite")) -> (error out=w295:errorcluster)  [unwired: 1 out]
        n233 = property class="Seite"(reference=w290, "PageEnb"=T14."Page Enabled" ("Aktiv-Status der Seite")) -> (error out=w289:errorcluster)  [unwired: 1 in, 1 out]
        n234 = property on="Test Start 2" class="Bool."("Visible"=TRUE ("Sichtbar")) -> (error out=w301:errorcluster)  [unwired: 2 in, 1 out]
        n235 = property on="Test Start" class="Bool."("Visible"=FALSE ("Sichtbar")) -> (error out=w304:errorcluster)  [unwired: 2 in, 1 out]
        n236 = Merge Errors(w301, w304, w295, w289) -> (w302:errorcluster)
        n237 = call <vilib>:"Clear Errors.vi"("error in (no error)"=w302) -> ("error out"=w293:errorcluster)  [unwired: 5 in, 1 out]
        n238 = call "FGV Drift Daten.vi"("error in (no error)"=w293, "Aktion"=Aktion_FGV_Drift_Daten."speichern") -> ()  [unwired: 6 in, 8 out]
      }
      event "Pre Drift entsperren": Value Change {
        n239 = event-data() -> ()  [unwired: 1 in, 1 out]
        n240 = property on="Registerkarte" class="RKElem (strikt)"() -> (error out=w313:errorcluster, "Pages"=w314:refnum<vi>[])  [unwired: 2 in, 1 out]
        n241 = Index Array(array=w314, index #1=2 ("Index"), index #2=3 ("Index")) -> (element #1=w319:refnum<vi>, element #2=w310:refnum<vi>)
        n242 = property on="Test Start 2" class="Bool."("Visible"=FALSE ("Sichtbar")) -> (error out=w321:errorcluster)  [unwired: 2 in, 1 out]
        n243 = property on="Test Start" class="Bool."("Visible"=TRUE ("Sichtbar")) -> (error out=w324:errorcluster)  [unwired: 2 in, 1 out]
        n244 = property class="Seite"(reference=w319, error in=w313, "PageEnb"=T14."Page Enabled" ("Aktiv-Status der Seite")) -> (error out=w317:errorcluster)  [unwired: 1 out]
        n245 = property class="Seite"(reference=w310, "PageEnb"=T14."Page Disabled & Grayed" ("Aktiv-Status der Seite")) -> (error out=w309:errorcluster)  [unwired: 1 in, 1 out]
        n246 = Merge Errors(w321, w324, w317, w309) -> (w322:errorcluster)
        n247 = call "Automatischer Ablauf Zustandsautomat.vi"("Aktion"=Aktion_Automatischer_Ablauf_Zustandsautomat."Pre Test aktiv") -> ()  [unwired: 10 in, 5 out]
        n248 = call <vilib>:"Clear Errors.vi"("error in (no error)"=w322) -> ("error out"=w315:errorcluster)  [unwired: 5 in, 1 out]
        n249 = call "FGV Drift Daten.vi"("error in (no error)"=w315, "Aktion"=Aktion_FGV_Drift_Daten."speichern") -> ()  [unwired: 6 in, 8 out]
      }
      event Value Change {
        n250 = event-data() -> ("OldVal.Komponenten"=w344:T9, "NewVal.Komponenten"=w343:T9, "OldVal.Gasflasche"=w332:T7, "NewVal.Gasflasche"=w331:T7)  [unwired: 1 in]
        n251 = control-ref of="Gasflasche"() -> (w335:refnum<vi>)
        n252 = call "FGV Drift Daten.vi"("Aktion"=Aktion_FGV_Drift_Daten."lesen") -> ("Spangaseinstellungen"=w340:T4[])  [unwired: 7 in, 7 out]
        n253 = Unbundle By Name("Span 1") -> ("Konfig Gasflasche"=w346:T5, "Gasflasche"=w345:T7)
        n254 = Not Equal?(x=w344, y=w343) -> (x != y?=w342:bool)
        n255 = Not Equal?(x=w332, y=w331) -> (x != y?=w329:bool)
        n256 = And(x=w346, y=w329) -> (x .and. y?=w330:T5)
        n257 = call "Konfig Gasflasche aktiv.vi"("Konfig Gasflasche"=w346, "Referenz Gasflasche"=w335) -> ()  [unwired: 9 in, 1 out]
        n258 = case shown="False" w342 {
          tunnel: w330 -> [w351 _]
          tunnel: w345 -> [w350 _]
          tunnel: "Span 1" -> [w349 w356]
          tunnel: [w348 w356] -> w333
          frame False {
            n259 = case shown="True" w351 {
              tunnel: w350 -> [_ w355]
              tunnel: w349 -> [w352 w354]
              tunnel: [w352 w353] -> w348
              frame False {
              }
              frame True {
                n260 = call "Spaneinstellung befuellen.vi"("Gasflasche"=w355, "Span 1"=w354) -> ("Span 1"=w353:T4)  [unwired: 7 in, 2 out]
              }
            }
          }
          frame True {
          }
        }
        n261 = Replace Array Subset(array=w340, new element=w333, index=0 ("Index")) -> (w337:T4[])
        n262 = call "FGV Drift Daten.vi"("Spangaseinstellungen"=w337, "Aktion"=Aktion_FGV_Drift_Daten."Span Einstellung") -> ("error out"=w327:errorcluster)  [unwired: 6 in, 7 out]
        n263 = local write "Span 1"(w333) -> ()
        n264 = call "FGV Drift Daten.vi"("error in (no error)"=w327, "Aktion"=Aktion_FGV_Drift_Daten."speichern") -> ()  [unwired: 6 in, 8 out]
      }
      event Value Change {
        n265 = event-data() -> ("OldVal.Komponenten"=w374:T9, "NewVal.Komponenten"=w364:T9, "OldVal.Gasflasche"=w362:T7, "NewVal.Gasflasche"=w361:T7)  [unwired: 1 in]
        n266 = control-ref of="Gasflasche"() -> (w366:refnum<vi>)
        n267 = call "FGV Drift Daten.vi"("Aktion"=Aktion_FGV_Drift_Daten."lesen") -> ("Spangaseinstellungen"=w371:T4[])  [unwired: 7 in, 7 out]
        n268 = Unbundle By Name("Span 2") -> ("Konfig Gasflasche"=w376:T5, "Gasflasche"=w375:T7)
        n269 = Not Equal?(x=w362, y=w361) -> (x != y?=w359:bool)
        n270 = Not Equal?(x=w374, y=w364) -> (x != y?=w373:bool)
        n271 = And(x=w376, y=w359) -> (x .and. y?=w360:T5)
        n272 = call "Konfig Gasflasche aktiv.vi"("Konfig Gasflasche"=w376, "Referenz Gasflasche"=w366) -> ()  [unwired: 9 in, 1 out]
        n273 = case shown="False" w373 {
          tunnel: w360 -> [w381 _]
          tunnel: w375 -> [w380 _]
          tunnel: "Span 2" -> [w379 w386]
          tunnel: [w378 w386] -> w363
          frame False {
            n274 = case shown="True" w381 {
              tunnel: w380 -> [_ w385]
              tunnel: w379 -> [w382 w384]
              tunnel: [w382 w383] -> w378
              frame False {
              }
              frame True {
                n275 = call "Spaneinstellung befuellen.vi"("Gasflasche"=w385, "Span 1"=w384) -> ("Span 1"=w383:T4)  [unwired: 7 in, 2 out]
              }
            }
          }
          frame True {
          }
        }
        n276 = Replace Array Subset(array=w371, new element=w363, index=1 ("Index")) -> (w368:T4[])
        n277 = call "FGV Drift Daten.vi"("Spangaseinstellungen"=w368, "Aktion"=Aktion_FGV_Drift_Daten."Span Einstellung") -> ("error out"=w357:errorcluster)  [unwired: 6 in, 7 out]
        n278 = local write "Span 2"(w363) -> ()
        n279 = call "FGV Drift Daten.vi"("error in (no error)"=w357, "Aktion"=Aktion_FGV_Drift_Daten."speichern") -> ()  [unwired: 6 in, 8 out]
      }
      event Value Change {
        n280 = event-data() -> ("OldVal.Komponenten"=w404:T9, "NewVal.Komponenten"=w394:T9, "OldVal.Gasflasche"=w392:T7, "NewVal.Gasflasche"=w391:T7)  [unwired: 1 in]
        n281 = control-ref of="Gasflasche"() -> (w396:refnum<vi>)
        n282 = call "FGV Drift Daten.vi"("Aktion"=Aktion_FGV_Drift_Daten."lesen") -> ("Spangaseinstellungen"=w401:T4[])  [unwired: 7 in, 7 out]
        n283 = Unbundle By Name("Span 3") -> ("Konfig Gasflasche"=w406:T5, "Gasflasche"=w405:T7)
        n284 = Not Equal?(x=w392, y=w391) -> (x != y?=w389:bool)
        n285 = Not Equal?(x=w404, y=w394) -> (x != y?=w403:bool)
        n286 = call "Konfig Gasflasche aktiv.vi"("Konfig Gasflasche"=w406, "Referenz Gasflasche"=w396) -> ()  [unwired: 9 in, 1 out]
        n287 = And(x=w406, y=w389) -> (x .and. y?=w390:T5)
        n288 = case shown="False" w403 {
          tunnel: w390 -> [w411 _]
          tunnel: w405 -> [w410 _]
          tunnel: "Span 3" -> [w409 w416]
          tunnel: [w408 w416] -> w393
          frame False {
            n289 = case shown="True" w411 {
              tunnel: w410 -> [_ w415]
              tunnel: w409 -> [w412 w414]
              tunnel: [w412 w413] -> w408
              frame False {
              }
              frame True {
                n290 = call "Spaneinstellung befuellen.vi"("Gasflasche"=w415, "Span 1"=w414) -> ("Span 1"=w413:T4)  [unwired: 7 in, 2 out]
              }
            }
          }
          frame True {
          }
        }
        n291 = Replace Array Subset(array=w401, new element=w393, index=2 ("Index")) -> (w398:T4[])
        n292 = call "FGV Drift Daten.vi"("Spangaseinstellungen"=w398, "Aktion"=Aktion_FGV_Drift_Daten."Span Einstellung") -> ("error out"=w387:errorcluster)  [unwired: 6 in, 7 out]
        n293 = local write "Span 3"(w393) -> ()
        n294 = call "FGV Drift Daten.vi"("error in (no error)"=w387, "Aktion"=Aktion_FGV_Drift_Daten."speichern") -> ()  [unwired: 6 in, 8 out]
      }
      event Value Change {
        n295 = event-data() -> ("OldVal.Komponenten"=w434:T9, "NewVal.Komponenten"=w424:T9, "OldVal.Gasflasche"=w422:T7, "NewVal.Gasflasche"=w421:T7)  [unwired: 1 in]
        n296 = control-ref of="Gasflasche"() -> (w426:refnum<vi>)
        n297 = call "FGV Drift Daten.vi"("Aktion"=Aktion_FGV_Drift_Daten."lesen") -> ("Spangaseinstellungen"=w431:T4[])  [unwired: 7 in, 7 out]
        n298 = Unbundle By Name("Span 4") -> ("Konfig Gasflasche"=w436:T5, "Gasflasche"=w435:T7)
        n299 = Not Equal?(x=w434, y=w424) -> (x != y?=w433:bool)
        n300 = Not Equal?(x=w422, y=w421) -> (x != y?=w419:bool)
        n301 = And(x=w436, y=w419) -> (x .and. y?=w420:T5)
        n302 = call "Konfig Gasflasche aktiv.vi"("Konfig Gasflasche"=w436, "Referenz Gasflasche"=w426) -> ()  [unwired: 9 in, 1 out]
        n303 = case shown="False" w433 {
          tunnel: w420 -> [w441 _]
          tunnel: w435 -> [w440 _]
          tunnel: "Span 4" -> [w439 w446]
          tunnel: [w438 w446] -> w423
          frame False {
            n304 = case shown="True" w441 {
              tunnel: w440 -> [_ w445]
              tunnel: w439 -> [w442 w444]
              tunnel: [w442 w443] -> w438
              frame False {
              }
              frame True {
                n305 = call "Spaneinstellung befuellen.vi"("Gasflasche"=w445, "Span 1"=w444) -> ("Span 1"=w443:T4)  [unwired: 7 in, 2 out]
              }
            }
          }
          frame True {
          }
        }
        n306 = Replace Array Subset(array=w431, new element=w423, index=3 ("Index")) -> (w428:T4[])
        n307 = call "FGV Drift Daten.vi"("Spangaseinstellungen"=w428, "Aktion"=Aktion_FGV_Drift_Daten."Span Einstellung") -> ("error out"=w417:errorcluster)  [unwired: 6 in, 7 out]
        n308 = call "FGV Drift Daten.vi"("error in (no error)"=w417, "Aktion"=Aktion_FGV_Drift_Daten."speichern") -> ()  [unwired: 6 in, 8 out]
        n309 = local write "Span 4"(w423) -> ()
      }
      event Value Change {
        n310 = event-data() -> ("OldVal.Komponenten"=w464:T9, "NewVal.Komponenten"=w454:T9, "OldVal.Gasflasche"=w452:T7, "NewVal.Gasflasche"=w451:T7)  [unwired: 1 in]
        n311 = call "FGV Drift Daten.vi"("Aktion"=Aktion_FGV_Drift_Daten."lesen") -> ("Spangaseinstellungen"=w461:T4[])  [unwired: 7 in, 7 out]
        n312 = Unbundle By Name("Span 5") -> ("Konfig Gasflasche"=w466:T5, "Gasflasche"=w465:T7)
        n313 = control-ref of="Gasflasche"() -> (w456:refnum<vi>)
        n314 = Not Equal?(x=w464, y=w454) -> (x != y?=w463:bool)
        n315 = Not Equal?(x=w452, y=w451) -> (x != y?=w449:bool)
        n316 = And(x=w466, y=w449) -> (x .and. y?=w450:T5)
        n317 = call "Konfig Gasflasche aktiv.vi"("Konfig Gasflasche"=w466, "Referenz Gasflasche"=w456) -> ()  [unwired: 9 in, 1 out]
        n318 = case shown="False" w463 {
          tunnel: w450 -> [w471 _]
          tunnel: w465 -> [w470 _]
          tunnel: "Span 5" -> [w469 w476]
          tunnel: [w468 w476] -> w453
          frame False {
            n319 = case shown="True" w471 {
              tunnel: w470 -> [_ w475]
              tunnel: w469 -> [w472 w474]
              tunnel: [w472 w473] -> w468
              frame False {
              }
              frame True {
                n320 = call "Spaneinstellung befuellen.vi"("Gasflasche"=w475, "Span 1"=w474) -> ("Span 1"=w473:T4)  [unwired: 7 in, 2 out]
              }
            }
          }
          frame True {
          }
        }
        n321 = Replace Array Subset(array=w461, new element=w453, index=4 ("Index")) -> (w458:T4[])
        n322 = call "FGV Drift Daten.vi"("Spangaseinstellungen"=w458, "Aktion"=Aktion_FGV_Drift_Daten."Span Einstellung") -> ("error out"=w447:errorcluster)  [unwired: 6 in, 7 out]
        n323 = call "FGV Drift Daten.vi"("error in (no error)"=w447, "Aktion"=Aktion_FGV_Drift_Daten."speichern") -> ()  [unwired: 6 in, 8 out]
        n324 = local write "Span 5"(w453) -> ()
      }
      event Value Change {
        n325 = event-data() -> ("OldVal.Komponenten"=w494:T9, "NewVal.Komponenten"=w484:T9, "OldVal.Gasflasche"=w482:T7, "NewVal.Gasflasche"=w481:T7)  [unwired: 1 in]
        n326 = call "FGV Drift Daten.vi"("Aktion"=Aktion_FGV_Drift_Daten."lesen") -> ("Spangaseinstellungen"=w491:T4[])  [unwired: 7 in, 7 out]
        n327 = Unbundle By Name("Span 6") -> ("Konfig Gasflasche"=w496:T5, "Gasflasche"=w495:T7)
        n328 = control-ref of="Gasflasche"() -> (w486:refnum<vi>)
        n329 = Not Equal?(x=w494, y=w484) -> (x != y?=w493:bool)
        n330 = Not Equal?(x=w482, y=w481) -> (x != y?=w479:bool)
        n331 = And(x=w496, y=w479) -> (x .and. y?=w480:T5)
        n332 = call "Konfig Gasflasche aktiv.vi"("Konfig Gasflasche"=w496, "Referenz Gasflasche"=w486) -> ()  [unwired: 9 in, 1 out]
        n333 = case shown="False" w493 {
          tunnel: w480 -> [w501 _]
          tunnel: w495 -> [w500 _]
          tunnel: "Span 6" -> [w499 w506]
          tunnel: [w498 w506] -> w483
          frame False {
            n334 = case shown="True" w501 {
              tunnel: w500 -> [_ w505]
              tunnel: w499 -> [w502 w504]
              tunnel: [w502 w503] -> w498
              frame False {
              }
              frame True {
                n335 = call "Spaneinstellung befuellen.vi"("Gasflasche"=w505, "Span 1"=w504) -> ("Span 1"=w503:T4)  [unwired: 7 in, 2 out]
              }
            }
          }
          frame True {
          }
        }
        n336 = Replace Array Subset(array=w491, new element=w483, index=5 ("Index")) -> (w488:T4[])
        n337 = call "FGV Drift Daten.vi"("Spangaseinstellungen"=w488, "Aktion"=Aktion_FGV_Drift_Daten."Span Einstellung") -> ("error out"=w477:errorcluster)  [unwired: 6 in, 7 out]
        n338 = call "FGV Drift Daten.vi"("error in (no error)"=w477, "Aktion"=Aktion_FGV_Drift_Daten."speichern") -> ()  [unwired: 6 in, 8 out]
        n339 = local write "Span 6"(w483) -> ()
      }
      event Value Change {
        n340 = event-data() -> ("OldVal.Komponenten"=w524:T9, "NewVal.Komponenten"=w514:T9, "OldVal.Gasflasche"=w512:T7, "NewVal.Gasflasche"=w511:T7)  [unwired: 1 in]
        n341 = call "FGV Drift Daten.vi"("Aktion"=Aktion_FGV_Drift_Daten."lesen") -> ("Spangaseinstellungen"=w521:T4[])  [unwired: 7 in, 7 out]
        n342 = Unbundle By Name("Span 7") -> ("Konfig Gasflasche"=w526:T5, "Gasflasche"=w525:T7)
        n343 = control-ref of="Gasflasche"() -> (w516:refnum<vi>)
        n344 = Not Equal?(x=w524, y=w514) -> (x != y?=w523:bool)
        n345 = Not Equal?(x=w512, y=w511) -> (x != y?=w509:bool)
        n346 = And(x=w526, y=w509) -> (x .and. y?=w510:T5)
        n347 = call "Konfig Gasflasche aktiv.vi"("Konfig Gasflasche"=w526, "Referenz Gasflasche"=w516) -> ()  [unwired: 9 in, 1 out]
        n348 = case shown="False" w523 {
          tunnel: w510 -> [w531 _]
          tunnel: w525 -> [w530 _]
          tunnel: "Span 7" -> [w529 w536]
          tunnel: [w528 w536] -> w513
          frame False {
            n349 = case shown="True" w531 {
              tunnel: w530 -> [_ w535]
              tunnel: w529 -> [w532 w534]
              tunnel: [w532 w533] -> w528
              frame False {
              }
              frame True {
                n350 = call "Spaneinstellung befuellen.vi"("Gasflasche"=w535, "Span 1"=w534) -> ("Span 1"=w533:T4)  [unwired: 7 in, 2 out]
              }
            }
          }
          frame True {
          }
        }
        n351 = Replace Array Subset(array=w521, new element=w513, index=6 ("Index")) -> (w518:T4[])
        n352 = call "FGV Drift Daten.vi"("Spangaseinstellungen"=w518, "Aktion"=Aktion_FGV_Drift_Daten."Span Einstellung") -> ("error out"=w507:errorcluster)  [unwired: 6 in, 7 out]
        n353 = local write "Span 7"(w513) -> ()
        n354 = call "FGV Drift Daten.vi"("error in (no error)"=w507, "Aktion"=Aktion_FGV_Drift_Daten."speichern") -> ()  [unwired: 6 in, 8 out]
      }
      event Value Change {
        n355 = event-data() -> ("OldVal.Komponenten"=w554:T9, "NewVal.Komponenten"=w544:T9, "OldVal.Gasflasche"=w542:T7, "NewVal.Gasflasche"=w541:T7)  [unwired: 1 in]
        n356 = call "FGV Drift Daten.vi"("Aktion"=Aktion_FGV_Drift_Daten."lesen") -> ("Spangaseinstellungen"=w551:T4[])  [unwired: 7 in, 7 out]
        n357 = Unbundle By Name("Span 8") -> ("Konfig Gasflasche"=w556:T5, "Gasflasche"=w555:T7)
        n358 = control-ref of="Gasflasche"() -> (w546:refnum<vi>)
        n359 = Not Equal?(x=w542, y=w541) -> (x != y?=w539:bool)
        n360 = Not Equal?(x=w554, y=w544) -> (x != y?=w553:bool)
        n361 = And(x=w556, y=w539) -> (x .and. y?=w540:T5)
        n362 = call "Konfig Gasflasche aktiv.vi"("Konfig Gasflasche"=w556, "Referenz Gasflasche"=w546) -> ()  [unwired: 9 in, 1 out]
        n363 = case shown="False" w553 {
          tunnel: w540 -> [w561 _]
          tunnel: w555 -> [w560 _]
          tunnel: "Span 8" -> [w559 w566]
          tunnel: [w558 w566] -> w543
          frame False {
            n364 = case shown="True" w561 {
              tunnel: w560 -> [_ w565]
              tunnel: w559 -> [w562 w564]
              tunnel: [w562 w563] -> w558
              frame False {
              }
              frame True {
                n365 = call "Spaneinstellung befuellen.vi"("Gasflasche"=w565, "Span 1"=w564) -> ("Span 1"=w563:T4)  [unwired: 7 in, 2 out]
              }
            }
          }
          frame True {
          }
        }
        n366 = Replace Array Subset(array=w551, new element=w543, index=7 ("Index")) -> (w548:T4[])
        n367 = call "FGV Drift Daten.vi"("Spangaseinstellungen"=w548, "Aktion"=Aktion_FGV_Drift_Daten."Span Einstellung") -> ("error out"=w537:errorcluster)  [unwired: 6 in, 7 out]
        n368 = local write "Span 8"(w543) -> ()
        n369 = call "FGV Drift Daten.vi"("error in (no error)"=w537, "Aktion"=Aktion_FGV_Drift_Daten."speichern") -> ()  [unwired: 6 in, 8 out]
      }
      event Value Change {
        n370 = event-data() -> ("OldVal.Komponenten"=w584:T9, "NewVal.Komponenten"=w574:T9, "OldVal.Gasflasche"=w572:T7, "NewVal.Gasflasche"=w571:T7)  [unwired: 1 in]
        n371 = call "FGV Drift Daten.vi"("Aktion"=Aktion_FGV_Drift_Daten."lesen") -> ("Spangaseinstellungen"=w581:T4[])  [unwired: 7 in, 7 out]
        n372 = Unbundle By Name("Span 9") -> ("Konfig Gasflasche"=w586:T5, "Gasflasche"=w585:T7)
        n373 = control-ref of="Gasflasche"() -> (w576:refnum<vi>)
        n374 = Not Equal?(x=w584, y=w574) -> (x != y?=w583:bool)
        n375 = Not Equal?(x=w572, y=w571) -> (x != y?=w569:bool)
        n376 = And(x=w586, y=w569) -> (x .and. y?=w570:T5)
        n377 = call "Konfig Gasflasche aktiv.vi"("Konfig Gasflasche"=w586, "Referenz Gasflasche"=w576) -> ()  [unwired: 9 in, 1 out]
        n378 = case shown="False" w583 {
          tunnel: w570 -> [w591 _]
          tunnel: w585 -> [w590 _]
          tunnel: "Span 9" -> [w589 w596]
          tunnel: [w588 w596] -> w573
          frame False {
            n379 = case shown="True" w591 {
              tunnel: w590 -> [_ w595]
              tunnel: w589 -> [w592 w594]
              tunnel: [w592 w593] -> w588
              frame False {
              }
              frame True {
                n380 = call "Spaneinstellung befuellen.vi"("Gasflasche"=w595, "Span 1"=w594) -> ("Span 1"=w593:T4)  [unwired: 7 in, 2 out]
              }
            }
          }
          frame True {
          }
        }
        n381 = Replace Array Subset(array=w581, new element=w573, index=8 ("Index")) -> (w578:T4[])
        n382 = call "FGV Drift Daten.vi"("Spangaseinstellungen"=w578, "Aktion"=Aktion_FGV_Drift_Daten."Span Einstellung") -> ("error out"=w567:errorcluster)  [unwired: 6 in, 7 out]
        n383 = local write "Span 9"(w573) -> ()
        n384 = call "FGV Drift Daten.vi"("error in (no error)"=w567, "Aktion"=Aktion_FGV_Drift_Daten."speichern") -> ()  [unwired: 6 in, 8 out]
      }
      event Value Change {
        n385 = event-data() -> ("OldVal.Komponenten"=w614:T9, "NewVal.Komponenten"=w604:T9, "OldVal.Gasflasche"=w602:T7, "NewVal.Gasflasche"=w601:T7)  [unwired: 1 in]
        n386 = call "FGV Drift Daten.vi"("Aktion"=Aktion_FGV_Drift_Daten."lesen") -> ("Spangaseinstellungen"=w611:T4[])  [unwired: 7 in, 7 out]
        n387 = Unbundle By Name("Span 10") -> ("Konfig Gasflasche"=w616:T5, "Gasflasche"=w615:T7)
        n388 = control-ref of="Gasflasche"() -> (w606:refnum<vi>)
        n389 = Not Equal?(x=w614, y=w604) -> (x != y?=w613:bool)
        n390 = Not Equal?(x=w602, y=w601) -> (x != y?=w599:bool)
        n391 = And(x=w616, y=w599) -> (x .and. y?=w600:T5)
        n392 = call "Konfig Gasflasche aktiv.vi"("Konfig Gasflasche"=w616, "Referenz Gasflasche"=w606) -> ()  [unwired: 9 in, 1 out]
        n393 = case shown="False" w613 {
          tunnel: w600 -> [w621 _]
          tunnel: w615 -> [w620 _]
          tunnel: "Span 10" -> [w619 w626]
          tunnel: [w618 w626] -> w603
          frame False {
            n394 = case shown="True" w621 {
              tunnel: w620 -> [_ w625]
              tunnel: w619 -> [w622 w624]
              tunnel: [w622 w623] -> w618
              frame False {
              }
              frame True {
                n395 = call "Spaneinstellung befuellen.vi"("Gasflasche"=w625, "Span 1"=w624) -> ("Span 1"=w623:T4)  [unwired: 7 in, 2 out]
              }
            }
          }
          frame True {
          }
        }
        n396 = Replace Array Subset(array=w611, new element=w603, index=9 ("Index")) -> (w608:T4[])
        n397 = call "FGV Drift Daten.vi"("Spangaseinstellungen"=w608, "Aktion"=Aktion_FGV_Drift_Daten."Span Einstellung") -> ("error out"=w597:errorcluster)  [unwired: 6 in, 7 out]
        n398 = call "FGV Drift Daten.vi"("error in (no error)"=w597, "Aktion"=Aktion_FGV_Drift_Daten."speichern") -> ()  [unwired: 6 in, 8 out]
        n399 = local write "Span 10"(w603) -> ()
      }
      event "Tab löschen": Value Change {
        n400 = event-data() -> ()  [unwired: 1 in, 1 out]
        n401 = call "FGV Drift Daten.vi"("Aktion"=Aktion_FGV_Drift_Daten."Tabelle löschen") -> ()  [unwired: 7 in, 8 out]
      }
    }
    n402 = Not Equal?(x=w146, y=w147) -> (x != y?=w148:bool)
    n403 = case shown="False" w148 {
      frame False {
      }
      frame True {
        n404 = property on="Status" class="Str"("Text.Scroll Position"=u32 9999 ("Text.Anzeigeposition")) -> (error out=w157:errorcluster)  [unwired: 2 in, 1 out]
        n405 = property on="Status 2" class="Str"("Text.Scroll Position"=u32 9999 ("Text.Anzeigeposition")) -> (error out=w154:errorcluster)  [unwired: 2 in, 1 out]
        n406 = call <vilib>:"Clear Errors.vi"("error in (no error)"=w157) -> ()  [unwired: 5 in, 2 out]
        n407 = call <vilib>:"Clear Errors.vi"("error in (no error)"=w154) -> ()  [unwired: 5 in, 2 out]
      }
    }
  }
